vi "MC_8_16_12b_JW.vi"() -> ()   [LabVIEW 2011]
uses:
  <vilib>/Utility/file.llb/Read From Spreadsheet File (string).vi
  <vilib>/Utility/inputDevices.llb/keyboardAcquire.vi
  <vilib>/Utility/file.llb/Write To Spreadsheet File (DBL).vi
  <vilib>/Utility/file.llb/Write To Spreadsheet File (string).vi
  <vilib>/regexp/Match Regular Expression.xnode
panel:
  out "X Axis Display Type":string
  out "Opj X Axis":string
  in  "Room Temp":dbl=294.0
  out "No Image 2":path=path "\\\\acad1\\physics/Jurchescu-group/JW-PD/Image Not Found.png"
  out "Save1 Array":string[][](array[string])
  out "Lin Vd":dbl
  out "Lin-Vg Array-Used":dbl[](array[numeric])
  out "Lin Id-Used":dbl[](array[numeric])
  out "Comments":string
  out "Folder Index":dbl caption="Length"
  out "Current \nRecord":string[](array[string])
  out "Transformer \nHeaders":string[](array[string])
  out "Current Device ID":string
  out "Column":string
  out "Row":string
  out "Rec: Concentration":dbl
  out "Rec: Solvent":string
  out "Rec: Method":string
  in  "?":T1(tab)
  in  "Transport File":path
  out "Transport Folder":path
  out "Rec: Material":string
  in  "Treatment Concentration (mM):":dbl=nan
  in  "Surface Treatment:":string="NaN"
  in  "# Drops*:":dbl=inf
  in  "Solution Temp (C):":dbl=nan
  in  "Relative Humidity (%):":dbl=nan
  in  "Room Temp (F):":dbl=nan
  in  "Time (s):":dbl=nan
  out "Accel (RPM/s):":dbl
  in  "RPM:":dbl=nan
  in  "Wait Time (s):":dbl=nan
  in  "Sample #:":dbl=1.0
  in  "Fabricator:":string="NaN"
  in  "Transfer File":path
  out "Transfer Folder":path
  in  "Image Folder":path
  out "Image File":path=path "D:/UserData/Desktop/Jeremy/WFU/Research/Programs/VI mods/Image Not Found.png"
  in  "Ramp (s):":dbl=3.0
  out "Calc: On/Off":dbl caption="On/Off-Sat" format="%#.2e"
  out "Calc: Off I-Sat":dbl caption="Off I-Sat" format="%#.2e"
  in  "Manuel-Dielectric":bool
  in  "Manuel-Length":bool
  out "Calc: VT-Lin":dbl
  out "New: VT-Lin":dbl
  out "Rec: VT-Lin":dbl caption="VT-Lin" format="%#_3g"
  out "Calc: Trap Density-STS":dbl format="%#.2e"
  out "New: Trap Density-STS":dbl format="%#.2e"
  out "Rec: Trap Density-STS":dbl caption="N-Sat (STS)" format="%#.2e"
  out "Calc: Trap Density-VT":dbl format="%#.2e"
  out "New: Trap Density-VT":dbl format="%#.2e"
  out "Rec: Trap Density-VT":dbl caption="N-Sat (VT)" format="%#.2e"
  out "Calc: Mobility-Lin":dbl format="%#.2e"
  out "New: Mobility-Lin":dbl format="%#_4e"
  out "Rec: Mobility-Lin":dbl caption="Mobility-Lin" format="%#_3e"
  out "Calc: Mobility-Sat":dbl format="%#.2e"
  out "Rec: Length":dbl caption="Length" format="%#_3g"
  out "Rec: Width":dbl caption="Width" format="%#_4g"
  out "Rec: Dielectric (d)":dbl caption="Dielectric (d)" format="%#_3g"
  in  "Cancel Button":bool
  in  "Up Button":bool
  in  "Down Button":bool
  out "Data Name:":string
  in  "Save Changes?":bool
  in  "New: Dielectric":dbl
  in  "New: Length":dbl
  in  "New: Width":dbl
  out "New: Mobility-Sat":dbl format="%#.2e"
  in  "Blank Button":bool
  in  "Zoom":i16(slide)=-3 scale=-5.0..5.0
  out "Image Out 2":T2(plugin-control)
  out "Image Out":T2(plugin-control)
  in  "Magnification":u16(ring) items=["5x", "10x", "20x", "50x", "80x"]
  out "Total Width":dbl
  out "Distances":dbl[](array[numeric])
  in  "Undo Button":bool
  in  "Remove Button":bool
  out "Rec: Mobility-Sat":dbl caption="Mobility-Sat" format="%#.2e"
  out "Index":string
  out "Image Name":string
  in  "Export":bool
  out "Calc: VT-Sat":dbl format="%#.2g"
  out "New: VT-Sat":dbl format="%#.2g"
  in  "Manual-Width":bool caption="Manual"
  out "Calc: STS":dbl format="%#.2g"
  out "New: STS":dbl format="%#.2g"
  out "Rec: VT-Sat":dbl caption="VT-Sat" format="%#.2g"
  out "Rec: STS":dbl caption="STS-Sat" format="%#.2g"
  out "Rec: On/Off":dbl caption="On/Off-Sat" format="%#.2e"
  in  "Save Changes? 2":bool
  in  "Save Changes? 3":bool
  out "Date Recorded":string="Date Recorded" caption="Measured"
  out "Date Created":string caption="Fabricated"
  out "Rec: Temp":dbl caption="Sample Temp" format="%.1f"
  in  "New: Temp":dbl format="%.1f"
  out "Rec: Off I-Sat":dbl caption="Off I-Sat" format="%#.2e"
  in  "Independant Variable":string(combo)="Length (um):"
  in  "Transfer Plots":enum32{"Linear", "Saturation"}(tab)=enum."Saturation"
  out "XY Graph-Lin":cluster{dbl[], dbl[]}[](graph)
  in  "Slide":dbl(slide) step=1.0 scale=-22.0..90.0 scale format="%#_1p"
  out "XY Graph":cluster{dbl[], dbl[]}[](graph)
  in  "Previous Button":bool
  in  "Next Button":bool
  in  "NumPts":dbl=5.0
  in  "Log Plots":enum32{"Linear", "Saturation"}(tab)=enum."Saturation"
  in  "Slide 2":dbl(slide) step=1.0 scale=-1.0..82.0 scale format="%#_1p"
  out "XY Graph 2":cluster{dbl[], dbl[]}[](graph)
  in  "Previous Button 2":bool
  in  "Next Button 2":bool
  in  "NumPts 2":dbl=5.0 caption="NumPts"
  in  "Manual-Temp":bool caption="Manual"
  in  "Origin Project File":path=path "\\\\acad1\\physics/Jurchescu-group/JW-PD/Group Library/Origin Project Files/DeviceData_8_10_12a_JW.opj"
  in  "No Image File":path=path "\\\\acad1\\physics/Jurchescu-group/JW-PD/Mega Awesome/Image Not Found.png"
  out "String":string
  out "Index 2":dbl
  out "Sat Id-Log-Used":dbl[](array[numeric])
  out "Vg Array-Log-Used":dbl[](array[numeric])
  out "ROI Descriptor out":T3 {"Contours"."Type" items=["No Selection", "Point", "Line", "Rectangle", "Oval", "Polygon", "Freehand Region", "Annulus", "Unused2", "Unused3", "Broken Line", "Freehand Line", "Rotated Rectangle"]}
  out "ROI Descriptor":T3 {"Contours"."Type" items=["No Selection", "Point", "Line", "Rectangle", "Oval", "Polygon", "Freehand Region", "Annulus", "Unused2", "Unused3", "Broken Line", "Freehand Line", "Rotated Rectangle"]}
  out "Numeric 3":dbl
  out "Array 6":dbl[][](array[numeric])
  out "Cluster":T4
  out "Array 5":dbl[](array[numeric])
  out "Array 4":dbl[](array[numeric])
  out "Array 3":dbl[](array[numeric])
  out "Numeric 2":dbl
  out "Numeric":dbl
  out "Sat Id-Used":dbl[](array[numeric])
  out "Sat Vg Array-Used":dbl[](array[numeric])
  out "MobVi Index":dbl
  in  "Row Start":dbl=20.0
  # "Data Locations"
  # "Transport Location"
  # "Transfer Location"
  # "Image Location"
  # "Sample Properties"
  # "*     Inf = Full coverage\n   NaN = Unknown or Not Applicable"
  # "Recorded"
  # "Calculated"
  # "Re-Calculated"
  # "Manual"
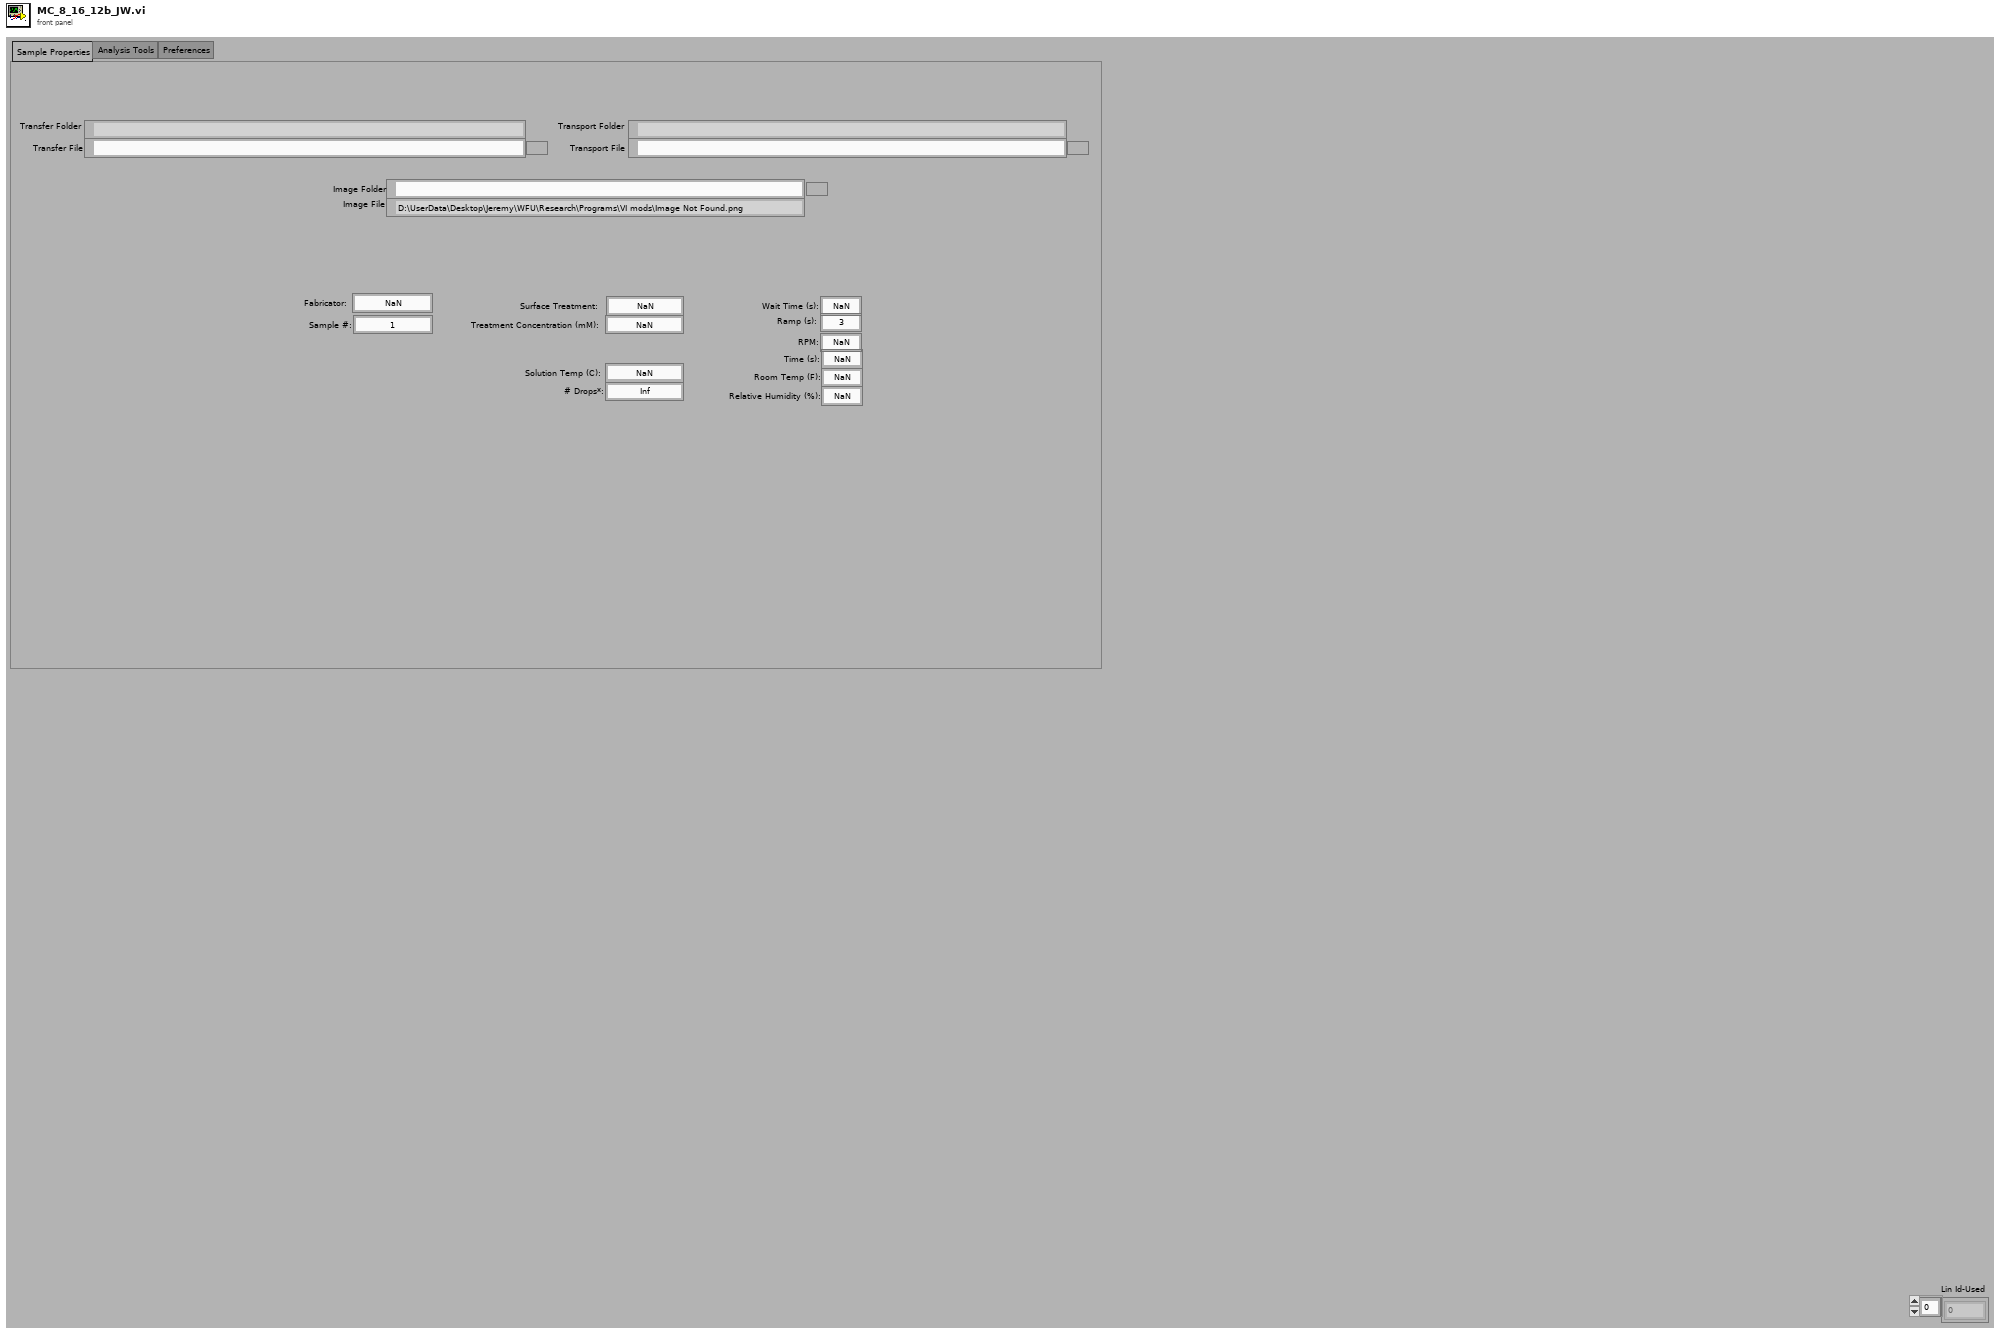
[diagram p1: front panel]
types:
  T1 = enum32{"Sample Properties", "Analysis Tools", "Preferences", "Current Database"}
  T2 = typedef "IMAQ Image.ctl" = refnum<image>
  T3 = typedef "ROI Descriptor" = cluster{"Global Rectangle":i32[], "Contours":cluster{"ID":enum32{"External", "Internal"}, "Type":u32, "Coordinates":i32[]}[]}
  T4 = cluster{"Numeric":dbl, "Numeric 2":dbl, "Numeric 3":dbl, "Numeric 4":dbl}
  T5 = cluster{"Mobility-Sat":dbl, "Moblitity-Lin":dbl, "On/Off":dbl, "Off Current":dbl, "Vt-Sat":dbl, "STS":dbl, "Trap Density-VT":dbl, "Trap Density-STS":dbl}
  T6 = cluster{"Date Recorded":string, "Index":string, "Length":dbl, "Width":dbl, "Sample Temp":dbl}
  T7 = cluster{"Date Created":string, "Material":string, "Solvent":string, "Concentration":dbl, "Method":string, "Dielectric (nm)":dbl, "Treatment":string, "Comments":string}
  T8 = cluster{"Mobility-Sat":dbl, "Vt-Sat":dbl, "Mobility-Lin":dbl, "Vt-Lin":dbl, "Off I-Sat":dbl, "On/Off I-Sat":dbl}
  T9 = cluster{"[0]":cluster{dbl[], dbl[]}, "[1]":cluster{dbl[], dbl[]}, "[2]":cluster{dbl[], dbl[]}, "[3]":cluster{dbl[], dbl[]}, "[4]":cluster{dbl[], dbl[]}, "[5]":cluster{dbl[], dbl[]}, "[6]":cluster{dbl[], dbl[]}, "[7]":cluster{dbl[], dbl[]}, "[8]":cluster{dbl[], dbl[]}}
  T10 = cluster{"Global Rectangle":i32[], "Contours":cluster{"Contour Type":u32, "ROI Type":u32, "Points":i32[]}[]}
  T11 = typedef "LVBoundsTypeDef.ctl" = cluster{"Width":u32, "Height":u32}
  T12 = enum16{"0", "1", "2", "3", "4", "5", "6", "7", "8", "9", "A", "B", "C", "D", "E", "F", "G", "H", "I", "J", "K", "L", "M", "N", "O", "P", "Q", "R", "S", "T", "U", "V", "W", "X", "Y", "Z", "F1", "F2", "F3", "F4", "F5", "F6", "F7", "F8", "F9", "F10", "F11", "F12", "F13", "F14", "F15", "ADD", "BACK", "BACKSLASH", "CAPITAL", "COMMA", "DECIMAL", "DELETE", "DIVIDE", "DOWN", "END", "EQUALS", "ESCAPE", "GRAVE (`)", "HOME", "INSERT", "LBRACKET", "LCONTROL", "LEFT", "L ALT", "LSHIFT", "LWIN", "MINUS", "MULTIPLY", "NEXT", "NUMLOCK", "NUMPAD_0", "NUMPAD_1", "NUMPAD_2", "NUMPAD_3", "NUMPAD_4", "NUMPAD_5", "NUMPAD_6", "NUMPAD_7", "NUMPAD_8", "NUMPAD_9", "PAUSE", "PERIOD", "PRIOR (PG UP)", "RBRACKET", "RCONTROL", "RETURN", "RIGHT", "R ALT", "RSHIFT", "RWIN", "SCROLL", "SEMICOLON", "SLASH", "SPACE", "SUBTRACT", "TAB", "UP", "ENTER (num pad)", "' (quote)"}[]
  T13 = enum16{"0", "1", "2", "3", "4", "5", "6", "7", "8", "9", "A", "B", "C", "D", "E", "F", "G", "H", "I", "J", "K", "L", "M", "N", "O", "P", "Q", "R", "S", "T", "U", "V", "W", "X", "Y", "Z", "F1", "F2", "F3", "F4", "F5", "F6", "F7", "F8", "F9", "F10", "F11", "F12", "F13", "F14", "F15", "ADD", "BACK", "BACKSLASH", "CAPITAL", "COMMA", "DECIMAL", "DELETE", "DIVIDE", "DOWN", "END", "EQUALS", "ESCAPE", "GRAVE (`)", "HOME", "INSERT", "LBRACKET", "LCONTROL", "LEFT", "L ALT", "LSHIFT", "LWIN", "MINUS", "MULTIPLY", "NEXT", "NUMLOCK", "NUMPAD_0", "NUMPAD_1", "NUMPAD_2", "NUMPAD_3", "NUMPAD_4", "NUMPAD_5", "NUMPAD_6", "NUMPAD_7", "NUMPAD_8", "NUMPAD_9", "PAUSE", "PERIOD", "PRIOR (PG UP)", "RBRACKET", "RCONTROL", "RETURN", "RIGHT", "R ALT", "RSHIFT", "RWIN", "SCROLL", "SEMICOLON", "SLASH", "SPACE", "SUBTRACT", "TAB", "UP", "ENTER (num pad)", "' (quote)"}
  T14 = cluster{"Contour Type":u32, "ROI Type":u32, "Points":i32[]}[]
  T15 = cluster{i32[], cluster{"Contour Type":u32, "ROI Type":u32, "Points":i32[]}[]}
  T16 = cluster{"Independant  Variable Indicator":string, "Parameter String Indicator":string}
  T17 = cluster{string, sgl, bool, bool, bool, bool, bool, bool, i32}
  T18 = cluster{i32, cluster{string, sgl, bool, bool, bool, bool, bool, bool, i32}, i32, i32}
  T19 = cluster{"Contour Type":u32, "ROI Type":u32, "Points":i32[]}
  T20 = cluster{"Points[0]":i32, "Points[1]":i32, "Points[2]":i32, "Points[3]":i32, "Points[4]":i32, "Points[5]":i32, "Points[6]":i32, "Points[7]":i32, "Points[8]":i32}
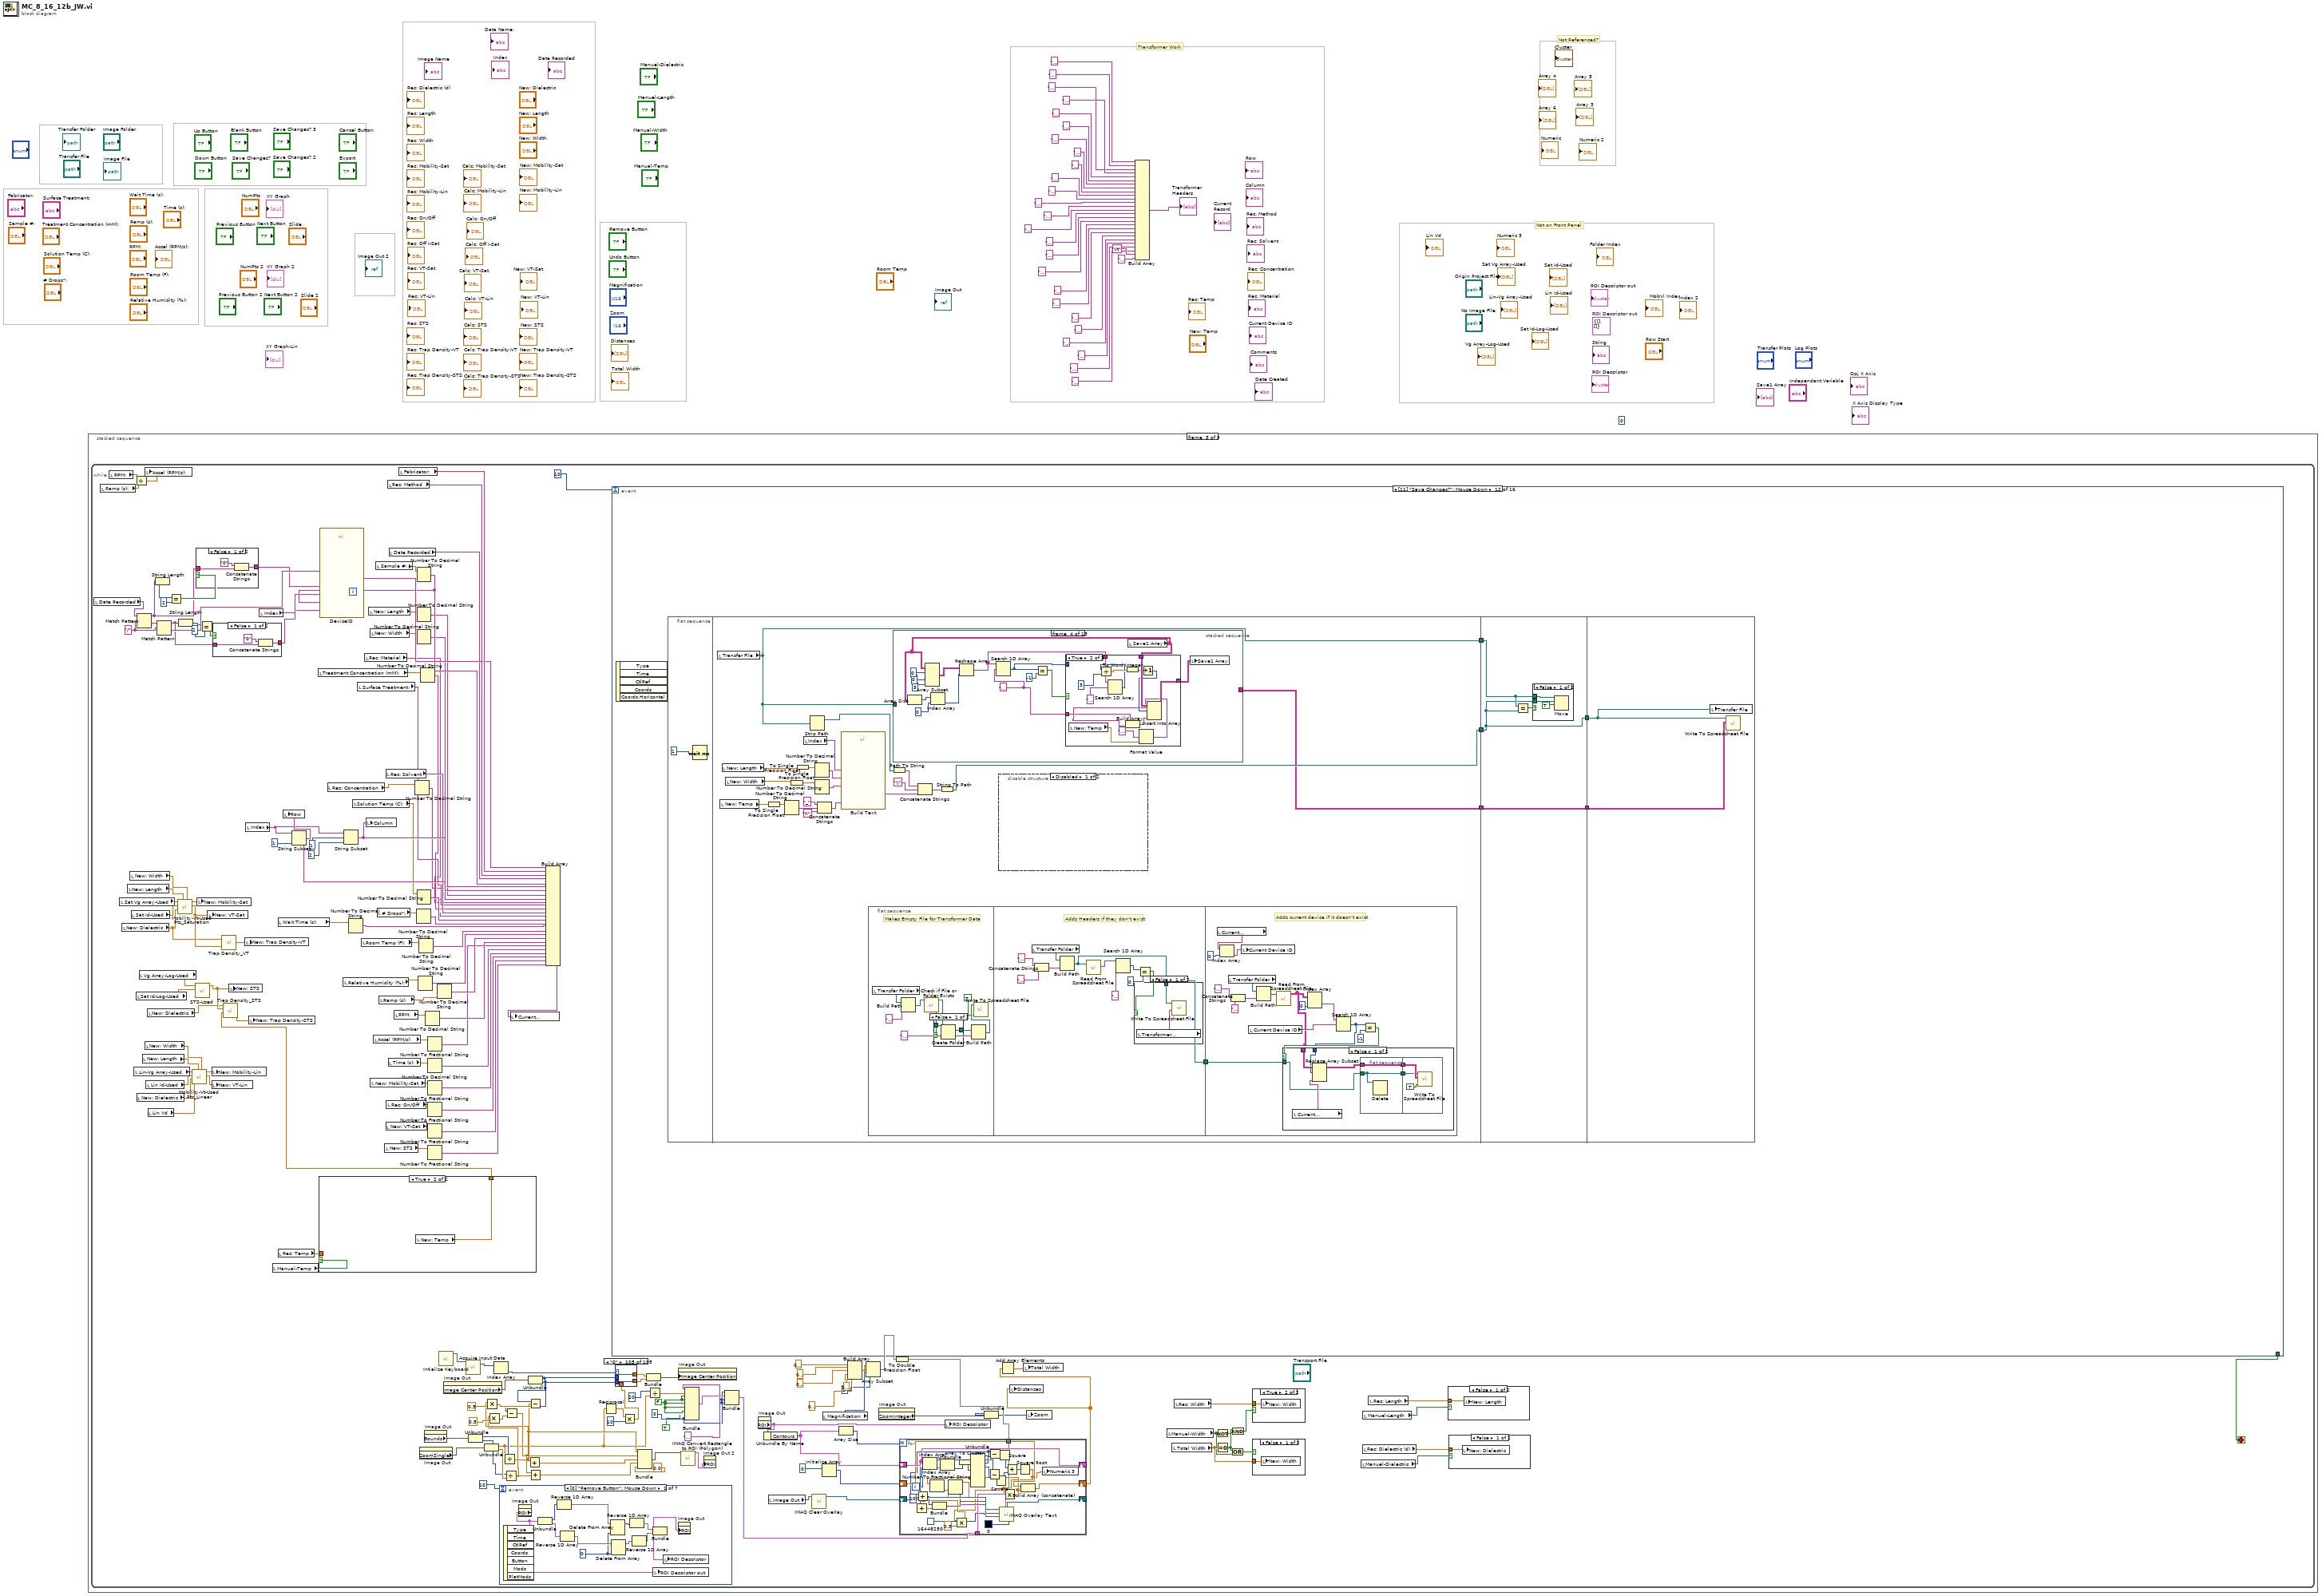
[diagram p0: block diagram]
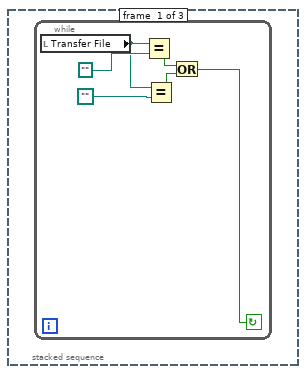
[diagram p2: hidden frame]
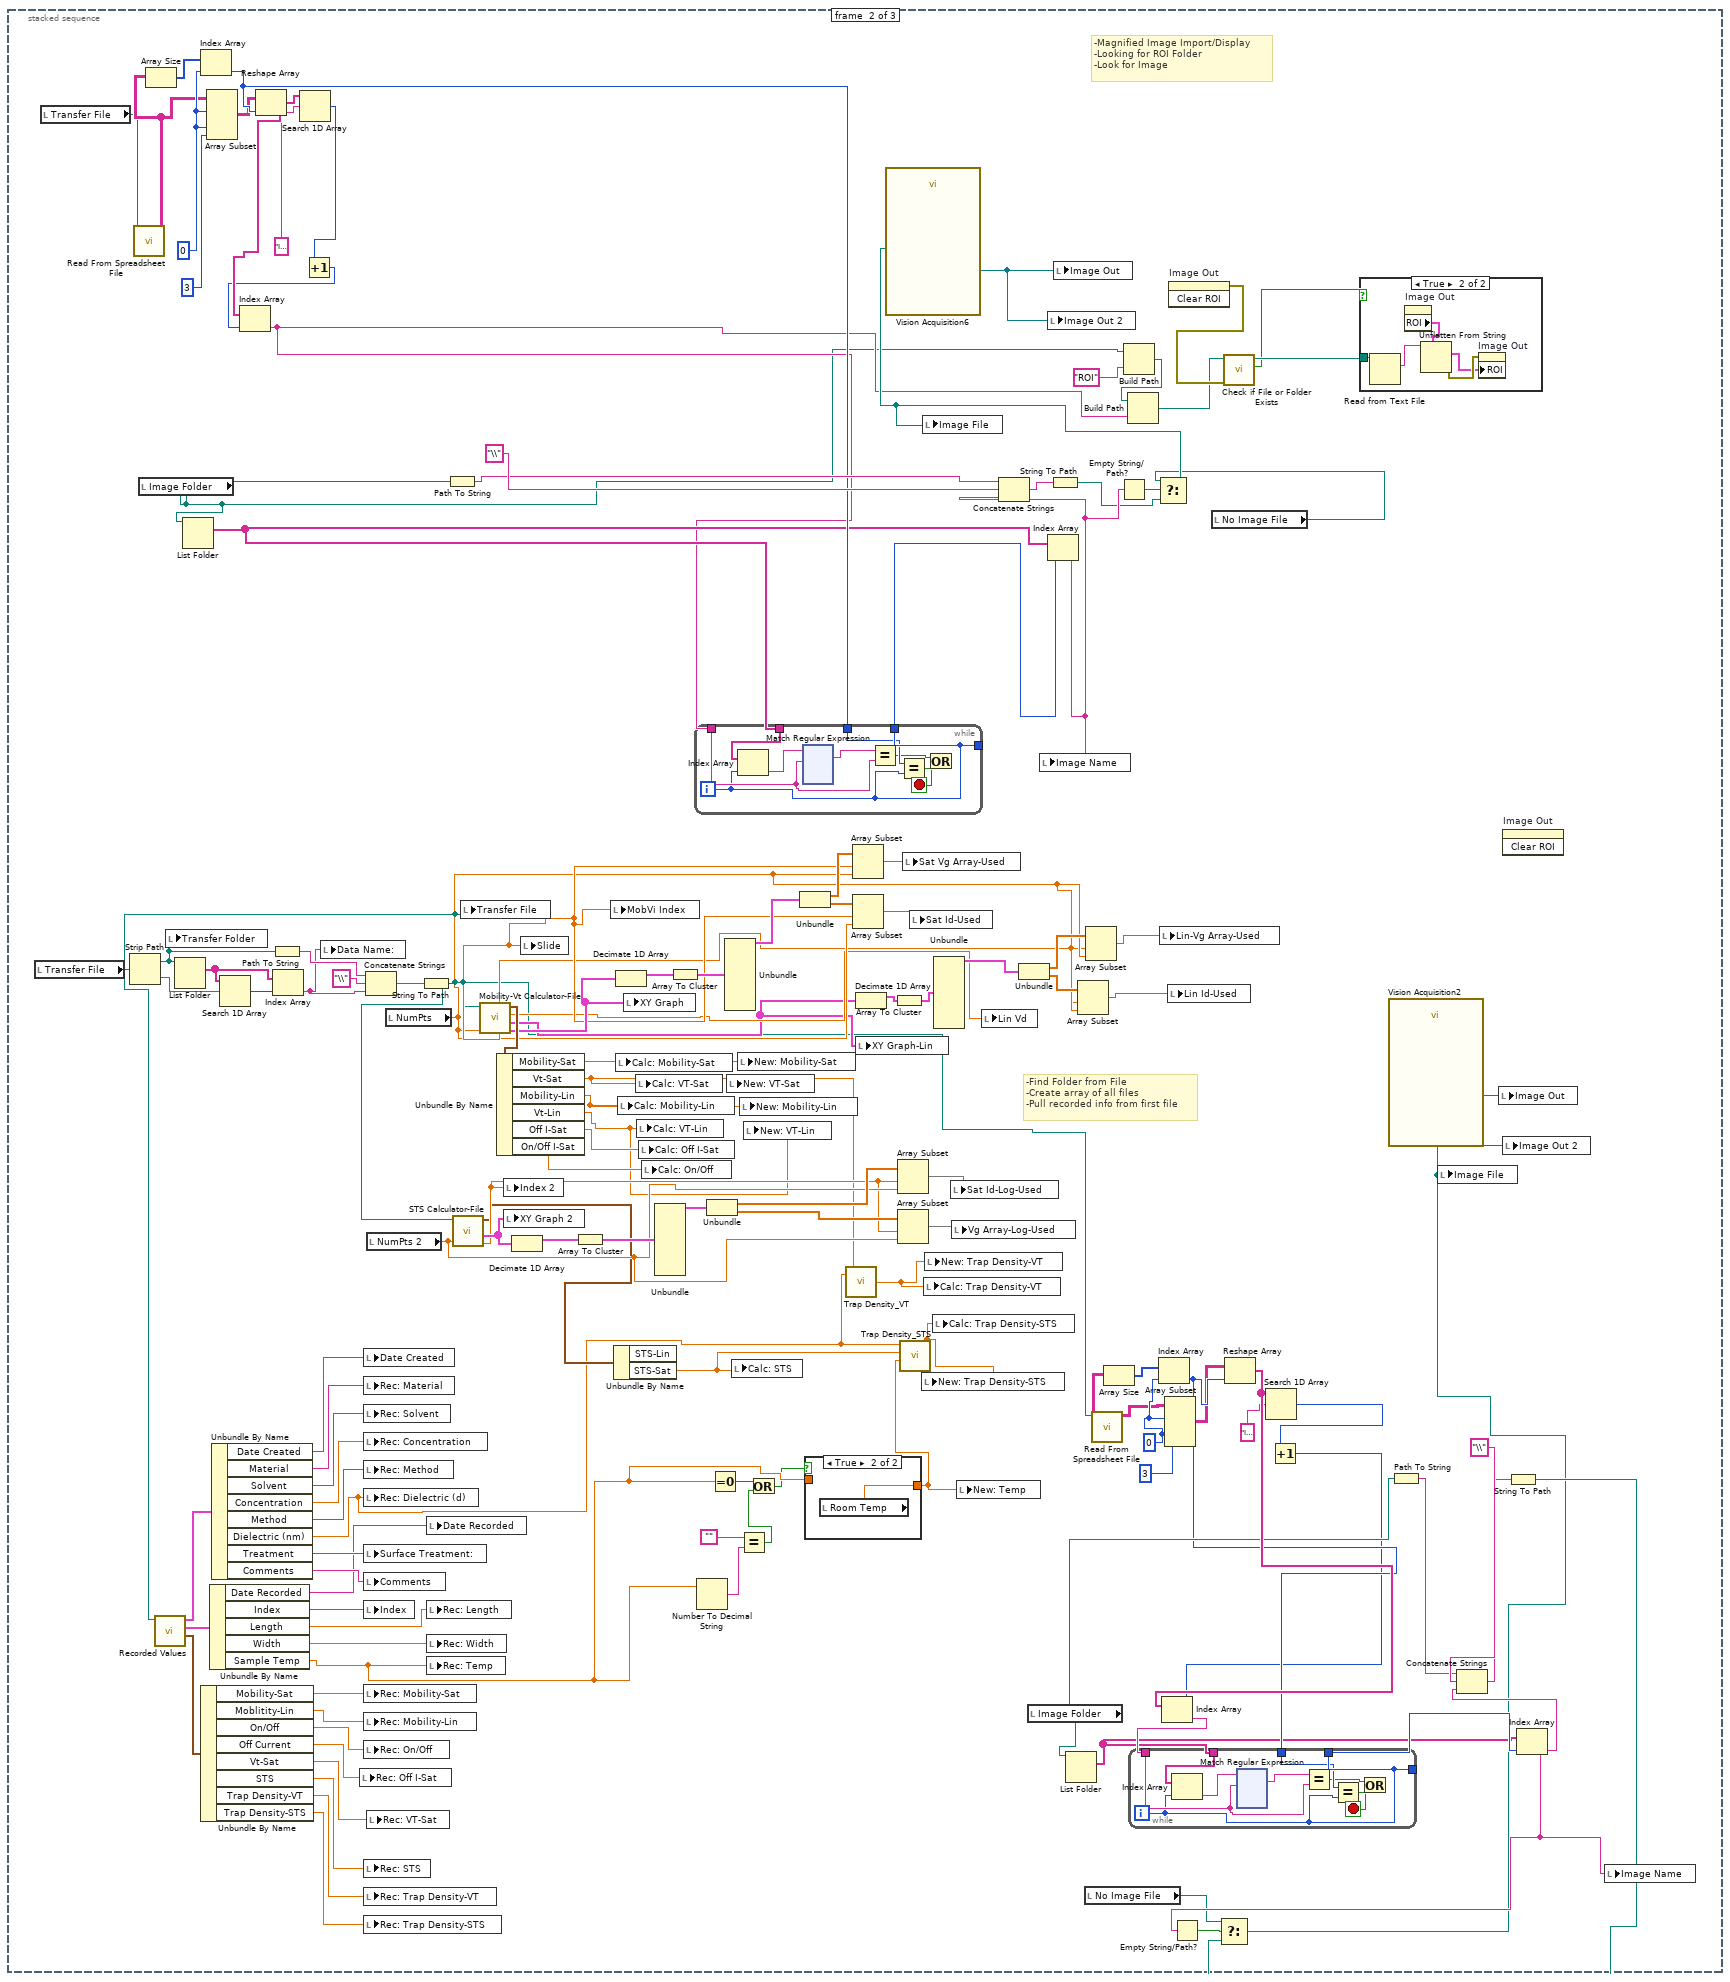
[diagram p3: hidden frame]
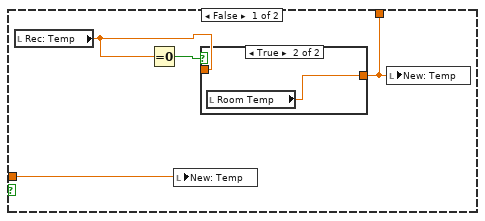
[diagram p6: hidden frame]
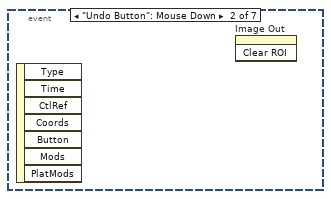
[diagram p14: hidden frame]
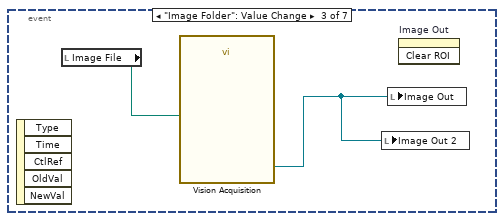
[diagram p15: hidden frame]
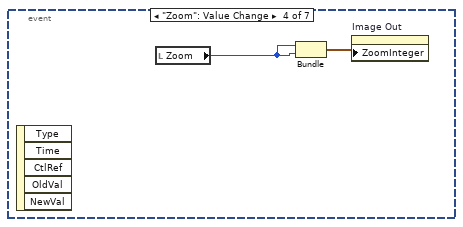
[diagram p16: hidden frame]
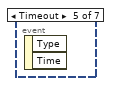
[diagram p17: hidden frame]
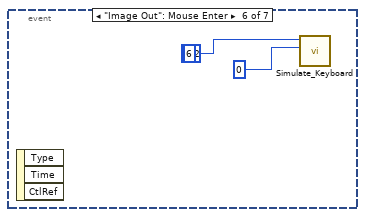
[diagram p18: hidden frame]
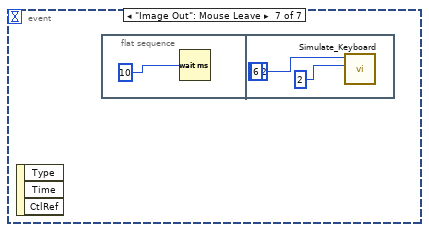
[diagram p19: hidden frame]
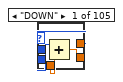
[diagram p20: hidden frame]
diagram:
  (unwired) 0
  (unwired) T3 {"Global Rectangle"=[], "Contours"=[]}  # ROI Descriptor out
  # "Not Referenced?"
  # "Transformer Work"
  # "Not on Front Panel"
  n1 = stacked-sequence {
    frame #0 {
      n2 = while {
        stop <- w29 continue-if-true
        n3 = local read "Transfer File"() -> (w31:path)
        n4 = Equal?(x=w31, y=path "") -> (x = y?=w33:bool)
        n5 = Equal?(x=w31, y=path "") -> (x = y?=w32:bool)
        n6 = Or(x=w33, y=w32) -> (x .or. y?=w29:bool)
      }
    }
    frame #1 {
      w133 = 0
      w157 = 0
      # "-Find Folder from File\n-Create array of all files\n-Pull recorded info from first file"
      # "-Magnified Image Import/Display\n-Looking for ROI Folder\n-Look for Image"
      n7 = local read "Transfer File"() -> (w137:path)
      n8 = local read "Transfer File"() -> (w152:path)
      n9 = Strip Path(path=w137) -> (stripped path=w138:path, name=w124:string)
      n10 = call-poly <vilib>:"Read From Spreadsheet File.vi"("file path (dialog if empty)"=w152) -> ("all rows"=w155:string[][])  [unwired: 6 in, 4 out]
      n11 = local read "Image Folder"() -> (w94:path)
      n12 = Array Size(array=w155) -> (size(s)=w156:i32[])
      n13 = local write "Transfer Folder"(w138) -> ()
      n14 = List Folder(path=w138) -> (filenames=w128:string[])  [unwired: 3 in, 3 out]
      n15 = List Folder(path=w94) -> (filenames=w161:string[])  [unwired: 3 in, 3 out]
      n16 = Index Array(array=w156, index=w157) -> (element=w163:i32)
      n17 = Array Subset(array=w155, index (row)=w157, index (col)=w157, length (col)=3) -> (w154:string[][])  [unwired: 1 in]
      n18 = Search 1D Array(1D array=w128, element=w124) -> (index of element=w127:i32)  [unwired: 1 in]
      n19 = Reshape Array(w154, w163) -> (w168:string[])
      n20 = Path To String(path=w138) -> (string=w123:string)
      n21 = Index Array(array=w128, index=w127) -> (element=w93:string)
      n22 = Search 1D Array(1D array=w168, element="Index:") -> (index of element=w160:i32)  [unwired: 1 in]
      n23 = Increment(x=w160) -> (x+1=w159:i32)
      n24 = Index Array(array=w168, index=w159) -> (element=w95:string)
      n25 = local write "Data Name:"(w93) -> ()
      n26 = Concatenate Strings(w123, "\\", w93) -> (w125:string)
      n27 = local read "NumPts 2"() -> (w68:dbl)
      n28 = local read "NumPts"() -> (w59:dbl)
      n29 = String To Path(string=w125) -> (path=w52:path)
      n30 = call "Recorded Values.vi"("Path"=w52) -> ("Recorded Char"=w91:T5, "Recorded Prop"=w90:T6, "Fabrication Prop"=w92:T7)  [unwired: 8 in]
      n31 = Unbundle By Name(w91) -> ("Mobility-Sat"=w79:dbl, "Moblitity-Lin"=w78:dbl, "On/Off"=w77:dbl, "Off Current"=w76:dbl, "Vt-Sat"=w38:dbl, "STS"=w75:dbl, "Trap Density-VT"=w74:dbl, "Trap Density-STS"=w73:dbl)
      n32 = Unbundle By Name(w90) -> ("Date Recorded"=w83:string, "Index"=w82:string, "Length"=w81:dbl, "Width"=w80:dbl, "Sample Temp"=w44:dbl)
      n33 = Unbundle By Name(w92) -> ("Date Created"=w72:string, "Material"=w89:string, "Solvent"=w88:string, "Concentration"=w87:dbl, "Method"=w86:string, "Dielectric (nm)"=w48:dbl, "Treatment"=w85:string, "Comments"=w84:string)
      n34 = local write "Rec: Off I-Sat"(w76) -> ()
      n35 = local write "Date Created"(w72) -> ()
      n36 = local write "Rec: Material"(w89) -> ()
      n37 = local write "Rec: Solvent"(w88) -> ()
      n38 = local write "Rec: Concentration"(w87) -> ()
      n39 = local write "Rec: Method"(w86) -> ()
      n40 = local write "Rec: Dielectric (d)"(w48) -> ()
      n41 = local write "Surface Treatment:"(w85) -> ()
      n42 = local write "Comments"(w84) -> ()
      n43 = local write "Index"(w82) -> ()
      n44 = local write "Rec: Mobility-Sat"(w79) -> ()
      n45 = local write "Rec: Mobility-Lin"(w78) -> ()
      n46 = local write "Rec: On/Off"(w77) -> ()
      n47 = local write "Rec: STS"(w75) -> ()
      n48 = local write "Rec: Trap Density-VT"(w74) -> ()
      n49 = local write "Rec: Trap Density-STS"(w73) -> ()
      n50 = local write "Rec: VT-Sat"(w38) -> ()
      n51 = local write "Date Recorded"(w83) -> ()
      n52 = local write "Rec: Length"(w81) -> ()
      n53 = local write "Rec: Width"(w80) -> ()
      n54 = local write "Rec: Temp"(w44) -> ()
      n55 = Path To String(path=w94) -> (string=w165:string)
      n56 = call "STS Calculator-File.vi"("NumPts"=w68, "Path"=w52) -> ("STS Index-Sat"=w66:dbl, "XY Graph-Sat"=w67:cluster{dbl[], dbl[]}[], "Ouput"=w65:cluster{"STS-Sat":dbl, "STS-Lin":dbl})  [unwired: 5 in, 2 out]
      n57 = local write "Transfer File"(w52) -> ()
      n58 = call "Mobility-Vt Calculator-File.vi"("NumPts"=w59, "Path"=w52) -> ("XY Graph-Sat"=w70:cluster{dbl[], dbl[]}[], "XY Graph-Lin"=w54:cluster{dbl[], dbl[]}[], "Lin Vd"=w55:dbl, "Output"=w71:T8, "Index-Sat"=w69:dbl, "Index-Lin"=w58:dbl)  [unwired: 4 in]
      n59 = Unbundle By Name(w71) -> ("Mobility-Sat"=w47:dbl, "Vt-Sat"=w46:dbl, "Mobility-Lin"=w37:dbl, "Vt-Lin"=w35:dbl, "Off I-Sat"=w53:dbl, "On/Off I-Sat"=w36:dbl)
      n60 = local write "Index 2"(w66) -> ()
      n61 = local write "XY Graph 2"(w67) -> ()
      n62 = Decimate 1D Array(w67) -> (w115:cluster{dbl[], dbl[]}[])  [unwired: 1 out]
      n63 = local write "Slide"(w69) -> ()
      n64 = Array To Cluster(array=w115) -> (cluster=w117:T9)
      n65 = local write "MobVi Index"(w69) -> ()
      n66 = Unbundle By Name(w65) -> ("STS-Sat"=w51:dbl)  [unwired: 1 out]
      n67 = Decimate 1D Array(w70) -> (w151:cluster{dbl[], dbl[]}[])  [unwired: 1 out]
      n68 = local write "Calc: Mobility-Sat"(w47) -> ()
      n69 = local write "Calc: Mobility-Lin"(w37) -> ()
      n70 = local write "XY Graph"(w70) -> ()
      n71 = local write "Calc: VT-Sat"(w46) -> ()
      n72 = local write "Calc: VT-Lin"(w35) -> ()
      n73 = local write "Calc: Off I-Sat"(w53) -> ()
      n74 = local write "Calc: On/Off"(w36) -> ()
      n75 = Unbundle(w117) -> ("[0]"=w116:cluster{dbl[], dbl[]})  [unwired: 8 out]
      n76 = Array To Cluster(array=w151) -> (cluster=w149:T9)
      n77 = while {
        tunnel: w161 -> [w303]
        tunnel: w95 -> [w301]
        tunnel: [w300] -> _
        tunnel: [w300] -> w162
        tunnel: w163 -> [w299]
        i -> [w300]
        stop <- w296 stop-if-true
        n78 = Index Array(array=w303, index=w300) -> (element=w304:string)
        n79 = xnode "Match Regular Expression"("input string"=w304, "regular expression"=w301) -> ("whole match"=w302:string)  [unwired: 4 in, 4 out]
        n80 = Equal?(x=w302, y=w301) -> (x = y?=w298:bool)
        n81 = Equal?(x=w299, y=w300) -> (x = y?=w297:bool)
        n82 = Or(x=w298, y=w297) -> (x .or. y?=w296:bool)
      }
      n83 = Number To Decimal String(number=w44) -> (decimal integer string=w42:string)  [unwired: 1 in]
      n84 = Unbundle(w116) -> (w113:dbl[], w112:dbl[])
      n85 = Equal To 0?(x=w44) -> (x = 0?=w43:bool)
      n86 = Unbundle(w149) -> ("[0]"=w150:cluster{dbl[], dbl[]})  [unwired: 8 out]
      n87 = local write "New: VT-Sat"(w46) -> ()
      n88 = local write "Calc: STS"(w51) -> ()
      n89 = local write "New: Mobility-Sat"(w47) -> ()
      n90 = Equal?(x="", y=w42) -> (x = y?=w40:bool)
      n91 = local write "New: Mobility-Lin"(w37) -> ()
      n92 = local write "New: VT-Lin"(w35) -> ()
      n93 = Or(x=w43, y=w40) -> (x .or. y?=w39:bool)
      n94 = Unbundle(w150) -> (w114:dbl[], w118:dbl[])
      n95 = case shown="True" w39 {
        tunnel: [w169 w170] -> w50
        tunnel: w44 -> [w169 _]
        frame False {
        }
        frame True {
          n96 = local read "Room Temp"() -> (w170:dbl)
        }
      }
      n97 = call "Trap Density_VT.vi"("VT"=w46, "Dielectric"=w48) -> ("Trap Density-VT"=w45:dbl)
      n98 = Array Subset(array=w114, index=w69, length=w59) -> (w121:dbl[])
      n99 = Array Subset(array=w118, index=w69, length=w59) -> (w122:dbl[])
      n100 = Decimate 1D Array(w54) -> (w64:cluster{dbl[], dbl[]}[])  [unwired: 1 out]
      n101 = local write "XY Graph-Lin"(w54) -> ()
      n102 = Array To Cluster(array=w64) -> (cluster=w63:T9)
      n103 = Array Subset(array=w113, index=w66, length=w68) -> (w120:dbl[])
      n104 = Array Subset(array=w112, index=w66, length=w68) -> (w119:dbl[])
      n105 = call "Trap Density_STS.vi"("Temp (T) [K]"=w50, "S.T.S. (S)"=w51, "Dielectric"=w48) -> ("Trap Density (N)"=w49:dbl)  [unwired: 8 in]
      n106 = local write "Sat Vg Array-Used"(w121) -> ()
      n107 = local write "Sat Id-Used"(w122) -> ()
      n108 = local write "New: Trap Density-STS"(w49) -> ()
      n109 = local write "Calc: Trap Density-VT"(w45) -> ()
      n110 = local write "New: Trap Density-VT"(w45) -> ()
      n111 = local write "Calc: Trap Density-STS"(w49) -> ()
      n112 = Unbundle(w63) -> ("[0]"=w62:cluster{dbl[], dbl[]})  [unwired: 8 out]
      n113 = local write "Sat Id-Log-Used"(w120) -> ()
      n114 = local write "Vg Array-Log-Used"(w119) -> ()
      n115 = local write "New: Temp"(w50) -> ()
      n116 = local write "Lin Vd"(w55) -> ()
      n117 = Unbundle(w62) -> (w61:dbl[], w60:dbl[])
      n118 = local read "Image Folder"() -> (w144:path)
      n119 = Index Array(array=w161, index=w162) -> (element=w111:string)
      n120 = Concatenate Strings(w165, "\\", w111) -> (w166:string)
      n121 = local write "Image Name"(w111) -> ()
      n122 = String To Path(string=w166) -> (path=w109:path)
      n123 = List Folder(path=w144) -> (filenames=w140:string[])  [unwired: 3 in, 3 out]
      n124 = Array Subset(array=w60, index=w58, length=w59) -> (w56:dbl[])
      n125 = local read "No Image File"() -> (w103:path)
      n126 = Array Subset(array=w61, index=w58, length=w59) -> (w57:dbl[])
      n127 = call-poly <vilib>:"Read From Spreadsheet File.vi"("file path (dialog if empty)"=w52) -> ("all rows"=w131:string[][])  [unwired: 6 in, 4 out]
      n128 = Array Size(array=w131) -> (size(s)=w132:i32[])
      n129 = Empty String/Path?(string/path=w111) -> (empty?=w110:bool)
      n130 = Build Path(base path=w94, name or relative path="ROI") -> (appended path=w97:path)
      n131 = Build Path(base path=w97, name or relative path=w95) -> (appended path=w96:path)
      n132 = Index Array(array=w132, index=w133) -> (element=w143:i32)
      n133 = local write "Lin-Vg Array-Used"(w57) -> ()
      n134 = Array Subset(array=w131, index (row)=w133, index (col)=w133, length (col)=3) -> (w130:string[][])  [unwired: 1 in]
      n135 = local write "Lin Id-Used"(w56) -> ()
      n136 = invoke on="Image Out" class="ImageControl" method="Clear ROI"() -> (error out=w101:errorcluster)  [unwired: 3 in, 2 out]
      n137 = local read "No Image File"() -> (w102:path)
      n138 = Select(t=w102, s=w110, f=w109) -> (s? t:f=w108:path)
      n139 = call "Vision Acquisition6"("Image Path"=w108) -> ("Image Out"=w164:T2)  [unwired: 25 in, 1 out]
      n140 = local write "Image File"(w108) -> ()
      n141 = local write "Image Out 2"(w164) -> ()
      n142 = local write "Image Out"(w164) -> ()
      n143 = call <vilib>:"Check if File or Folder Exists.vi"("error in (no error)"=w101, "path"=w96) -> ("file or folder exists?"=w99:bool, "dup path"=w100:path)  [unwired: 7 in, 1 out]
      n144 = Reshape Array(w130, w143) -> (w148:string[])
      n145 = Search 1D Array(1D array=w148, element="Index:") -> (index of element=w136:i32)  [unwired: 1 in]
      n146 = Increment(x=w136) -> (x+1=w135:i32)
      n147 = Index Array(array=w148, index=w135) -> (element=w141:string)
      n148 = while {
        tunnel: w140 -> [w183]
        tunnel: w141 -> [w181]
        tunnel: [w180] -> _
        tunnel: [w180] -> w142
        tunnel: w143 -> [w179]
        i -> [w180]
        stop <- w176 stop-if-true
        n149 = Index Array(array=w183, index=w180) -> (element=w184:string)
        n150 = xnode "Match Regular Expression"("input string"=w184, "regular expression"=w181) -> ("whole match"=w182:string)  [unwired: 4 in, 4 out]
        n151 = Equal?(x=w182, y=w181) -> (x = y?=w178:bool)
        n152 = Equal?(x=w179, y=w180) -> (x = y?=w177:bool)
        n153 = Or(x=w178, y=w177) -> (x .or. y?=w176:bool)
      }
      n154 = case shown="True" w99 {
        tunnel: w100 -> [_ w171]
        frame False {
        }
        frame True {
          n155 = Read from Text File(file (use dialog)=w171) -> (text=w175:string)  [unwired: 3 in, 3 out]
          n156 = property on="Image Out" class="ImageControl"() -> ("ROI"=w172:T10)  [unwired: 2 in, 2 out]
          n157 = Unflatten From String(type=w172, binary string=w175) -> (value=w173:T10, error out=w174:errorcluster)  [unwired: 3 in, 1 out]
          n158 = property on="Image Out" class="ImageControl"(error in=w174, "ROI"=w173) -> ()  [unwired: 1 in, 2 out]
        }
      }
      n159 = Path To String(path=w144) -> (string=w145:string)
      n160 = invoke on="Image Out" class="ImageControl" method="Clear ROI"() -> ()  [unwired: 3 in, 3 out]
      n161 = Index Array(array=w140, index=w142) -> (element=w106:string)
      n162 = Empty String/Path?(string/path=w106) -> (empty?=w107:bool)
      n163 = Concatenate Strings(w145, "\\", w106) -> (w146:string)
      n164 = String To Path(string=w146) -> (path=w105:path)
      n165 = Select(t=w103, s=w107, f=w105) -> (s? t:f=w104:path)
      n166 = call "Vision Acquisition2"("Image Path"=w104) -> ("Image Out"=w139:T2)  [unwired: 25 in, 1 out]
      n167 = local write "Image File"(w104) -> ()
      n168 = local write "Image Out"(w139) -> ()
      n169 = local write "Image Out 2"(w139) -> ()
      n170 = local write "Image Name"(w106) -> ()
    }
    frame #2 {
      n171 = while {
        stop <- w581 stop-if-true
        w477 = "/"
        w531 = FALSE
        w529 = 0
        n172 = local read "Date Recorded"() -> (w480:string)
        n173 = local read "Ramp (s):"() -> (w447:dbl)
        n174 = local read "RPM:"() -> (w448:dbl)
        n175 = local read "Sat Vg Array-Used"() -> (w436:dbl[])
        n176 = local read "New: Dielectric"() -> (w421:dbl)
        n177 = local read "New: Length"() -> (w437:dbl)
        n178 = local read "New: Width"() -> (w439:dbl)
        n179 = local read "Sat Id-Used"() -> (w435:dbl[])
        n180 = local read "Lin-Vg Array-Used"() -> (w430:dbl[])
        n181 = Divide(x=w448, y=w447) -> (x/y=w446:dbl)
        n182 = local read "Sat Id-Log-Used"() -> (w434:dbl[])
        n183 = local read "New: Dielectric"() -> (w427:dbl)
        n184 = Match Pattern(string=w480, regular expression=w477) -> (before substring=w471:string, after substring=w478:string)  [unwired: 1 in, 2 out]
        n185 = local read "Vg Array-Log-Used"() -> (w433:dbl[])
        n186 = local read "New: Length"() -> (w429:dbl)
        n187 = local write "Accel (RPM/s):"(w446) -> ()
        n188 = local read "New: Width"() -> (w426:dbl)
        n189 = local read "Lin Id-Used"() -> (w431:dbl[])
        n190 = local read "New: Dielectric"() -> (w423:dbl)
        n191 = local read "Lin Vd"() -> (w425:dbl)
        n192 = String Length(string=w471) -> (length=w474:i32)
        n193 = Match Pattern(string=w478, regular expression=w477) -> (before substring=w465:string, after substring=w476:string)  [unwired: 1 in, 2 out]
        n194 = Equal?(x=w474, y=2) -> (x = y?=w472:bool)
        n195 = call "Mobility-Vt-Used Pts_Saturation.vi"("Width"=w439, "Length"=w437, "Dielectric (d)"=w421, "Sat Id Used"=w435, "Vg Used"=w436) -> ("Vt"=w422:dbl, "Mobility"=w438:dbl)  [unwired: 4 in, 1 out]
        n196 = String Length(string=w465) -> (length=w467:i32)
        n197 = call "Mobility-Vt-Used Pts_Linear.vi"("Width"=w426, "Length"=w429, "Vd"=w425, "Dielectric (d)"=w427, "Sat Id Used"=w431, "Vg Used"=w430) -> ("Vt"=w432:dbl, "Mobility"=w428:dbl)  [unwired: 3 in, 1 out]
        n198 = call "STS-Used.vi"("Id Used"=w434, "Vg-Used"=w433) -> ("STS"=w424:dbl)  [unwired: 9 in]
        n199 = case shown="False" w472 {
          tunnel: w471 -> [w596 w598]
          tunnel: [w595 w598] -> w470
          frame False {
            n200 = Concatenate Strings("0", w596) -> (w595:string)
          }
          frame True {
          }
        }
        n201 = local write "New: Mobility-Sat"(w438) -> ()
        n202 = Equal?(x=w467, y=2) -> (x = y?=w469:bool)
        n203 = local write "New: VT-Sat"(w422) -> ()
        n204 = local write "New: Mobility-Lin"(w428) -> ()
        n205 = local write "New: VT-Lin"(w432) -> ()
        n206 = case shown="False" w469 {
          tunnel: w465 -> [w592 w594]
          tunnel: [w591 w594] -> w466
          frame False {
            n207 = Concatenate Strings("0", w592) -> (w591:string)
          }
          frame True {
          }
        }
        n208 = call "Trap Density_VT.vi"("VT"=w422, "Dielectric"=w421) -> ("Trap Density-VT"=w420:dbl)
        n209 = local write "New: STS"(w424) -> ()
        n210 = local write "New: Trap Density-VT"(w420) -> ()
        n211 = local read "Index"() -> (w450:string)
        n212 = local read "Index"() -> (w464:string)
        n213 = local read "Manual-Temp"() -> (w417:bool)
        n214 = local read "Wait Time (s):"() -> (w510:dbl)
        n215 = local read "Rec: Temp"() -> (w418:dbl)
        n216 = String Subset(string=w450, length (rest)=1) -> (substring=w505:string)  [unwired: 1 in]
        n217 = local write "Row"(w505) -> ()
        n218 = local read "Treatment Concentration (mM):"() -> (w458:dbl)
        n219 = case shown="True" w417 {
          tunnel: w418 -> [w585 _]
          tunnel: [w582 w588] -> w416
          frame False {
            n220 = local read "Rec: Temp"() -> (w583:dbl)
            n221 = Equal To 0?(x=w583) -> (x = 0?=w584:bool)
            n222 = local write "New: Temp"(w585) -> ()
            n223 = case shown="True" w584 {
              tunnel: [w586 w587] -> w582
              tunnel: w583 -> [w586 _]
              frame False {
              }
              frame True {
                n224 = local read "Room Temp"() -> (w587:dbl)
              }
            }
            n225 = local write "New: Temp"(w582) -> ()
          }
          frame True {
            n226 = local read "New: Temp"() -> (w588:dbl)
          }
        }
        n227 = call "Trap Density_STS.vi"("Temp (T) [K]"=w416, "S.T.S. (S)"=w424, "Dielectric"=w423) -> ("Trap Density (N)"=w419:dbl)  [unwired: 8 in]
        n228 = local write "New: Trap Density-STS"(w419) -> ()
        n229 = local read "Rec: Concentration"() -> (w445:dbl)
        n230 = local read "Relative Humidity (%):"() -> (w455:dbl)
        n231 = String Subset(string=w450, offset (0)=1, length (rest)=2) -> (substring=w506:string)
        n232 = Number To Decimal String(number=w510) -> (decimal integer string=w511:string)  [unwired: 1 in]
        n233 = local read "Solution Temp (C):"() -> (w499:dbl)
        n234 = local read "Surface Treatment:"() -> (w457:string)
        n235 = local read "Room Temp (F):"() -> (w503:dbl)
        n236 = local read "Rec: Material"() -> (w453:string)
        n237 = local write "Column"(w506) -> ()
        n238 = local read "New: Length"() -> (w463:dbl)
        n239 = local read "New: Width"() -> (w462:dbl)
        n240 = local read "New: Mobility-Sat"() -> (w492:dbl)
        n241 = local read "Accel (RPM/s):"() -> (w490:dbl)
        n242 = local read "Sample #:"() -> (w482:dbl)
        n243 = local read "# Drops*:"() -> (w500:dbl)
        n244 = local read "Ramp (s):"() -> (w508:dbl)
        n245 = local read "New: STS"() -> (w484:dbl)
        n246 = local read "Rec: Solvent"() -> (w459:string)
        n247 = local read "New: VT-Sat"() -> (w486:dbl)
        n248 = local read "Rec: On/Off"() -> (w488:dbl)
        n249 = local read "Rec: Method"() -> (w483:string)
        n250 = local read "Time (s):"() -> (w495:dbl)
        n251 = local read "Date Recorded"() -> (w479:string)
        n252 = local read "RPM:"() -> (w496:dbl)
        n253 = local read "Fabricator:"() -> (w504:string)
        n254 = Number To Decimal String(number=w445) -> (decimal integer string=w444:string)  [unwired: 1 in]
        n255 = Number To Decimal String(number=w500) -> (decimal integer string=w501:string)  [unwired: 1 in]
        n256 = Number To Decimal String(number=w482) -> (decimal integer string=w475:string)  [unwired: 1 in]
        n257 = call "DeviceID"("Sample"=w475, "Year"=w476, "Month"=w470, "Day"=w466, "Index"=w464) -> ("Result"=w481:string)  [unwired: 9 in, 1 out]
        n258 = Number To Decimal String(number=w463) -> (decimal integer string=w461:string)  [unwired: 1 in]
        n259 = Number To Decimal String(number=w462) -> (decimal integer string=w460:string)  [unwired: 1 in]
        n260 = Number To Decimal String(number=w499) -> (decimal integer string=w498:string)  [unwired: 1 in]
        n261 = Number To Decimal String(number=w455) -> (decimal integer string=w454:string)  [unwired: 1 in]
        n262 = Number To Decimal String(number=w503) -> (decimal integer string=w502:string)  [unwired: 1 in]
        n263 = property on="Image Out" class="ImageControl"() -> ("ZoomSingle"=w549:cluster{"X":sgl, "Y":sgl})  [unwired: 2 in, 2 out]
        n264 = Number To Decimal String(number=w458) -> (decimal integer string=w456:string)  [unwired: 1 in]
        n265 = property on="Image Out" class="ImageControl"() -> ("Bounds"=w550:T11)  [unwired: 2 in, 2 out]
        n266 = Number To Decimal String(number=w496) -> (decimal integer string=w497:string)  [unwired: 1 in]
        n267 = Number To Fractional String(number=w490) -> (F-format string=w491:string)  [unwired: 3 in]
        n268 = Number To Decimal String(number=w495) -> (decimal integer string=w494:string)  [unwired: 1 in]
        n269 = Number To Fractional String(number=w492) -> (F-format string=w493:string)  [unwired: 3 in]
        n270 = Number To Fractional String(number=w488) -> (F-format string=w489:string)  [unwired: 3 in]
        n271 = Number To Fractional String(number=w486) -> (F-format string=w487:string)  [unwired: 3 in]
        n272 = Number To Fractional String(number=w484) -> (F-format string=w485:string)  [unwired: 3 in]
        n273 = Number To Decimal String(number=w508) -> (decimal integer string=w509:string)  [unwired: 1 in]
        n274 = call <vilib>:"Intialize Keyboard.vi"() -> ("device ID"=w561:refnum<k1>)  [unwired: 10 in, 1 out]
        n275 = property on="Image Out" class="ImageControl"() -> ("Image Center Position"=w556:cluster{"X":u32, "Y":u32})  [unwired: 2 in, 2 out]
        n276 = call-poly <vilib>:"Acquire Input Data.vi"("device ID"=w561) -> ("keys pressed"=w560:T12)  [unwired: 16 in, 2 out]
        n277 = Unbundle(w550) -> ("Width"=w547:u32, "Height"=w546:u32)
        n278 = Unbundle(w549) -> ("X"=w524:sgl, "Y"=w548:sgl)
        n279 = Index Array(array=w560) -> (element=w564:T13)  [unwired: 1 in]
        n280 = event shown="[0] \"Remove Button\": Mouse Down" {
          selector: _ -> [_ _ _ _ _ _ _]
          dyn-events: _ -> [_ _ _ _ _ _ _]
          timeout: 10 -> [_ _ _ _ _ _ _]
          event "Remove Button": Mouse Down {
            w603 = 0
            n281 = event-data() -> ()  [unwired: 1 in, 7 out]
            n282 = property on="Image Out" class="ImageControl"() -> ("ROI"=w601:T10)  [unwired: 2 in, 2 out]
            n283 = Unbundle(w601) -> ("Global Rectangle"=w604:i32[], "Contours"=w606:T14)
            n284 = Reverse 1D Array(array=w604) -> (reversed array=w605:i32[])
            n285 = Reverse 1D Array(array=w606) -> (reversed array=w607:T14)
            n286 = Delete From Array(array=w605, index=w603) -> (array with subset deleted=w608:i32[])  [unwired: 1 in, 1 out]
            n287 = Delete From Array(array=w607, index=w603) -> (array with subset deleted=w609:T14)  [unwired: 1 in, 1 out]
            n288 = Reverse 1D Array(array=w608) -> (reversed array=w610:i32[])
            n289 = Reverse 1D Array(array=w609) -> (reversed array=w611:T14)
            n290 = Bundle(w610, w611) -> (w602:T15)  [unwired: 1 in]
            n291 = local write "ROI Descriptor out"(w601) -> ()
            n292 = local write "ROI Descriptor"(w602) -> ()
            n293 = property on="Image Out" class="ImageControl"("ROI"=w602) -> ()  [unwired: 2 in, 2 out]
          }
          event "Undo Button": Mouse Down {
            n294 = event-data() -> ()  [unwired: 1 in, 7 out]
            n295 = invoke on="Image Out" class="ImageControl" method="Clear ROI"() -> ()  [unwired: 3 in, 3 out]
          }
          event "Image Folder": Value Change {
            n296 = event-data() -> ()  [unwired: 1 in, 5 out]
            n297 = local read "Image File"() -> (w613:path)
            n298 = call "Vision Acquisition"("Image Path"=w613) -> ("Image Out"=w612:T2)  [unwired: 25 in, 1 out]
            n299 = local write "Image Out 2"(w612) -> ()
            n300 = local write "Image Out"(w612) -> ()
            n301 = invoke on="Image Out" class="ImageControl" method="Clear ROI"() -> ()  [unwired: 3 in, 3 out]
          }
          event "Zoom": Value Change {
            n302 = event-data() -> ()  [unwired: 1 in, 5 out]
            n303 = local read "Zoom"() -> (w614:i16)
            n304 = Bundle("Zoom"=w614, "Zoom"=w614) -> (w615:cluster{"Zoom":i16, "Zoom":i16})  [unwired: 1 in]
            n305 = property on="Image Out" class="ImageControl"("ZoomInteger"=w615) -> ()  [unwired: 2 in, 2 out]
          }
          event Timeout {
            n306 = event-data() -> ()  [unwired: 1 in, 2 out]
          }
          event "Image Out": Mouse Enter {
            (unwired) 6
            n307 = event-data() -> ()  [unwired: 1 in, 3 out]
            n308 = call "Simulate_Keyboard.vi"("Action"=0, "Virtual Key"=162) -> ()  [unwired: 7 in, 1 out]
          }
          event "Image Out": Mouse Leave {
            n309 = event-data() -> ()  [unwired: 1 in, 3 out]
            n310 = flat-sequence {
              frame #0 {
                n311 = Wait (ms)(milliseconds to wait=10) -> ()  [unwired: 1 out]
              }
              frame #1 {
                (unwired) 6
                n312 = call "Simulate_Keyboard.vi"("Action"=2, "Virtual Key"=162) -> ()  [unwired: 7 in, 1 out]
              }
            }
          }
        }
        n313 = Divide(x=w547, y=w524) -> (x/y=w537:sgl)
        n314 = Multiply(x=w537, y=0.5) -> (x*y=w543:dbl)
        n315 = Divide(x=w546, y=w548) -> (x/y=w536:sgl)
        n316 = Multiply(x=w536, y=0.5) -> (x*y=w542:dbl)
        n317 = Unbundle(w556) -> ("X"=w538:u32, "Y"=w539:u32)
        n318 = Subtract(x=w539, y=w542) -> (x-y=w540:dbl)
        n319 = Subtract(x=w538, y=w543) -> (x-y=w541:dbl)
        n320 = Add(x=w541, y=w537) -> (x+y=w555:dbl)
        n321 = Add(x=w540, y=w536) -> (x+y=w554:dbl)
        n322 = Build Array(w481, w504, w483, w479, w475, w505, w506, w461, w460, w453, w457, w456, w459, w444, w498, w501, w511, w502, w454, w509, w497, w491, w494, w493, w489, w487, w485) -> (w507:string[])
        n323 = local write "Current \nRecord"(w507) -> ()
        n324 = Reciprocal(x=w524) -> (1/x=w523:sgl)
        n325 = event shown="[11] \"Save Changes?\": Mouse Down" {
          selector: _ -> [_ _ _ _ _ _ _ _ _ _ _ _ _ _ _ _]
          dyn-events: _ -> [_ _ _ _ _ _ _ _ _ _ _ _ _ _ _ _]
          timeout: 10 -> [_ _ _ _ _ _ _ _ _ _ _ _ _ _ _ _]
          tunnel: [_ _ _ _ _ _ _ _ _ _ _ _ _ TRUE _ TRUE] -> w581
          event Timeout {
            n326 = event-data() -> ()  [unwired: 1 in, 2 out]
          }
          event "Down Button": Mouse Down {
            w955 = 0
            n327 = event-data() -> ()  [unwired: 1 in, 7 out]
            n328 = local read "Transfer File"() -> (w960:path)
            n329 = Strip Path(path=w960) -> (stripped path=w951:path, name=w969:string)
            n330 = local write "Transfer Folder"(w951) -> ()
            n331 = List Folder(path=w951) -> (filenames=w965:string[], error out=w905:errorcluster)  [unwired: 3 in, 2 out]
            n332 = local read "Folder Index"() -> (w907:dbl)
            n333 = Array Size(array=w965) -> (size(s)=w961:i32)
            n334 = Search 1D Array(1D array=w965, element=w969) -> (index of element=w962:i32)  [unwired: 1 in]
            n335 = property on="Image Out" class="ImageControl"() -> (error out=w908:errorcluster, "Image Center Position"=w912:cluster{"X":u32, "Y":u32})  [unwired: 2 in, 1 out]
            n336 = Decrement(x=w961) -> (x-1=w963:i32)
            n337 = Equal?(x=w962, y=w963) -> (x = y?=w964:bool)
            n338 = invoke on="Image Out" class="ImageControl" method="Clear ROI"() -> ()  [unwired: 3 in, 3 out]
            n339 = case shown="False" w964 {
              tunnel: w907 -> [w1122 _]
              tunnel: [w1121 0] -> w906
              tunnel: w905 -> [w1120 w1123]
              tunnel: [w1120 w1123] -> w904
              frame False {
                n340 = Increment(x=w1122) -> (x+1=w1121:dbl)
              }
              frame True {
              }
            }
            n341 = Unbundle(w912) -> ("X"=w910:u32)  [unwired: 1 out]
            n342 = local write "Folder Index"(w906) -> ()
            n343 = Bundle("X"=w910, 0) -> (w911:cluster{"X":u32, i32})  [unwired: 1 in]
            n344 = property on="Image Out" class="ImageControl"(error in=w908, "Image Center Position"=w911) -> ()  [unwired: 1 in, 2 out]
            n345 = Path To String(path=w951) -> (string=w970:string)
            n346 = Index Array(array=w965, index=w906) -> (element=w966:string)
            n347 = local write "Data Name:"(w966) -> ()
            n348 = Concatenate Strings(w970, "\\", w966) -> (w968:string)
            n349 = String To Path(string=w968) -> (path=w878:path)
            n350 = call "Recorded Values.vi"("Path"=w878) -> ("Recorded Char"=w972:T5, "Recorded Prop"=w973:T6, "Fabrication Prop"=w971:T7)  [unwired: 8 in]
            n351 = Unbundle By Name(w972) -> ("Mobility-Sat"=w985:dbl, "Moblitity-Lin"=w986:dbl, "On/Off"=w987:dbl, "Off Current"=w988:dbl, "Vt-Sat"=w873:dbl, "STS"=w989:dbl, "Trap Density-VT"=w990:dbl, "Trap Density-STS"=w991:dbl)
            n352 = Unbundle By Name(w971) -> ("Date Created"=w992:string, "Material"=w974:string, "Solvent"=w975:string, "Concentration"=w976:dbl, "Method"=w977:string, "Dielectric (nm)"=w978:dbl, "Treatment"=w979:string, "Comments"=w980:string)
            n353 = Unbundle By Name(w973) -> ("Date Recorded"=w981:string, "Index"=w982:string, "Length"=w983:dbl, "Width"=w984:dbl, "Sample Temp"=w875:dbl)
            n354 = local write "Date Created"(w992) -> ()
            n355 = local write "Rec: Off I-Sat"(w988) -> ()
            n356 = local write "Rec: Material"(w974) -> ()
            n357 = local write "Rec: VT-Sat"(w873) -> ()
            n358 = local write "Rec: Concentration"(w976) -> ()
            n359 = local write "Rec: Method"(w977) -> ()
            n360 = local write "Rec: Dielectric (d)"(w978) -> ()
            n361 = local write "Surface Treatment:"(w979) -> ()
            n362 = local write "Comments"(w980) -> ()
            n363 = local write "Index"(w982) -> ()
            n364 = local write "Rec: Mobility-Sat"(w985) -> ()
            n365 = local write "Rec: Mobility-Lin"(w986) -> ()
            n366 = local write "Rec: On/Off"(w987) -> ()
            n367 = local write "Rec: STS"(w989) -> ()
            n368 = local write "Rec: Trap Density-VT"(w990) -> ()
            n369 = local write "Rec: Trap Density-STS"(w991) -> ()
            n370 = local write "Rec: Solvent"(w975) -> ()
            n371 = local write "Date Recorded"(w981) -> ()
            n372 = local write "Rec: Length"(w983) -> ()
            n373 = local write "Rec: Width"(w984) -> ()
            n374 = local write "Rec: Temp"(w875) -> ()
            n375 = Equal To 0?(x=w875) -> (x = 0?=w876:bool)
            n376 = case shown="True" w876 {
              tunnel: [w993 w994] -> w874
              tunnel: w875 -> [w993 _]
              frame False {
              }
              frame True {
                n377 = local read "Room Temp"() -> (w994:dbl)
              }
            }
            n378 = local read "NumPts 2"() -> (w899:dbl)
            n379 = local write "Transfer File"(w878) -> ()
            n380 = local read "NumPts"() -> (w903:dbl)
            n381 = call-poly <vilib>:"Read From Spreadsheet File.vi"("file path (dialog if empty)"=w878) -> ("all rows"=w957:string[][])  [unwired: 6 in, 4 out]
            n382 = call "Mobility-Vt Calculator-File.vi"("NumPts"=w903, "Path"=w878) -> ("XY Graph-Sat"=w901:cluster{dbl[], dbl[]}[], "XY Graph-Lin"=w872:cluster{dbl[], dbl[]}[], "Output"=w902:T8, "Index-Sat"=w900:dbl, "Index-Lin"=w886:dbl)  [unwired: 4 in, 1 out]
            n383 = local read "New: Dielectric"() -> (w883:dbl)
            n384 = call "STS Calculator-File.vi"("NumPts"=w899, "Path"=w878) -> ("STS Index-Sat"=w898:dbl, "XY Graph-Sat"=w897:cluster{dbl[], dbl[]}[], "Ouput"=w896:cluster{"STS-Sat":dbl, "STS-Lin":dbl})  [unwired: 5 in, 2 out]
            n385 = Unbundle By Name(w902) -> ("Mobility-Sat"=w895:dbl, "Vt-Sat"=w882:dbl, "Mobility-Lin"=w894:dbl, "Vt-Lin"=w893:dbl, "Off I-Sat"=w879:dbl, "On/Off I-Sat"=w871:dbl)
            n386 = Unbundle By Name(w896) -> ("STS-Sat"=w877:dbl)  [unwired: 1 out]
            n387 = local write "Index 2"(w898) -> ()
            n388 = local write "XY Graph 2"(w897) -> ()
            n389 = local write "MobVi Index"(w900) -> ()
            n390 = local write "Slide"(w900) -> ()
            n391 = local write "XY Graph"(w901) -> ()
            n392 = Array Size(array=w957) -> (size(s)=w956:i32[])
            n393 = call "Trap Density_VT.vi"("VT"=w882, "Dielectric"=w883) -> ("Trap Density-VT"=w881:dbl)
            n394 = call "Trap Density_STS.vi"("Temp (T) [K]"=w874, "S.T.S. (S)"=w877, "Dielectric"=w883) -> ("Trap Density (N)"=w880:dbl)  [unwired: 8 in]
            n395 = local write "New: STS"(w877) -> ()
            n396 = local write "Calc: STS"(w877) -> ()
            n397 = local write "Calc: Mobility-Sat"(w895) -> ()
            n398 = local write "Calc: Off I-Sat"(w893) -> ()
            n399 = local write "Calc: Mobility-Lin"(w894) -> ()
            n400 = Index Array(array=w956, index=w955) -> (element=w937:i32)
            n401 = Decimate 1D Array(w897) -> (w931:cluster{dbl[], dbl[]}[])  [unwired: 1 out]
            n402 = Decimate 1D Array(w901) -> (w941:cluster{dbl[], dbl[]}[])  [unwired: 1 out]
            n403 = local write "Calc: Off I-Sat"(w879) -> ()
            n404 = local write "Calc: On/Off"(w871) -> ()
            n405 = Decimate 1D Array(w872) -> (w892:cluster{dbl[], dbl[]}[])  [unwired: 1 out]
            n406 = local write "Calc: VT-Sat"(w882) -> ()
            n407 = Array Subset(array=w957, index (row)=w955, index (col)=w955, length (col)=3) -> (w958:string[][])  [unwired: 1 in]
            n408 = local write "Calc: Trap Density-VT"(w881) -> ()
            n409 = local write "Calc: Trap Density-STS"(w880) -> ()
            n410 = local write "New: Trap Density-STS"(w880) -> ()
            n411 = local write "New: Trap Density-VT"(w881) -> ()
            n412 = local write "XY Graph-Lin"(w872) -> ()
            n413 = Array To Cluster(array=w931) -> (cluster=w929:T9)
            n414 = Array To Cluster(array=w941) -> (cluster=w943:T9)
            n415 = local write "New: VT-Lin"(w893) -> ()
            n416 = local write "New: VT-Sat"(w882) -> ()
            n417 = local write "New: Mobility-Sat"(w895) -> ()
            n418 = local write "New: Mobility-Lin"(w894) -> ()
            n419 = Reshape Array(w958, w937) -> (w944:string[])
            n420 = Array To Cluster(array=w892) -> (cluster=w891:T9)
            n421 = Subtract(x=w937, y=20) -> (x-y=w936:i32)
            n422 = property on="Slide" class="Slide (strict)"("Scale.Maximum"=w936) -> ()  [unwired: 2 in, 2 out]
            n423 = Unbundle(w929) -> ("[0]"=w930:cluster{dbl[], dbl[]})  [unwired: 8 out]
            n424 = Unbundle(w943) -> ("[0]"=w942:cluster{dbl[], dbl[]})  [unwired: 8 out]
            n425 = Unbundle(w891) -> ("[0]"=w888:cluster{dbl[], dbl[]})  [unwired: 8 out]
            n426 = Search 1D Array(1D array=w944, element="Index:") -> (index of element=w952:i32)  [unwired: 1 in]
            n427 = local read "NumPts"() -> (w887:dbl)
            n428 = Unbundle(w888) -> (w890:dbl[], w889:dbl[])
            n429 = Increment(x=w952) -> (x+1=w953:i32)
            n430 = Unbundle(w930) -> (w928:dbl[], w927:dbl[])
            n431 = Unbundle(w942) -> (w933:dbl[], w932:dbl[])
            n432 = Array Subset(array=w890, index=w886, length=w887) -> (w885:dbl[])
            n433 = Array Subset(array=w889, index=w886, length=w887) -> (w884:dbl[])
            n434 = Array Subset(array=w928, index=w898, length=w899) -> (w935:dbl[])
            n435 = Array Subset(array=w927, index=w898, length=w899) -> (w934:dbl[])
            n436 = Array Subset(array=w933, index=w900, length=w903) -> (w940:dbl[])
            n437 = Array Subset(array=w932, index=w900, length=w903) -> (w939:dbl[])
            n438 = Index Array(array=w944, index=w953) -> (element=w916:string)
            n439 = local write "Lin-Vg Array-Used"(w885) -> ()
            n440 = local write "Sat Vg Array-Used"(w940) -> ()
            n441 = local write "Vg Array-Log-Used"(w934) -> ()
            n442 = local write "Lin Id-Used"(w884) -> ()
            n443 = local read "Image Folder"() -> (w914:path)
            n444 = local write "Sat Id-Used"(w939) -> ()
            n445 = local write "Sat Id-Log-Used"(w935) -> ()
            n446 = List Folder(path=w914, error in=w904) -> (filenames=w950:string[], error out=w917:errorcluster)  [unwired: 2 in, 2 out]
            n447 = while {
              tunnel: w950 -> [w1007]
              tunnel: w916 -> [w1005]
              tunnel: [w1004] -> _
              tunnel: [w1004] -> w949
              tunnel: w937 -> [w1003]
              i -> [w1004]
              stop <- w1000 stop-if-true
              n448 = Index Array(array=w1007, index=w1004) -> (element=w1008:string)
              n449 = xnode "Match Regular Expression"("input string"=w1008, "regular expression"=w1005) -> ("whole match"=w1006:string)  [unwired: 4 in, 4 out]
              n450 = Equal?(x=w1006, y=w1005) -> (x = y?=w1002:bool)
              n451 = Equal?(x=w1003, y=w1004) -> (x = y?=w1001:bool)
              n452 = Or(x=w1002, y=w1001) -> (x .or. y?=w1000:bool)
            }
            n453 = Build Path(base path=w914, name or relative path="ROI") -> (appended path=w913:path)
            n454 = Path To String(path=w914) -> (string=w947:string)
            n455 = Index Array(array=w950, index=w949) -> (element=w925:string)
            n456 = invoke on="Image Out" class="ImageControl" method="Clear ROI"(error in=w917) -> (error out=w920:errorcluster)  [unwired: 2 in, 2 out]
            n457 = local write "Image Name"(w925) -> ()
            n458 = Build Path(base path=w913, name or relative path=w916) -> (appended path=w921:path)
            n459 = call <vilib>:"Check if File or Folder Exists.vi"("error in (no error)"=w920, "path"=w921) -> ("file or folder exists?"=w918:bool, "dup path"=w919:path)  [unwired: 7 in, 1 out]
            n460 = Concatenate Strings(w947, "\\", w925) -> (w946:string)
            n461 = case shown="False" w918 {
              tunnel: w919 -> [_ w995]
              frame False {
              }
              frame True {
                n462 = Read from Text File(file (use dialog)=w995) -> (text=w999:string)  [unwired: 3 in, 3 out]
                n463 = property on="Image Out" class="ImageControl"() -> ("ROI"=w996:T10)  [unwired: 2 in, 2 out]
                n464 = Unflatten From String(type=w996, binary string=w999) -> (value=w997:T10, error out=w998:errorcluster)  [unwired: 3 in, 1 out]
                n465 = property on="Image Out" class="ImageControl"(error in=w998, "ROI"=w997) -> ()  [unwired: 1 in, 2 out]
              }
            }
            n466 = String To Path(string=w946) -> (path=w924:path)
            n467 = Empty String/Path?(string/path=w925) -> (empty?=w926:bool)
            n468 = local read "No Image File"() -> (w922:path)
            n469 = Select(t=w922, s=w926, f=w924) -> (s? t:f=w923:path)
            n470 = local write "Image File"(w923) -> ()
            n471 = call "Vision Acquisition4"("Image Path"=w923) -> ("Image Out"=w948:T2)  [unwired: 25 in, 1 out]
            n472 = local write "Image Out"(w948) -> ()
            n473 = local write "Image Out 2"(w948) -> ()
          }
          event "Transfer File": Value Change {
            w1231 = 0
            n474 = event-data() -> ()  [unwired: 1 in, 5 out]
            n475 = local read "Transfer File"() -> (w1227:path)
            n476 = Strip Path(path=w1227) -> (stripped path=w1226:path, name=w1240:string)
            n477 = local write "Transfer Folder"(w1226) -> ()
            n478 = property on="Image Out" class="ImageControl"() -> (error out=w1182:errorcluster, "Image Center Position"=w1186:cluster{"X":u32, "Y":u32})  [unwired: 2 in, 1 out]
            n479 = List Folder(path=w1226) -> (filenames=w1236:string[], error out=w1192:errorcluster)  [unwired: 3 in, 2 out]
            n480 = Search 1D Array(1D array=w1236, element=w1240) -> (index of element=w1181:i32)  [unwired: 1 in]
            n481 = local write "Folder Index"(w1181) -> ()
            n482 = Unbundle(w1186) -> ("X"=w1184:u32)  [unwired: 1 out]
            n483 = Path To String(path=w1226) -> (string=w1241:string)
            n484 = Index Array(array=w1236, index=w1181) -> (element=w1237:string)
            n485 = Bundle("X"=w1184, 0) -> (w1185:cluster{"X":u32, i32})  [unwired: 1 in]
            n486 = local write "Data Name:"(w1237) -> ()
            n487 = property on="Image Out" class="ImageControl"(error in=w1182, "Image Center Position"=w1185) -> ()  [unwired: 1 in, 2 out]
            n488 = Concatenate Strings(w1241, "\\", w1237) -> (w1239:string)
            n489 = String To Path(string=w1239) -> (path=w1132:path)
            n490 = call "Recorded Values.vi"("Path"=w1132) -> ("Recorded Char"=w1179:T5, "Recorded Prop"=w1178:T6, "Fabrication Prop"=w1180:T7)  [unwired: 8 in]
            n491 = Unbundle By Name(w1179) -> ("Mobility-Sat"=w1166:dbl, "Moblitity-Lin"=w1165:dbl, "On/Off"=w1164:dbl, "Off Current"=w1163:dbl, "Vt-Sat"=w1128:dbl, "STS"=w1162:dbl, "Trap Density-VT"=w1161:dbl, "Trap Density-STS"=w1160:dbl)
            n492 = Unbundle By Name(w1180) -> ("Date Created"=w1159:string, "Material"=w1177:string, "Solvent"=w1176:string, "Concentration"=w1175:dbl, "Method"=w1174:string, "Dielectric (nm)"=w1173:dbl, "Treatment"=w1172:string, "Comments"=w1171:string)
            n493 = Unbundle By Name(w1178) -> ("Date Recorded"=w1170:string, "Index"=w1169:string, "Length"=w1168:dbl, "Width"=w1167:dbl, "Sample Temp"=w1130:dbl)
            n494 = local write "Date Created"(w1159) -> ()
            n495 = local write "Rec: Material"(w1177) -> ()
            n496 = local write "Rec: Off I-Sat"(w1163) -> ()
            n497 = local write "Rec: VT-Sat"(w1128) -> ()
            n498 = local write "Rec: Concentration"(w1175) -> ()
            n499 = local write "Rec: Method"(w1174) -> ()
            n500 = local write "Rec: Dielectric (d)"(w1173) -> ()
            n501 = local write "Surface Treatment:"(w1172) -> ()
            n502 = local write "Comments"(w1171) -> ()
            n503 = local write "Index"(w1169) -> ()
            n504 = local write "Rec: Mobility-Sat"(w1166) -> ()
            n505 = local write "Rec: Mobility-Lin"(w1165) -> ()
            n506 = local write "Rec: On/Off"(w1164) -> ()
            n507 = local write "Rec: STS"(w1162) -> ()
            n508 = local write "Rec: Trap Density-VT"(w1161) -> ()
            n509 = local write "Rec: Trap Density-STS"(w1160) -> ()
            n510 = local write "Rec: Solvent"(w1176) -> ()
            n511 = local write "Date Recorded"(w1170) -> ()
            n512 = local write "Rec: Length"(w1168) -> ()
            n513 = local write "Rec: Width"(w1167) -> ()
            n514 = local write "Rec: Temp"(w1130) -> ()
            n515 = Equal To 0?(x=w1130) -> (x = 0?=w1131:bool)
            n516 = case shown="False" w1131 {
              tunnel: [w1242 w1243] -> w1129
              tunnel: w1130 -> [w1242 _]
              frame False {
              }
              frame True {
                n517 = local read "Room Temp"() -> (w1243:dbl)
              }
            }
            n518 = local write "Transfer File"(w1132) -> ()
            n519 = local read "NumPts 2"() -> (w1154:dbl)
            n520 = local read "NumPts"() -> (w1155:dbl)
            n521 = call-poly <vilib>:"Read From Spreadsheet File.vi"("file path (dialog if empty)"=w1132) -> ("all rows"=w1233:string[][])  [unwired: 6 in, 4 out]
            n522 = local read "New: Dielectric"() -> (w1138:dbl)
            n523 = call "STS Calculator-File.vi"("NumPts"=w1154, "Path"=w1132) -> ("STS Index-Sat"=w1152:dbl, "XY Graph-Sat"=w1153:cluster{dbl[], dbl[]}[], "Ouput"=w1151:cluster{"STS-Sat":dbl, "STS-Lin":dbl})  [unwired: 5 in, 2 out]
            n524 = call "Mobility-Vt Calculator-File.vi"("NumPts"=w1155, "Path"=w1132) -> ("XY Graph-Sat"=w1158:cluster{dbl[], dbl[]}[], "XY Graph-Lin"=w1127:cluster{dbl[], dbl[]}[], "Output"=w1156:T8, "Index-Sat"=w1157:dbl, "Index-Lin"=w1144:dbl)  [unwired: 4 in, 1 out]
            n525 = Unbundle By Name(w1156) -> ("Mobility-Sat"=w1140:dbl, "Vt-Sat"=w1134:dbl, "Mobility-Lin"=w1139:dbl, "Vt-Lin"=w1125:dbl, "Off I-Sat"=w1133:dbl, "On/Off I-Sat"=w1126:dbl)
            n526 = local write "Index 2"(w1152) -> ()
            n527 = local write "XY Graph 2"(w1153) -> ()
            n528 = Unbundle By Name(w1151) -> ("STS-Sat"=w1135:dbl)  [unwired: 1 out]
            n529 = local write "MobVi Index"(w1157) -> ()
            n530 = Array Size(array=w1233) -> (size(s)=w1232:i32[])
            n531 = call "Trap Density_VT.vi"("VT"=w1134, "Dielectric"=w1138) -> ("Trap Density-VT"=w1137:dbl)
            n532 = call "Trap Density_STS.vi"("Temp (T) [K]"=w1129, "S.T.S. (S)"=w1135, "Dielectric"=w1138) -> ("Trap Density (N)"=w1136:dbl)  [unwired: 8 in]
            n533 = local write "Slide"(w1157) -> ()
            n534 = local write "Calc: Mobility-Lin"(w1139) -> ()
            n535 = local write "Calc: Mobility-Sat"(w1140) -> ()
            n536 = local write "Calc: VT-Sat"(w1134) -> ()
            n537 = local write "Calc: Off I-Sat"(w1133) -> ()
            n538 = local write "Calc: VT-Lin"(w1125) -> ()
            n539 = local write "Calc: On/Off"(w1126) -> ()
            n540 = local write "Calc: STS"(w1135) -> ()
            n541 = Decimate 1D Array(w1127) -> (w1150:cluster{dbl[], dbl[]}[])  [unwired: 1 out]
            n542 = local write "Calc: Trap Density-VT"(w1137) -> ()
            n543 = local write "Calc: Trap Density-STS"(w1136) -> ()
            n544 = local write "New: Trap Density-STS"(w1136) -> ()
            n545 = local write "New: Trap Density-VT"(w1137) -> ()
            n546 = local write "XY Graph-Lin"(w1127) -> ()
            n547 = local write "New: VT-Sat"(w1134) -> ()
            n548 = Decimate 1D Array(w1153) -> (w1207:cluster{dbl[], dbl[]}[])  [unwired: 1 out]
            n549 = Index Array(array=w1232, index=w1231) -> (element=w1213:i32)
            n550 = Decimate 1D Array(w1158) -> (w1216:cluster{dbl[], dbl[]}[])  [unwired: 1 out]
            n551 = local write "XY Graph"(w1158) -> ()
            n552 = local write "New: Mobility-Lin"(w1139) -> ()
            n553 = Array Subset(array=w1233, index (row)=w1231, index (col)=w1231, length (col)=3) -> (w1234:string[][])  [unwired: 1 in]
            n554 = local write "New: VT-Lin"(w1125) -> ()
            n555 = Array To Cluster(array=w1150) -> (cluster=w1149:T9)
            n556 = local write "New: STS"(w1135) -> ()
            n557 = local write "New: Mobility-Sat"(w1140) -> ()
            n558 = Array To Cluster(array=w1207) -> (cluster=w1205:T9)
            n559 = Array To Cluster(array=w1216) -> (cluster=w1218:T9)
            n560 = Reshape Array(w1234, w1213) -> (w1219:string[])
            n561 = Subtract(x=w1213, y=20) -> (x-y=w1211:i32)
            n562 = Unbundle(w1149) -> ("[0]"=w1148:cluster{dbl[], dbl[]})  [unwired: 8 out]
            n563 = property on="Slide" class="Slide (strict)"("Scale.Maximum"=w1211) -> ()  [unwired: 2 in, 2 out]
            n564 = local read "NumPts"() -> (w1145:dbl)
            n565 = Unbundle(w1148) -> (w1147:dbl[], w1146:dbl[])
            n566 = Unbundle(w1205) -> ("[0]"=w1206:cluster{dbl[], dbl[]})  [unwired: 8 out]
            n567 = Unbundle(w1218) -> ("[0]"=w1217:cluster{dbl[], dbl[]})  [unwired: 8 out]
            n568 = Search 1D Array(1D array=w1219, element="Index:") -> (index of element=w1228:i32)  [unwired: 1 in]
            n569 = local read "NumPts"() -> (w1141:dbl)
            n570 = Array Subset(array=w1147, index=w1144, length=w1145) -> (w1143:dbl[])
            n571 = Array Subset(array=w1146, index=w1144, length=w1145) -> (w1142:dbl[])
            n572 = Increment(x=w1228) -> (x+1=w1229:i32)
            n573 = Unbundle(w1206) -> (w1203:dbl[], w1202:dbl[])
            n574 = Unbundle(w1217) -> (w1204:dbl[], w1208:dbl[])
            n575 = local read "Image Folder"() -> (w1188:path)
            n576 = local write "Lin-Vg Array-Used"(w1143) -> ()
            n577 = Array Subset(array=w1203, index=w1152, length=w1154) -> (w1210:dbl[])
            n578 = Array Subset(array=w1202, index=w1152, length=w1154) -> (w1209:dbl[])
            n579 = Array Subset(array=w1204, index=w1157, length=w1141) -> (w1215:dbl[])
            n580 = Array Subset(array=w1208, index=w1157, length=w1141) -> (w1214:dbl[])
            n581 = Index Array(array=w1219, index=w1229) -> (element=w1190:string)
            n582 = local write "Lin Id-Used"(w1142) -> ()
            n583 = local write "Sat Vg Array-Used"(w1215) -> ()
            n584 = local write "Vg Array-Log-Used"(w1209) -> ()
            n585 = local write "Sat Id-Log-Used"(w1210) -> ()
            n586 = local write "Sat Id-Used"(w1214) -> ()
            n587 = local write "Index"(w1190) -> ()
            n588 = List Folder(path=w1188, error in=w1192) -> (filenames=w1224:string[], error out=w1191:errorcluster)  [unwired: 2 in, 2 out]
            n589 = Build Path(base path=w1188, name or relative path="ROI") -> (appended path=w1187:path)
            n590 = invoke on="Image Out" class="ImageControl" method="Clear ROI"(error in=w1191) -> (error out=w1195:errorcluster)  [unwired: 2 in, 2 out]
            n591 = Build Path(base path=w1187, name or relative path=w1190) -> (appended path=w1196:path)
            n592 = while {
              tunnel: w1224 -> [w1256]
              tunnel: w1190 -> [w1254]
              tunnel: [w1253] -> _
              tunnel: [w1253] -> w1223
              tunnel: w1213 -> [w1252]
              i -> [w1253]
              stop <- w1249 stop-if-true
              n593 = Index Array(array=w1256, index=w1253) -> (element=w1257:string)
              n594 = xnode "Match Regular Expression"("input string"=w1257, "regular expression"=w1254) -> ("whole match"=w1255:string)  [unwired: 4 in, 4 out]
              n595 = Equal?(x=w1255, y=w1254) -> (x = y?=w1251:bool)
              n596 = Equal?(x=w1252, y=w1253) -> (x = y?=w1250:bool)
              n597 = Or(x=w1251, y=w1250) -> (x .or. y?=w1249:bool)
            }
            n598 = call <vilib>:"Check if File or Folder Exists.vi"("error in (no error)"=w1195, "path"=w1196) -> ("file or folder exists?"=w1193:bool, "dup path"=w1194:path)  [unwired: 7 in, 1 out]
            n599 = case shown="True" w1193 {
              tunnel: w1194 -> [_ w1244]
              frame False {
              }
              frame True {
                n600 = Read from Text File(file (use dialog)=w1244) -> (text=w1248:string)  [unwired: 3 in, 3 out]
                n601 = property on="Image Out" class="ImageControl"() -> ("ROI"=w1245:T10)  [unwired: 2 in, 2 out]
                n602 = Unflatten From String(type=w1245, binary string=w1248) -> (value=w1246:T10, error out=w1247:errorcluster)  [unwired: 3 in, 1 out]
                n603 = property on="Image Out" class="ImageControl"(error in=w1247, "ROI"=w1246) -> ()  [unwired: 1 in, 2 out]
              }
            }
            n604 = invoke on="Image Out" class="ImageControl" method="Clear ROI"() -> ()  [unwired: 3 in, 3 out]
            n605 = Path To String(path=w1188) -> (string=w1222:string)
            n606 = Index Array(array=w1224, index=w1223) -> (element=w1200:string)
            n607 = Concatenate Strings(w1222, "\\", w1200) -> (w1221:string)
            n608 = local write "Image Name"(w1200) -> ()
            n609 = String To Path(string=w1221) -> (path=w1199:path)
            n610 = Empty String/Path?(string/path=w1200) -> (empty?=w1201:bool)
            n611 = local read "No Image File"() -> (w1197:path)
            n612 = Select(t=w1197, s=w1201, f=w1199) -> (s? t:f=w1198:path)
            n613 = local write "Image File"(w1198) -> ()
            n614 = call "Vision Acquisition3"("Image Path"=w1198) -> ("Image Out"=w1225:T2)  [unwired: 25 in, 1 out]
            n615 = local write "Image Out"(w1225) -> ()
            n616 = local write "Image Out 2"(w1225) -> ()
          }
          event "Up Button": Mouse Down {
            w1476 = 0
            n617 = event-data() -> ()  [unwired: 1 in, 5 out]
            n618 = local read "Transfer File"() -> (w1472:path)
            n619 = Strip Path(path=w1472) -> (stripped path=w1471:path, name=w1487:string)
            n620 = local write "Transfer Folder"(w1471) -> ()
            n621 = List Folder(path=w1471) -> (filenames=w1481:string[], error out=w1438:errorcluster)  [unwired: 3 in, 2 out]
            n622 = Array Size(array=w1481) -> (size(s)=w1426:i32)
            n623 = Search 1D Array(1D array=w1481, element=w1487) -> (index of element=w1482:i32)  [unwired: 1 in]
            n624 = Equal To 0?(x=w1482) -> (x = 0?=w1483:bool)
            n625 = local read "Folder Index"() -> (w1425:dbl)
            n626 = property on="Image Out" class="ImageControl"() -> (error out=w1428:errorcluster, "Image Center Position"=w1432:cluster{"X":u32, "Y":u32})  [unwired: 2 in, 1 out]
            n627 = case shown="True" w1483 {
              tunnel: w1425 -> [w1617 _]
              tunnel: [w1616 w1618] -> w1424
              tunnel: w1426 -> [_ w1619]
              frame False {
                n628 = Decrement(x=w1617) -> (x-1=w1616:dbl)
              }
              frame True {
                n629 = Decrement(x=w1619) -> (x-1=w1618:i32)
              }
            }
            n630 = Unbundle(w1432) -> ("X"=w1430:u32)  [unwired: 1 out]
            n631 = local write "Folder Index"(w1424) -> ()
            n632 = Bundle("X"=w1430, 0) -> (w1431:cluster{"X":u32, i32})  [unwired: 1 in]
            n633 = Path To String(path=w1471) -> (string=w1488:string)
            n634 = Index Array(array=w1481, index=w1424) -> (element=w1484:string)
            n635 = local write "Data Name:"(w1484) -> ()
            n636 = property on="Image Out" class="ImageControl"(error in=w1428, "Image Center Position"=w1431) -> ()  [unwired: 1 in, 2 out]
            n637 = Concatenate Strings(w1488, "\\", w1484) -> (w1486:string)
            n638 = String To Path(string=w1486) -> (path=w1375:path)
            n639 = call "Recorded Values.vi"("Path"=w1375) -> ("Recorded Char"=w1422:T5, "Recorded Prop"=w1421:T6, "Fabrication Prop"=w1423:T7)  [unwired: 8 in]
            n640 = Unbundle By Name(w1422) -> ("Mobility-Sat"=w1409:dbl, "Moblitity-Lin"=w1408:dbl, "On/Off"=w1407:dbl, "Off Current"=w1406:dbl, "Vt-Sat"=w1371:dbl, "STS"=w1405:dbl, "Trap Density-VT"=w1404:dbl, "Trap Density-STS"=w1403:dbl)
            n641 = Unbundle By Name(w1423) -> ("Date Created"=w1402:string, "Material"=w1420:string, "Solvent"=w1419:string, "Concentration"=w1418:dbl, "Method"=w1417:string, "Dielectric (nm)"=w1416:dbl, "Treatment"=w1415:string, "Comments"=w1414:string)
            n642 = Unbundle By Name(w1421) -> ("Date Recorded"=w1413:string, "Index"=w1412:string, "Length"=w1411:dbl, "Width"=w1410:dbl, "Sample Temp"=w1372:dbl)
            n643 = local write "Date Created"(w1402) -> ()
            n644 = local write "Rec: Material"(w1420) -> ()
            n645 = local write "Rec: Off I-Sat"(w1406) -> ()
            n646 = local write "Rec: VT-Sat"(w1371) -> ()
            n647 = local write "Rec: Solvent"(w1419) -> ()
            n648 = local write "Rec: Concentration"(w1418) -> ()
            n649 = local write "Rec: Method"(w1417) -> ()
            n650 = local write "Rec: Dielectric (d)"(w1416) -> ()
            n651 = local write "Surface Treatment:"(w1415) -> ()
            n652 = local write "Comments"(w1414) -> ()
            n653 = local write "Index"(w1412) -> ()
            n654 = local write "Rec: Mobility-Sat"(w1409) -> ()
            n655 = local write "Rec: Mobility-Lin"(w1408) -> ()
            n656 = local write "Rec: On/Off"(w1407) -> ()
            n657 = local write "Rec: STS"(w1405) -> ()
            n658 = local write "Rec: Trap Density-VT"(w1404) -> ()
            n659 = local write "Rec: Trap Density-STS"(w1403) -> ()
            n660 = local write "Date Recorded"(w1413) -> ()
            n661 = local write "Rec: Length"(w1411) -> ()
            n662 = local write "Rec: Width"(w1410) -> ()
            n663 = local write "Rec: Temp"(w1372) -> ()
            n664 = Equal To 0?(x=w1372) -> (x = 0?=w1374:bool)
            n665 = case shown="False" w1374 {
              tunnel: [w1489 w1490] -> w1373
              tunnel: w1372 -> [w1489 _]
              frame False {
              }
              frame True {
                n666 = local read "Room Temp"() -> (w1490:dbl)
              }
            }
            n667 = local write "Transfer File"(w1375) -> ()
            n668 = local read "NumPts 2"() -> (w1397:dbl)
            n669 = local read "NumPts"() -> (w1401:dbl)
            n670 = local read "New: Dielectric"() -> (w1381:dbl)
            n671 = call "Mobility-Vt Calculator-File.vi"("NumPts"=w1401, "Path"=w1375) -> ("XY Graph-Sat"=w1399:cluster{dbl[], dbl[]}[], "XY Graph-Lin"=w1370:cluster{dbl[], dbl[]}[], "Output"=w1400:T8, "Index-Sat"=w1398:dbl, "Index-Lin"=w1385:dbl)  [unwired: 4 in, 1 out]
            n672 = call "STS Calculator-File.vi"("NumPts"=w1397, "Path"=w1375) -> ("STS Index-Sat"=w1396:dbl, "XY Graph-Sat"=w1395:cluster{dbl[], dbl[]}[], "Ouput"=w1394:cluster{"STS-Sat":dbl, "STS-Lin":dbl})  [unwired: 5 in, 2 out]
            n673 = call-poly <vilib>:"Read From Spreadsheet File.vi"("file path (dialog if empty)"=w1375) -> ("all rows"=w1478:string[][])  [unwired: 6 in, 4 out]
            n674 = Unbundle By Name(w1400) -> ("Mobility-Sat"=w1384:dbl, "Vt-Sat"=w1377:dbl, "Mobility-Lin"=w1383:dbl, "Vt-Lin"=w1382:dbl, "Off I-Sat"=w1376:dbl, "On/Off I-Sat"=w1369:dbl)
            n675 = Unbundle By Name(w1394) -> ("STS-Sat"=w1378:dbl)  [unwired: 1 out]
            n676 = local write "Index 2"(w1396) -> ()
            n677 = local write "XY Graph 2"(w1395) -> ()
            n678 = local write "MobVi Index"(w1398) -> ()
            n679 = local write "Slide"(w1398) -> ()
            n680 = local write "XY Graph"(w1399) -> ()
            n681 = local write "Calc: Mobility-Sat"(w1384) -> ()
            n682 = local write "Calc: VT-Sat"(w1377) -> ()
            n683 = local write "Calc: Mobility-Lin"(w1383) -> ()
            n684 = local write "Calc: Off I-Sat"(w1376) -> ()
            n685 = local write "Calc: On/Off"(w1369) -> ()
            n686 = Array Size(array=w1478) -> (size(s)=w1477:i32[])
            n687 = local write "Calc: VT-Lin"(w1382) -> ()
            n688 = call "Trap Density_VT.vi"("VT"=w1377, "Dielectric"=w1381) -> ("Trap Density-VT"=w1380:dbl)
            n689 = call "Trap Density_STS.vi"("Temp (T) [K]"=w1373, "S.T.S. (S)"=w1378, "Dielectric"=w1381) -> ("Trap Density (N)"=w1379:dbl)  [unwired: 8 in]
            n690 = local write "Calc: STS"(w1378) -> ()
            n691 = local write "New: STS"(w1378) -> ()
            n692 = Decimate 1D Array(w1370) -> (w1393:cluster{dbl[], dbl[]}[])  [unwired: 1 out]
            n693 = local write "Calc: Trap Density-VT"(w1380) -> ()
            n694 = local write "New: VT-Sat"(w1377) -> ()
            n695 = local write "Calc: Trap Density-STS"(w1379) -> ()
            n696 = local write "New: Trap Density-STS"(w1379) -> ()
            n697 = local write "New: Trap Density-VT"(w1380) -> ()
            n698 = local write "XY Graph-Lin"(w1370) -> ()
            n699 = local write "New: VT-Lin"(w1382) -> ()
            n700 = local write "New: Mobility-Sat"(w1384) -> ()
            n701 = local write "New: Mobility-Lin"(w1383) -> ()
            n702 = Decimate 1D Array(w1395) -> (w1455:cluster{dbl[], dbl[]}[])  [unwired: 1 out]
            n703 = Index Array(array=w1477, index=w1476) -> (element=w1461:i32)
            n704 = Decimate 1D Array(w1399) -> (w1465:cluster{dbl[], dbl[]}[])  [unwired: 1 out]
            n705 = Array To Cluster(array=w1393) -> (cluster=w1392:T9)
            n706 = Array Subset(array=w1478, index (row)=w1476, index (col)=w1476, length (col)=3) -> (w1479:string[][])  [unwired: 1 in]
            n707 = Array To Cluster(array=w1455) -> (cluster=w1453:T9)
            n708 = Array To Cluster(array=w1465) -> (cluster=w1467:T9)
            n709 = Reshape Array(w1479, w1461) -> (w1468:string[])
            n710 = Subtract(x=w1461, y=20) -> (x-y=w1460:i32)
            n711 = Unbundle(w1392) -> ("[0]"=w1389:cluster{dbl[], dbl[]})  [unwired: 8 out]
            n712 = property on="Slide" class="Slide (strict)"("Scale.Maximum"=w1460) -> ()  [unwired: 2 in, 2 out]
            n713 = Unbundle(w1453) -> ("[0]"=w1454:cluster{dbl[], dbl[]})  [unwired: 8 out]
            n714 = Unbundle(w1467) -> ("[0]"=w1466:cluster{dbl[], dbl[]})  [unwired: 8 out]
            n715 = local read "NumPts"() -> (w1386:dbl)
            n716 = Unbundle(w1389) -> (w1388:dbl[], w1387:dbl[])
            n717 = Search 1D Array(1D array=w1468, element="Index:") -> (index of element=w1473:i32)  [unwired: 1 in]
            n718 = Increment(x=w1473) -> (x+1=w1474:i32)
            n719 = Unbundle(w1454) -> (w1452:dbl[], w1451:dbl[])
            n720 = Unbundle(w1466) -> (w1459:dbl[], w1458:dbl[])
            n721 = Array Subset(array=w1388, index=w1385, length=w1386) -> (w1390:dbl[])
            n722 = Array Subset(array=w1387, index=w1385, length=w1386) -> (w1391:dbl[])
            n723 = local read "Image Folder"() -> (w1427:path)
            n724 = local write "Lin-Vg Array-Used"(w1390) -> ()
            n725 = Array Subset(array=w1452, index=w1396, length=w1397) -> (w1457:dbl[])
            n726 = Array Subset(array=w1451, index=w1396, length=w1397) -> (w1456:dbl[])
            n727 = Array Subset(array=w1459, index=w1398, length=w1401) -> (w1464:dbl[])
            n728 = Array Subset(array=w1458, index=w1398, length=w1401) -> (w1463:dbl[])
            n729 = local write "Lin Id-Used"(w1391) -> ()
            n730 = Index Array(array=w1468, index=w1474) -> (element=w1434:string)
            n731 = local write "Sat Vg Array-Used"(w1464) -> ()
            n732 = local write "Vg Array-Log-Used"(w1456) -> ()
            n733 = local write "Sat Id-Log-Used"(w1457) -> ()
            n734 = local write "Sat Id-Used"(w1463) -> ()
            n735 = local write "Index"(w1434) -> ()
            n736 = List Folder(path=w1427, error in=w1438) -> (filenames=w1470:string[], error out=w1437:errorcluster)  [unwired: 2 in, 2 out]
            n737 = Build Path(base path=w1427, name or relative path="ROI") -> (appended path=w1435:path)
            n738 = invoke on="Image Out" class="ImageControl" method="Clear ROI"(error in=w1437) -> (error out=w1441:errorcluster)  [unwired: 2 in, 2 out]
            n739 = while {
              tunnel: w1470 -> [w1503]
              tunnel: w1434 -> [w1501]
              tunnel: [w1500] -> w1469
              tunnel: w1461 -> [w1499]
              i -> [w1500]
              stop <- w1496 stop-if-true
              n740 = Index Array(array=w1503, index=w1500) -> (element=w1504:string)
              n741 = xnode "Match Regular Expression"("input string"=w1504, "regular expression"=w1501) -> ("whole match"=w1502:string)  [unwired: 4 in, 4 out]
              n742 = Equal?(x=w1502, y=w1501) -> (x = y?=w1498:bool)
              n743 = Equal?(x=w1499, y=w1500) -> (x = y?=w1497:bool)
              n744 = Or(x=w1498, y=w1497) -> (x .or. y?=w1496:bool)
            }
            n745 = Build Path(base path=w1435, name or relative path=w1434) -> (appended path=w1433:path)
            n746 = call <vilib>:"Check if File or Folder Exists.vi"("error in (no error)"=w1441, "path"=w1433) -> ("file or folder exists?"=w1439:bool, "dup path"=w1440:path)  [unwired: 7 in, 1 out]
            n747 = case shown="True" w1439 {
              tunnel: w1440 -> [_ w1491]
              frame False {
              }
              frame True {
                n748 = Read from Text File(file (use dialog)=w1491) -> (text=w1495:string)  [unwired: 3 in, 3 out]
                n749 = property on="Image Out" class="ImageControl"() -> ("ROI"=w1492:T10)  [unwired: 2 in, 2 out]
                n750 = Unflatten From String(type=w1492, binary string=w1495) -> (value=w1493:T10, error out=w1494:errorcluster)  [unwired: 3 in, 1 out]
                n751 = property on="Image Out" class="ImageControl"(error in=w1494, "ROI"=w1493) -> ()  [unwired: 1 in, 2 out]
              }
            }
            n752 = Index Array(array=w1470, index=w1469) -> (element=w1443:string)
            n753 = local write "Image Name"(w1443) -> ()
            n754 = Empty String/Path?(string/path=w1443) -> (empty?=w1450:bool)
            n755 = Build Path(base path=w1427, name or relative path=w1443) -> (appended path=w1442:path)
            n756 = local read "No Image File"() -> (w1449:path)
            n757 = Select(t=w1449, s=w1450, f=w1442) -> (s? t:f=w1444:path)
            n758 = call <vilib>:"Get File Extension.vi"("file"=w1444) -> ("lowercase file extension"=w1446:string)  [unwired: 7 in, 3 out]
            n759 = local write "Image File"(w1444) -> ()
            n760 = local write "String"(w1446) -> ()
            n761 = Search 1D Array(1D array=string[] ["bmp", "jpeg", "png", "jpg", "gif"], element=w1446) -> (index of element=w1445:i32)  [unwired: 1 in]
            n762 = call "Vision Acquisition5"("Image Path"=w1444) -> ("Image Out"=w1448:T2)  [unwired: 25 in, 1 out]
            n763 = Less Than 0?(x=w1445) -> ()  [unwired: 1 out]
            n764 = local write "Image Out"(w1448) -> ()
            n765 = local write "Image Out 2"(w1448) -> ()
          }
          event "Save Changes? 3": Mouse Down {
            n766 = event-data() -> ()  [unwired: 1 in, 7 out]
            n767 = local read "Image Folder"() -> (w1620:path)
            n768 = Build Path(base path=w1620, name or relative path="ROI") -> (appended path=w1627:path)
            n769 = call <vilib>:"Check if File or Folder Exists.vi"("path"=w1627) -> ("file or folder exists?"=w1629:bool, "dup path"=w1626:path)  [unwired: 8 in, 1 out]
            n770 = case shown="False" w1629 {
              tunnel: w1626 -> [w1631 w1632]
              tunnel: [w1630 w1632] -> w1621
              frame False {
                n771 = Create Folder(path (use dialog)=w1631) -> (created path=w1630:path)  [unwired: 2 in, 2 out]
              }
              frame True {
              }
            }
            n772 = local read "Index"() -> (w1623:string)
            n773 = property on="Image Out" class="ImageControl"() -> ("ROI"=w1625:T10)  [unwired: 2 in, 2 out]
            n774 = Build Path(base path=w1621, name or relative path=w1623) -> (appended path=w1622:path)
            n775 = Flatten To String(anything=w1625) -> (data string=w1624:string)  [unwired: 3 in, 2 out]
            n776 = Write to Text File(file (use dialog)=w1622, text=w1624) -> ()  [unwired: 2 in, 3 out]
          }
          event "Next Button": Mouse Down {
            n777 = event-data() -> ()  [unwired: 1 in, 5 out]
            n778 = local read "XY Graph"() -> (w1645:cluster{dbl[], dbl[]}[])
            n779 = Decimate 1D Array(w1645) -> (w1641:cluster{dbl[], dbl[]}[], w1640:cluster{dbl[], dbl[]}[])
            n780 = Array To Cluster(array=w1641) -> (cluster=w1651:T9)
            n781 = local read "MobVi Index"() -> (w1647:dbl)
            n782 = Unbundle(w1651) -> ("[0]"=w1650:cluster{dbl[], dbl[]})  [unwired: 8 out]
            n783 = local read "NumPts"() -> (w1646:dbl)
            n784 = Unbundle(w1650) -> (w1649:dbl[], w1648:dbl[])
            n785 = Increment(x=w1647) -> (x+1=w1642:dbl)
            n786 = local read "New: Dielectric"() -> (w1636:dbl)
            n787 = local read "New: Length"() -> (w1635:dbl)
            n788 = local read "New: Width"() -> (w1634:dbl)
            n789 = local write "MobVi Index"(w1642) -> ()
            n790 = Array Subset(array=w1649, index=w1642, length=w1646) -> (w1638:dbl[])
            n791 = Array Subset(array=w1648, index=w1642, length=w1646) -> (w1637:dbl[])
            n792 = local write "Sat Vg Array-Used"(w1638) -> ()
            n793 = local write "Sat Id-Used"(w1637) -> ()
            n794 = call "Mobility-Vt-Used Pts_Saturation.vi"("Width"=w1634, "Length"=w1635, "Dielectric (d)"=w1636, "Sat Id Used"=w1637, "Vg Used"=w1638) -> ("Vt"=w1633:dbl, "Mobility"=w1639:dbl)  [unwired: 4 in, 1 out]
            n795 = Bundle(w1638, w1637) -> (w1644:cluster{dbl[], dbl[]})  [unwired: 1 in]
            n796 = Build Array (concatenate)(w1641, w1640, w1644) -> (w1643:cluster{dbl[], dbl[]}[])
            n797 = local write "New: Mobility-Sat"(w1639) -> ()
            n798 = local write "New: VT-Sat"(w1633) -> ()
            n799 = local write "XY Graph"(w1643) -> ()
          }
          event "Next Button 2": Mouse Down {
            n800 = event-data() -> ()  [unwired: 1 in, 7 out]
            n801 = local read "XY Graph 2"() -> (w1660:cluster{dbl[], dbl[]}[])
            n802 = Decimate 1D Array(w1660) -> (w1656:cluster{dbl[], dbl[]}[], w1655:cluster{dbl[], dbl[]}[])
            n803 = Array To Cluster(array=w1656) -> (cluster=w1666:T9)
            n804 = local read "Index 2"() -> (w1662:dbl)
            n805 = Unbundle(w1666) -> ("[0]"=w1665:cluster{dbl[], dbl[]})  [unwired: 8 out]
            n806 = local read "NumPts 2"() -> (w1661:dbl)
            n807 = Unbundle(w1665) -> (w1664:dbl[], w1663:dbl[])
            n808 = Increment(x=w1662) -> (x+1=w1657:dbl)
            n809 = local write "Index 2"(w1657) -> ()
            n810 = Array Subset(array=w1663, index=w1657, length=w1661) -> (w1652:dbl[])
            n811 = Array Subset(array=w1664, index=w1657, length=w1661) -> (w1653:dbl[])
            n812 = call "STS-Used.vi"("Id Used"=w1653, "Vg-Used"=w1652) -> ("STS"=w1654:dbl)  [unwired: 9 in]
            n813 = Bundle(w1653, w1652) -> (w1659:cluster{dbl[], dbl[]})  [unwired: 1 in]
            n814 = local write "Vg Array-Log-Used"(w1652) -> ()
            n815 = local write "Sat Id-Log-Used"(w1653) -> ()
            n816 = local write "New: STS"(w1654) -> ()
            n817 = Build Array (concatenate)(w1656, w1655, w1659) -> (w1658:cluster{dbl[], dbl[]}[])
            n818 = local write "XY Graph 2"(w1658) -> ()
          }
          event "Previous Button 2": Mouse Down {
            n819 = event-data() -> ()  [unwired: 1 in, 7 out]
            n820 = local read "XY Graph 2"() -> (w1676:cluster{dbl[], dbl[]}[])
            n821 = Decimate 1D Array(w1676) -> (w1673:cluster{dbl[], dbl[]}[], w1672:cluster{dbl[], dbl[]}[])
            n822 = Array To Cluster(array=w1673) -> (cluster=w1681:T9)
            n823 = local read "Index 2"() -> (w1669:dbl)
            n824 = Unbundle(w1681) -> ("[0]"=w1680:cluster{dbl[], dbl[]})  [unwired: 8 out]
            n825 = local read "NumPts 2"() -> (w1677:dbl)
            n826 = Unbundle(w1680) -> (w1679:dbl[], w1678:dbl[])
            n827 = Decrement(x=w1669) -> (x-1=w1670:dbl)
            n828 = local write "Index 2"(w1670) -> ()
            n829 = Array Subset(array=w1679, index=w1670, length=w1677) -> (w1667:dbl[])
            n830 = Array Subset(array=w1678, index=w1670, length=w1677) -> (w1668:dbl[])
            n831 = local write "Vg Array-Log-Used"(w1668) -> ()
            n832 = local write "Sat Id-Log-Used"(w1667) -> ()
            n833 = Bundle(w1667, w1668) -> (w1675:cluster{dbl[], dbl[]})  [unwired: 1 in]
            n834 = call "STS-Used.vi"("Id Used"=w1667, "Vg-Used"=w1668) -> ("STS"=w1671:dbl)  [unwired: 9 in]
            n835 = Build Array (concatenate)(w1673, w1672, w1675) -> (w1674:cluster{dbl[], dbl[]}[])
            n836 = local write "New: STS"(w1671) -> ()
            n837 = local write "XY Graph 2"(w1674) -> ()
          }
          event "Previous Button": Mouse Down {
            n838 = event-data() -> ()  [unwired: 1 in, 5 out]
            n839 = local read "XY Graph"() -> (w1695:cluster{dbl[], dbl[]}[])
            n840 = Decimate 1D Array(w1695) -> (w1692:cluster{dbl[], dbl[]}[], w1691:cluster{dbl[], dbl[]}[])
            n841 = Array To Cluster(array=w1692) -> (cluster=w1700:T9)
            n842 = local read "MobVi Index"() -> (w1690:dbl)
            n843 = Unbundle(w1700) -> ("[0]"=w1699:cluster{dbl[], dbl[]})  [unwired: 8 out]
            n844 = local read "NumPts"() -> (w1696:dbl)
            n845 = Unbundle(w1699) -> (w1698:dbl[], w1697:dbl[])
            n846 = Decrement(x=w1690) -> (x-1=w1689:dbl)
            n847 = local read "New: Dielectric"() -> (w1683:dbl)
            n848 = local read "New: Length"() -> (w1684:dbl)
            n849 = local read "New: Width"() -> (w1685:dbl)
            n850 = local write "MobVi Index"(w1689) -> ()
            n851 = Array Subset(array=w1698, index=w1689, length=w1696) -> (w1688:dbl[])
            n852 = Array Subset(array=w1697, index=w1689, length=w1696) -> (w1687:dbl[])
            n853 = local write "Sat Vg Array-Used"(w1688) -> ()
            n854 = local write "Sat Id-Used"(w1687) -> ()
            n855 = call "Mobility-Vt-Used Pts_Linear.vi"("Width"=w1685, "Length"=w1684, "Dielectric (d)"=w1683, "Sat Id Used"=w1687, "Vg Used"=w1688) -> ("Vt"=w1682:dbl, "Mobility"=w1686:dbl)  [unwired: 4 in, 1 out]
            n856 = Bundle(w1688, w1687) -> (w1694:cluster{dbl[], dbl[]})  [unwired: 1 in]
            n857 = local write "New: VT-Sat"(w1682) -> ()
            n858 = Build Array (concatenate)(w1692, w1691, w1694) -> (w1693:cluster{dbl[], dbl[]}[])
            n859 = local write "New: Mobility-Sat"(w1686) -> ()
            n860 = local write "XY Graph"(w1693) -> ()
          }
          event "Slide": Value Change {
            n861 = event-data() -> ()  [unwired: 1 in, 5 out]
            n862 = local read "XY Graph"() -> (w1713:cluster{dbl[], dbl[]}[])
            n863 = Decimate 1D Array(w1713) -> (w1710:cluster{dbl[], dbl[]}[], w1709:cluster{dbl[], dbl[]}[])
            n864 = Array To Cluster(array=w1710) -> (cluster=w1718:T9)
            n865 = Unbundle(w1718) -> ("[0]"=w1717:cluster{dbl[], dbl[]})  [unwired: 8 out]
            n866 = local read "NumPts"() -> (w1714:dbl)
            n867 = local read "Slide"() -> (w1702:dbl)
            n868 = Unbundle(w1717) -> (w1716:dbl[], w1715:dbl[])
            n869 = local read "New: Dielectric"() -> (w1703:dbl)
            n870 = local read "New: Length"() -> (w1704:dbl)
            n871 = local read "New: Width"() -> (w1705:dbl)
            n872 = local write "MobVi Index"(w1702) -> ()
            n873 = Array Subset(array=w1716, index=w1702, length=w1714) -> (w1708:dbl[])
            n874 = Array Subset(array=w1715, index=w1702, length=w1714) -> (w1707:dbl[])
            n875 = local write "Sat Vg Array-Used"(w1708) -> ()
            n876 = local write "Sat Id-Used"(w1707) -> ()
            n877 = call "Mobility-Vt-Used Pts_Linear.vi"("Width"=w1705, "Length"=w1704, "Dielectric (d)"=w1703, "Sat Id Used"=w1707, "Vg Used"=w1708) -> ("Vt"=w1701:dbl, "Mobility"=w1706:dbl)  [unwired: 4 in, 1 out]
            n878 = Bundle(w1708, w1707) -> (w1712:cluster{dbl[], dbl[]})  [unwired: 1 in]
            n879 = local write "New: VT-Sat"(w1701) -> ()
            n880 = Build Array (concatenate)(w1710, w1709, w1712) -> (w1711:cluster{dbl[], dbl[]}[])
            n881 = local write "New: Mobility-Sat"(w1706) -> ()
            n882 = local write "XY Graph"(w1711) -> ()
          }
          event "Slide 2": Value Change {
            n883 = event-data() -> ()  [unwired: 1 in, 5 out]
            n884 = local read "XY Graph 2"() -> (w1727:cluster{dbl[], dbl[]}[])
            n885 = Decimate 1D Array(w1727) -> (w1724:cluster{dbl[], dbl[]}[], w1723:cluster{dbl[], dbl[]}[])
            n886 = Array To Cluster(array=w1724) -> (cluster=w1732:T9)
            n887 = Unbundle(w1732) -> ("[0]"=w1731:cluster{dbl[], dbl[]})  [unwired: 8 out]
            n888 = local read "NumPts 2"() -> (w1728:dbl)
            n889 = local read "Slide 2"() -> (w1722:dbl)
            n890 = Unbundle(w1731) -> (w1730:dbl[], w1729:dbl[])
            n891 = local write "Index 2"(w1722) -> ()
            n892 = Array Subset(array=w1730, index=w1722, length=w1728) -> (w1720:dbl[])
            n893 = Array Subset(array=w1729, index=w1722, length=w1728) -> (w1719:dbl[])
            n894 = local write "Vg Array-Log-Used"(w1719) -> ()
            n895 = local write "Sat Id-Log-Used"(w1720) -> ()
            n896 = call "STS-Used.vi"("Id Used"=w1720, "Vg-Used"=w1719) -> ("STS"=w1721:dbl)  [unwired: 9 in]
            n897 = Bundle(w1720, w1719) -> (w1726:cluster{dbl[], dbl[]})  [unwired: 1 in]
            n898 = local write "New: STS"(w1721) -> ()
            n899 = Build Array (concatenate)(w1724, w1723, w1726) -> (w1725:cluster{dbl[], dbl[]}[])
            n900 = local write "XY Graph 2"(w1725) -> ()
          }
          event "Save Changes?": Mouse Down {
            n901 = event-data() -> ()  [unwired: 1 in, 5 out]
            n902 = flat-sequence {
              tunnel: [w1739] -> w1737
              tunnel: [w1747] -> w1736
              tunnel: [w1740] -> w1735
              tunnel: w1737 -> [w2256]
              tunnel: w1736 -> [w2253]
              tunnel: [w2254] -> w1734
              tunnel: w1735 -> [w2254]
              tunnel: [w2253] -> w1733
              tunnel: w1734 -> [w2261]
              tunnel: w1733 -> [w2260]
              frame #0 {
                n903 = Wait (ms)(milliseconds to wait=1) -> ()  [unwired: 1 out]
              }
              frame #1 {
                n904 = local read "Transfer File"() -> (w1739:path)
                n905 = local read "New: Temp"() -> (w1741:dbl)
                n906 = local read "New: Length"() -> (w1745:dbl)
                n907 = local read "New: Width"() -> (w1743:dbl)
                n908 = To Single Precision Float(number=w1741) -> (single precision float=w1742:sgl)
                n909 = Number To Decimal String(number=w1742) -> (decimal integer string=w1750:string)  [unwired: 1 in]
                n910 = To Single Precision Float(number=w1743) -> (single precision float=w1744:sgl)
                n911 = To Single Precision Float(number=w1745) -> (single precision float=w1746:sgl)
                n912 = local read "Index"() -> (w1755:string)
                n913 = Strip Path(path=w1739) -> (stripped path=w1760:path)  [unwired: 1 out]
                n914 = Number To Decimal String(number=w1746) -> (decimal integer string=w1753:string)  [unwired: 1 in]
                n915 = Number To Decimal String(number=w1744) -> (decimal integer string=w1754:string)  [unwired: 1 in]
                n916 = Concatenate Strings("_", w1750, "K") -> (w1748:string)
                n917 = call "Build Text"("Temp"=w1748, "Index"=w1755, "Length"=w1753, "Width"=w1754) -> ("Result"=w1756:string)  [unwired: 10 in, 1 out]
                n918 = flat-sequence {
                  tunnel: [w2210] -> w1752
                  tunnel: w1752 -> [w2227]
                  frame #0 {
                    # "Makes Empty File for Transformer Data"
                    n919 = local read "Transfer Folder"() -> (w2199:path)
                    n920 = Build Path(base path=w2199, name or relative path="Stats") -> (appended path=w2201:path)
                    n921 = call <vilib>:"Check if File or Folder Exists.vi"("path"=w2201) -> ("file or folder exists?"=w2202:bool, "dup path"=w2203:path)  [unwired: 8 in, 1 out]
                    n922 = case shown="False" w2202 {
                      tunnel: [w2207 w2209] -> w2204
                      tunnel: w2203 -> [w2208 w2209]
                      frame False {
                        n923 = Create Folder(path (use dialog)=w2208) -> (created path=w2207:path)  [unwired: 2 in, 2 out]
                      }
                      frame True {
                      }
                    }
                    n924 = Build Path(base path=w2204, name or relative path="Tranformer Data.txt") -> (appended path=w2206:path)
                    n925 = call-poly <vilib>:"Write To Spreadsheet File.vi"("append to file? (new file:F)"=TRUE, "file path (dialog if empty)"=w2206) -> ()  [unwired: 6 in, 1 out]
                  }
                  frame #1 {
                    # "Adds Headers if they don't exist"
                    n926 = local read "Transfer Folder"() -> (w2216:path)
                    n927 = Concatenate Strings("Stats\\", "Tranformer Data.txt") -> (w2217:string)
                    n928 = Build Path(base path=w2216, name or relative path=w2217) -> (appended path=w2210:path)
                    n929 = call-poly <vilib>:"Read From Spreadsheet File.vi"("file path (dialog if empty)"=w2210) -> ("first row"=w2215:string[])  [unwired: 6 in, 4 out]
                    n930 = Search 1D Array(1D array=w2215, element="DeviceID") -> (index of element=w2213:i32)  [unwired: 1 in]
                    n931 = Equal?(x=w2213, y=0) -> (x = y?=w2211:bool)
                    n932 = case shown="False" w2211 {
                      tunnel: w2210 -> [w2221 _]
                      frame False {
                        n933 = local read "Transformer \nHeaders"() -> (w2220:string[])
                        n934 = call-poly <vilib>:"Write To Spreadsheet File.vi"("1D data"=w2220, "file path (dialog if empty)"=w2221) -> ()  [unwired: 6 in, 1 out]
                      }
                      frame True {
                      }
                    }
                  }
                  frame #2 {
                    # "Adds current device if it doesn't exist"
                    n935 = local read "Current \nRecord"() -> (w2226:string[])
                    n936 = Index Array(array=w2226, index=0) -> (element=w2225:string)
                    n937 = local read "Transfer Folder"() -> (w2229:path)
                    n938 = Concatenate Strings("Stats\\", "Tranformer Data.txt") -> (w2230:string)
                    n939 = local write "Current Device ID"(w2225) -> ()
                    n940 = local read "Current Device ID"() -> (w2235:string)
                    n941 = Build Path(base path=w2229, name or relative path=w2230) -> (appended path=w2228:path)
                    n942 = call-poly <vilib>:"Read From Spreadsheet File.vi"("file path (dialog if empty)"=w2228) -> ("all rows"=w2222:string[][])  [unwired: 6 in, 4 out]
                    n943 = Index Array(array=w2222, index (col)=0) -> (element=w2223:string[])  [unwired: 1 in]
                    n944 = Search 1D Array(1D array=w2223, element=w2235) -> (index of element=w2224:i32)  [unwired: 1 in]
                    n945 = Equal?(x=w2224, y=-1) -> (x = y?=w2237:bool)
                    n946 = case shown="False" w2237 {
                      tunnel: w2227 -> [w2240 w2251]
                      tunnel: w2224 -> [w2243 _]
                      tunnel: w2222 -> [w2244 _]
                      frame False {
                        n947 = local read "Current \nRecord"() -> (w2242:string[])
                        n948 = Replace Array Subset(array=w2244, new element=w2242, index (row)=w2243) -> (w2241:string[][])  [unwired: 1 in]
                        n949 = flat-sequence {
                          tunnel: w2240 -> [w2245]
                          tunnel: w2241 -> [w2246]
                          tunnel: [w2246] -> w2239
                          tunnel: [w2245] -> w2238
                          tunnel: w2239 -> [w2248]
                          tunnel: w2238 -> [w2247]
                          frame #0 {
                            n950 = Delete(path (use dialog)=w2245) -> ()  [unwired: 4 in, 3 out]
                          }
                          frame #1 {
                            n951 = call-poly <vilib>:"Write To Spreadsheet File.vi"("append to file? (new file:F)"=TRUE, "2D data"=w2248, "file path (dialog if empty)"=w2247) -> ()  [unwired: 5 in, 1 out]
                          }
                        }
                      }
                      frame True {
                        n952 = local read "Current \nRecord"() -> (w2250:string[])
                        n953 = call-poly <vilib>:"Write To Spreadsheet File.vi"("append to file? (new file:F)"=TRUE, "1D data"=w2250, "file path (dialog if empty)"=w2251) -> ()  [unwired: 5 in, 1 out]
                      }
                    }
                  }
                }
                n954 = Path To String(path=w1760) -> (string=w1758:string)
                n955 = stacked-sequence {
                  tunnel: [_ _ _ _ _ _ _ _ _ _ _ _ w2170] -> w1740
                  tunnel: w1739 -> [w1762 _ _ _ _ _ _ _ _ _ _ _ _]
                  frame #0 {
                    n956 = call-poly <vilib>:"Read From Spreadsheet File.vi"("file path (dialog if empty)"=w1762) -> ("all rows"=w1761:string[][])  [unwired: 6 in, 4 out]
                    n957 = Array Size(array=w1761) -> (size(s)=w1766:i32[])
                    n958 = Array Subset(array=w1761, index (row)=0, index (col)=0, length (col)=3) -> (w1770:string[][])  [unwired: 1 in]
                    n959 = Index Array(array=w1766, index=0) -> (element=w1764:i32)
                    n960 = Reshape Array(w1770, w1764) -> (w1763:string[])
                    n961 = Search 1D Array(1D array=w1763, element="Dielectric (nm):") -> (index of element=w1773:i32)  [unwired: 1 in]
                    n962 = Equal?(x=w1773, y=-1) -> (x = y?=w1772:bool)
                    n963 = case shown="False" w1772 {
                      tunnel: w1761 -> [w1781 w1785]
                      tunnel: w1773 -> [w1777 _]
                      tunnel: [w1776 w1785] -> w1771
                      frame False {
                        n964 = local read "New: Dielectric"() -> (w1783:dbl)
                        n965 = Number To Fractional String(number=w1783) -> (F-format string=w1778:string)  [unwired: 3 in]
                        n966 = Divide(x=w1777, y=3) -> (x/y=w1780:dbl)
                        n967 = To Word Integer(number=w1780) -> (16bit integer=w1779:i16)
                        n968 = Replace Array Subset(array=w1781, new element=w1778, index (row)=w1779, index (col)=1) -> (w1776:string[][])
                      }
                      frame True {
                      }
                    }
                    n969 = local write "Save1 Array"(w1771) -> ()
                  }
                  frame #1 {
                    n970 = local read "Save1 Array"() -> (w1787:string[][])
                    n971 = Array Size(array=w1787) -> (size(s)=w1790:i32[])
                    n972 = Array Subset(array=w1787, index (row)=0, index (col)=0, length (col)=3) -> (w1794:string[][])  [unwired: 1 in]
                    n973 = Index Array(array=w1790, index=0) -> (element=w1788:i32)
                    n974 = Reshape Array(w1794, w1788) -> (w1786:string[])
                    n975 = Search 1D Array(1D array=w1786, element="Length (um):") -> (index of element=w1797:i32)  [unwired: 1 in]
                    n976 = Equal?(x=w1797, y=-1) -> (x = y?=w1796:bool)
                    n977 = case shown="False" w1796 {
                      tunnel: w1787 -> [w1807 w1810]
                      tunnel: w1797 -> [w1804 _]
                      tunnel: [w1803 w1810] -> w1795
                      frame False {
                        n978 = local read "New: Length"() -> (w1800:dbl)
                        n979 = Divide(x=w1804, y=3) -> (x/y=w1806:dbl)
                        n980 = Format Value(format string="%#g", value (0)=w1800) -> (output string=w1801:string)  [unwired: 1 in]
                        n981 = To Word Integer(number=w1806) -> (16bit integer=w1805:i16)
                        n982 = Replace Array Subset(array=w1807, new element=w1801, index (row)=w1805, index (col)=1) -> (w1803:string[][])
                      }
                      frame True {
                      }
                    }
                    n983 = local write "Save1 Array"(w1795) -> ()
                  }
                  frame #2 {
                    n984 = local read "Save1 Array"() -> (w1812:string[][])
                    n985 = Array Size(array=w1812) -> (size(s)=w1817:i32[])
                    n986 = Array Subset(array=w1812, index (row)=0, index (col)=0, length (col)=3) -> (w1813:string[][])  [unwired: 1 in]
                    n987 = Index Array(array=w1817, index=0) -> (element=w1819:i32)
                    n988 = Reshape Array(w1813, w1819) -> (w1811:string[])
                    n989 = Search 1D Array(1D array=w1811, element="Width (um):") -> (index of element=w1822:i32)  [unwired: 1 in]
                    n990 = Equal?(x=w1822, y=-1) -> (x = y?=w1821:bool)
                    n991 = case shown="False" w1821 {
                      tunnel: w1822 -> [w1830 _]
                      tunnel: w1812 -> [w1829 w1835]
                      tunnel: [w1828 w1835] -> w1820
                      frame False {
                        n992 = local read "New: Width"() -> (w1825:dbl)
                        n993 = Divide(x=w1830, y=3) -> (x/y=w1832:dbl)
                        n994 = To Word Integer(number=w1832) -> (16bit integer=w1831:i16)
                        n995 = Format Value(format string="%#g", value (0)=w1825) -> (output string=w1826:string)  [unwired: 1 in]
                        n996 = Replace Array Subset(array=w1829, new element=w1826, index (row)=w1831, index (col)=1) -> (w1828:string[][])
                      }
                      frame True {
                      }
                    }
                    n997 = local write "Save1 Array"(w1820) -> ()
                  }
                  frame #3 {
                    w1845 = "Sample Temp (K):"
                    n998 = local read "Save1 Array"() -> (w1837:string[][])
                    n999 = Array Size(array=w1837) -> (size(s)=w1842:i32[])
                    n1000 = Array Subset(array=w1837, index (row)=0, index (col)=0, length (col)=3) -> (w1838:string[][])  [unwired: 1 in]
                    n1001 = Index Array(array=w1842, index=0) -> (element=w1844:i32)
                    n1002 = Reshape Array(w1838, w1844) -> (w1836:string[])
                    n1003 = Search 1D Array(1D array=w1836, element=w1845) -> (index of element=w1848:i32)  [unwired: 1 in]
                    n1004 = Equal?(x=w1848, y=-1) -> (x = y?=w1847:bool)
                    n1005 = case shown="True" w1847 {
                      tunnel: w1837 -> [w1857 w1871]
                      tunnel: w1848 -> [w1854 _]
                      tunnel: [w1853 w1870] -> w1846
                      tunnel: w1836 -> [_ w1873]
                      tunnel: w1845 -> [_ w1860]
                      frame False {
                        n1006 = local read "New: Temp"() -> (w1851:dbl)
                        n1007 = Divide(x=w1854, y=3) -> (x/y=w1856:dbl)
                        n1008 = Format Value(format string="%#g", value (0)=w1851) -> (output string=w1850:string)  [unwired: 1 in]
                        n1009 = To Word Integer(number=w1856) -> (16bit integer=w1855:i16)
                        n1010 = Replace Array Subset(array=w1857, new element=w1850, index (row)=w1855, index (col)=1) -> (w1853:string[][])
                      }
                      frame True {
                        n1011 = local read "New: Temp"() -> (w1862:dbl)
                        n1012 = Search 1D Array(1D array=w1873, element="Width (um):") -> (index of element=w1867:i32)  [unwired: 1 in]
                        n1013 = Divide(x=w1867, y=3) -> (x/y=w1868:dbl)
                        n1014 = To Word Integer(number=w1868) -> (16bit integer=w1866:i16)
                        n1015 = Format Value(format string="%#g", value (0)=w1862) -> (output string=w1861:string)  [unwired: 1 in]
                        n1016 = Build Array(w1860, w1861) -> (w1864:string[])
                        n1017 = Increment(x=w1866) -> (x+1=w1865:i16)
                        n1018 = Insert Into Array(array=w1871, index (row)=w1865, new element=w1864) -> (w1870:string[][])  [unwired: 1 in]
                      }
                    }
                    n1019 = local write "Save1 Array"(w1846) -> ()
                  }
                  frame #4 {
                    w1883 = "Mobility-Sat (cm^2/Vs):"
                    n1020 = local read "Save1 Array"() -> (w1875:string[][])
                    n1021 = Array Size(array=w1875) -> (size(s)=w1880:i32[])
                    n1022 = Array Subset(array=w1875, index (row)=0, index (col)=0, length (col)=3) -> (w1876:string[][])  [unwired: 1 in]
                    n1023 = Index Array(array=w1880, index=0) -> (element=w1882:i32)
                    n1024 = Reshape Array(w1876, w1882) -> (w1874:string[])
                    n1025 = Search 1D Array(1D array=w1874, element=w1883) -> (index of element=w1886:i32)  [unwired: 1 in]
                    n1026 = Equal?(x=w1886, y=-1) -> (x = y?=w1885:bool)
                    n1027 = case shown="True" w1885 {
                      tunnel: w1875 -> [w1895 w1903]
                      tunnel: w1886 -> [w1892 _]
                      tunnel: [w1891 w1902] -> w1884
                      tunnel: w1874 -> [_ w1900]
                      tunnel: w1883 -> [_ w1898]
                      frame False {
                        n1028 = local read "New: Mobility-Sat"() -> (w1888:dbl)
                        n1029 = Divide(x=w1892, y=3) -> (x/y=w1894:dbl)
                        n1030 = To Word Integer(number=w1894) -> (16bit integer=w1893:i16)
                        n1031 = Format Value(format string="%#g", value (0)=w1888) -> (output string=w1889:string)  [unwired: 1 in]
                        n1032 = Replace Array Subset(array=w1895, new element=w1889, index (row)=w1893, index (col)=1) -> (w1891:string[][])
                      }
                      frame True {
                        n1033 = local read "New: Mobility-Sat"() -> (w1904:dbl)
                        n1034 = Search 1D Array(1D array=w1900, element="Mobility (cm^2/Vs):") -> (index of element=w1907:i32)  [unwired: 1 in]
                        n1035 = Divide(x=w1907, y=3) -> (x/y=w1908:dbl)
                        n1036 = To Word Integer(number=w1908) -> (16bit integer=w1899:i16)
                        n1037 = Format Value(format string="%#g", value (0)=w1904) -> (output string=w1901:string)  [unwired: 1 in]
                        n1038 = Build Array(w1898, w1901) -> (w1906:string[])
                        n1039 = Replace Array Subset(array=w1903, new element=w1906, index (row)=w1899) -> (w1902:string[][])  [unwired: 1 in]
                      }
                    }
                    n1040 = local write "Save1 Array"(w1884) -> ()
                  }
                  frame #5 {
                    w1920 = "Mobility-Lin (cm^2/Vs):"
                    n1041 = local read "Save1 Array"() -> (w1911:string[][])
                    n1042 = Array Size(array=w1911) -> (size(s)=w1917:i32[])
                    n1043 = Array Subset(array=w1911, index (row)=0, index (col)=0, length (col)=3) -> (w1913:string[][])  [unwired: 1 in]
                    n1044 = Index Array(array=w1917, index=0) -> (element=w1919:i32)
                    n1045 = Reshape Array(w1913, w1919) -> (w1912:string[])
                    n1046 = Search 1D Array(1D array=w1912, element=w1920) -> (index of element=w1923:i32)  [unwired: 1 in]
                    n1047 = Equal?(x=w1923, y=-1) -> (x = y?=w1922:bool)
                    n1048 = case shown="True" w1922 {
                      tunnel: w1911 -> [w1932 w1938]
                      tunnel: w1923 -> [w1929 _]
                      tunnel: [w1928 w1937] -> w1921
                      tunnel: w1912 -> [_ w1936]
                      tunnel: w1920 -> [_ w1935]
                      frame False {
                        n1049 = local read "Calc: Mobility-Lin"() -> (w1925:dbl)
                        n1050 = Divide(x=w1929, y=3) -> (x/y=w1931:dbl)
                        n1051 = To Word Integer(number=w1931) -> (16bit integer=w1930:i16)
                        n1052 = Format Value(format string="%#g", value (0)=w1925) -> (output string=w1926:string)  [unwired: 1 in]
                        n1053 = Replace Array Subset(array=w1932, new element=w1926, index (row)=w1930, index (col)=1) -> (w1928:string[][])
                      }
                      frame True {
                        n1054 = local read "Calc: Mobility-Lin"() -> (w1939:dbl)
                        n1055 = Search 1D Array(1D array=w1936, element="Mobility-Sat (cm^2/Vs):") -> (index of element=w1944:i32)  [unwired: 1 in]
                        n1056 = Divide(x=w1944, y=3) -> (x/y=w1945:dbl)
                        n1057 = To Word Integer(number=w1945) -> (16bit integer=w1943:i16)
                        n1058 = Format Value(format string="%#g", value (0)=w1939) -> (output string=w1948:string)  [unwired: 1 in]
                        n1059 = Build Array(w1935, w1948) -> (w1941:string[])
                        n1060 = Increment(x=w1943) -> (x+1=w1942:i16)
                        n1061 = Insert Into Array(array=w1938, index (row)=w1942, new element=w1941) -> (w1937:string[][])  [unwired: 1 in]
                      }
                    }
                    n1062 = local write "Save1 Array"(w1921) -> ()
                  }
                  frame #6 {
                    w1958 = "On/Off I-Sat:"
                    n1063 = local read "Save1 Array"() -> (w1949:string[][])
                    n1064 = Array Size(array=w1949) -> (size(s)=w1955:i32[])
                    n1065 = Array Subset(array=w1949, index (row)=0, index (col)=0, length (col)=3) -> (w1951:string[][])  [unwired: 1 in]
                    n1066 = Index Array(array=w1955, index=0) -> (element=w1957:i32)
                    n1067 = Reshape Array(w1951, w1957) -> (w1950:string[])
                    n1068 = Search 1D Array(1D array=w1950, element=w1958) -> (index of element=w1961:i32)  [unwired: 1 in]
                    n1069 = Equal?(x=w1961, y=-1) -> (x = y?=w1960:bool)
                    n1070 = case shown="True" w1960 {
                      tunnel: w1949 -> [w1970 w1977]
                      tunnel: w1961 -> [w1967 _]
                      tunnel: [w1966 w1978] -> w1959
                      tunnel: w1950 -> [_ w1975]
                      tunnel: w1958 -> [_ w1973]
                      frame False {
                        n1071 = local read "Calc: On/Off"() -> (w1963:dbl)
                        n1072 = Divide(x=w1967, y=3) -> (x/y=w1969:dbl)
                        n1073 = To Word Integer(number=w1969) -> (16bit integer=w1968:i16)
                        n1074 = Format Value(format string="%#g", value (0)=w1963) -> (output string=w1964:string)  [unwired: 1 in]
                        n1075 = Replace Array Subset(array=w1970, new element=w1964, index (row)=w1968, index (col)=1) -> (w1966:string[][])
                      }
                      frame True {
                        n1076 = local read "Calc: On/Off"() -> (w1979:dbl)
                        n1077 = Search 1D Array(1D array=w1975, element="On/Off Current:") -> (index of element=w1982:i32)  [unwired: 1 in]
                        n1078 = Divide(x=w1982, y=3) -> (x/y=w1983:dbl)
                        n1079 = To Word Integer(number=w1983) -> (16bit integer=w1974:i16)
                        n1080 = Format Value(format string="%#g", value (0)=w1979) -> (output string=w1976:string)  [unwired: 1 in]
                        n1081 = Build Array(w1973, w1976) -> (w1981:string[])
                        n1082 = Replace Array Subset(array=w1977, new element=w1981, index (row)=w1974) -> (w1978:string[][])  [unwired: 1 in]
                      }
                    }
                    n1083 = local write "Save1 Array"(w1959) -> ()
                  }
                  frame #7 {
                    w1995 = "Off I-Sat (A):"
                    n1084 = local read "Save1 Array"() -> (w1986:string[][])
                    n1085 = Array Size(array=w1986) -> (size(s)=w1992:i32[])
                    n1086 = Array Subset(array=w1986, index (row)=0, index (col)=0, length (col)=3) -> (w1988:string[][])  [unwired: 1 in]
                    n1087 = Index Array(array=w1992, index=0) -> (element=w1994:i32)
                    n1088 = Reshape Array(w1988, w1994) -> (w1987:string[])
                    n1089 = Search 1D Array(1D array=w1987, element=w1995) -> (index of element=w1998:i32)  [unwired: 1 in]
                    n1090 = Equal?(x=w1998, y=-1) -> (x = y?=w1997:bool)
                    n1091 = case shown="True" w1997 {
                      tunnel: w1986 -> [w2007 w2013]
                      tunnel: w1998 -> [w2004 _]
                      tunnel: [w2003 w2012] -> w1996
                      tunnel: w1987 -> [_ w2011]
                      tunnel: w1995 -> [_ w2010]
                      frame False {
                        n1092 = local read "Calc: Off I-Sat"() -> (w2002:dbl)
                        n1093 = Divide(x=w2004, y=3) -> (x/y=w2006:dbl)
                        n1094 = Format Value(format string="%#g", value (0)=w2002) -> (output string=w2000:string)  [unwired: 1 in]
                        n1095 = To Word Integer(number=w2006) -> (16bit integer=w2005:i16)
                        n1096 = Replace Array Subset(array=w2007, new element=w2000, index (row)=w2005, index (col)=1) -> (w2003:string[][])
                      }
                      frame True {
                        n1097 = local read "Calc: Off I-Sat"() -> (w2014:dbl)
                        n1098 = Search 1D Array(1D array=w2011, element="On/Off I-Sat:") -> (index of element=w2019:i32)  [unwired: 1 in]
                        n1099 = Divide(x=w2019, y=3) -> (x/y=w2020:dbl)
                        n1100 = To Word Integer(number=w2020) -> (16bit integer=w2018:i16)
                        n1101 = Format Value(format string="%#g", value (0)=w2014) -> (output string=w2023:string)  [unwired: 1 in]
                        n1102 = Build Array(w2010, w2023) -> (w2016:string[])
                        n1103 = Increment(x=w2018) -> (x+1=w2017:i16)
                        n1104 = Insert Into Array(array=w2013, index (row)=w2017, new element=w2016) -> (w2012:string[][])  [unwired: 1 in]
                      }
                    }
                    n1105 = local write "Save1 Array"(w1996) -> ()
                  }
                  frame #8 {
                    w2025 = "Vt-Sat (V):"
                    n1106 = local read "Save1 Array"() -> (w2026:string[][])
                    n1107 = Array Size(array=w2026) -> (size(s)=w2031:i32[])
                    n1108 = Array Subset(array=w2026, index (row)=0, index (col)=0, length (col)=3) -> (w2027:string[][])  [unwired: 1 in]
                    n1109 = Index Array(array=w2031, index=0) -> (element=w2033:i32)
                    n1110 = Reshape Array(w2027, w2033) -> (w2024:string[])
                    n1111 = Search 1D Array(1D array=w2024, element=w2025) -> (index of element=w2036:i32)  [unwired: 1 in]
                    n1112 = Equal?(x=w2036, y=-1) -> (x = y?=w2035:bool)
                    n1113 = case shown="True" w2035 {
                      tunnel: w2026 -> [w2043 w2052]
                      tunnel: w2036 -> [w2039 _]
                      tunnel: [w2038 w2051] -> w2034
                      tunnel: w2025 -> [_ w2050]
                      tunnel: w2024 -> [_ w2049]
                      frame False {
                        n1114 = local read "New: VT-Sat"() -> (w2045:dbl)
                        n1115 = Number To Fractional String(number=w2045) -> (F-format string=w2040:string)  [unwired: 3 in]
                        n1116 = Divide(x=w2039, y=3) -> (x/y=w2042:dbl)
                        n1117 = To Word Integer(number=w2042) -> (16bit integer=w2041:i16)
                        n1118 = Replace Array Subset(array=w2043, new element=w2040, index (row)=w2041, index (col)=1) -> (w2038:string[][])
                      }
                      frame True {
                        n1119 = local read "New: VT-Sat"() -> (w2053:dbl)
                        n1120 = Search 1D Array(1D array=w2049, element="Threshold V (V):") -> (index of element=w2048:i32)  [unwired: 1 in]
                        n1121 = Divide(x=w2048, y=3) -> (x/y=w2056:dbl)
                        n1122 = To Word Integer(number=w2056) -> (16bit integer=w2047:i16)
                        n1123 = Format Value(format string="%#g", value (0)=w2053) -> (output string=w2059:string)  [unwired: 1 in]
                        n1124 = Build Array(w2050, w2059) -> (w2055:string[])
                        n1125 = Replace Array Subset(array=w2052, new element=w2055, index (row)=w2047) -> (w2051:string[][])  [unwired: 1 in]
                      }
                    }
                    n1126 = local write "Save1 Array"(w2034) -> ()
                  }
                  frame #9 {
                    n1127 = local read "Save1 Array"() -> (w2060:string[][])
                    n1128 = Array Size(array=w2060) -> (size(s)=w2066:i32[])
                    n1129 = Array Subset(array=w2060, index (row)=0, index (col)=0, length (col)=3) -> (w2062:string[][])  [unwired: 1 in]
                    n1130 = Index Array(array=w2066, index=0) -> (element=w2068:i32)
                    n1131 = Reshape Array(w2062, w2068) -> (w2061:string[])
                    n1132 = Search 1D Array(1D array=w2061, element="VT-Lin (V):") -> (index of element=w2071:i32)  [unwired: 1 in]
                    n1133 = Equal?(x=w2071, y=-1) -> (x = y?=w2070:bool)
                    n1134 = case shown="False" w2070 {
                      tunnel: w2060 -> [w2081 w2084]
                      tunnel: w2071 -> [w2078 _]
                      tunnel: [w2077 w2084] -> w2069
                      frame False {
                        n1135 = local read "New: VT-Lin"() -> (w2075:dbl)
                        n1136 = Divide(x=w2078, y=3) -> (x/y=w2080:dbl)
                        n1137 = Format Value(format string="%#g", value (0)=w2075) -> (output string=w2074:string)  [unwired: 1 in]
                        n1138 = To Word Integer(number=w2080) -> (16bit integer=w2079:i16)
                        n1139 = Replace Array Subset(array=w2081, new element=w2074, index (row)=w2079, index (col)=1) -> (w2077:string[][])
                      }
                      frame True {
                      }
                    }
                    n1140 = local write "Save1 Array"(w2069) -> ()
                  }
                  frame #10 {
                    w2085 = "STS-Sat (V/decade):"
                    n1141 = local read "Save1 Array"() -> (w2087:string[][])
                    n1142 = Array Size(array=w2087) -> (size(s)=w2092:i32[])
                    n1143 = Array Subset(array=w2087, index (row)=0, index (col)=0, length (col)=3) -> (w2088:string[][])  [unwired: 1 in]
                    n1144 = Index Array(array=w2092, index=0) -> (element=w2094:i32)
                    n1145 = Reshape Array(w2088, w2094) -> (w2086:string[])
                    n1146 = Search 1D Array(1D array=w2086, element=w2085) -> (index of element=w2097:i32)  [unwired: 1 in]
                    n1147 = Equal?(x=w2097, y=-1) -> (x = y?=w2096:bool)
                    n1148 = case shown="True" w2096 {
                      tunnel: w2087 -> [w2106 w2112]
                      tunnel: w2097 -> [w2103 _]
                      tunnel: [w2102 w2113] -> w2095
                      tunnel: w2086 -> [_ w2111]
                      tunnel: w2085 -> [_ w2110]
                      frame False {
                        n1149 = local read "New: STS"() -> (w2100:dbl)
                        n1150 = Divide(x=w2103, y=3) -> (x/y=w2105:dbl)
                        n1151 = Format Value(format string="%#g", value (0)=w2100) -> (output string=w2099:string)  [unwired: 1 in]
                        n1152 = To Word Integer(number=w2105) -> (16bit integer=w2104:i16)
                        n1153 = Replace Array Subset(array=w2106, new element=w2099, index (row)=w2104, index (col)=1) -> (w2102:string[][])
                      }
                      frame True {
                        n1154 = local read "New: STS"() -> (w2114:dbl)
                        n1155 = Search 1D Array(1D array=w2111, element="S.T.S. (V/decade):") -> (index of element=w2117:i32)  [unwired: 1 in]
                        n1156 = Divide(x=w2117, y=3) -> (x/y=w2118:dbl)
                        n1157 = To Word Integer(number=w2118) -> (16bit integer=w2109:i16)
                        n1158 = Format Value(format string="%#g", value (0)=w2114) -> (output string=w2121:string)  [unwired: 1 in]
                        n1159 = Build Array(w2110, w2121) -> (w2116:string[])
                        n1160 = Replace Array Subset(array=w2112, new element=w2116, index (row)=w2109) -> (w2113:string[][])  [unwired: 1 in]
                      }
                    }
                    n1161 = local write "Save1 Array"(w2095) -> ()
                  }
                  frame #11 {
                    w2122 = "Trap Density-VT (Traps/Vcm^2):"
                    n1162 = local read "Save1 Array"() -> (w2124:string[][])
                    n1163 = Array Size(array=w2124) -> (size(s)=w2129:i32[])
                    n1164 = Array Subset(array=w2124, index (row)=0, index (col)=0, length (col)=3) -> (w2125:string[][])  [unwired: 1 in]
                    n1165 = Index Array(array=w2129, index=0) -> (element=w2131:i32)
                    n1166 = Reshape Array(w2125, w2131) -> (w2123:string[])
                    n1167 = Search 1D Array(1D array=w2123, element=w2122) -> (index of element=w2134:i32)  [unwired: 1 in]
                    n1168 = Equal?(x=w2134, y=-1) -> (x = y?=w2133:bool)
                    n1169 = case shown="True" w2133 {
                      tunnel: w2124 -> [w2143 w2148]
                      tunnel: w2134 -> [w2139 _]
                      tunnel: [w2138 w2149] -> w2132
                      tunnel: w2123 -> [_ w2147]
                      tunnel: w2122 -> [_ w2146]
                      frame False {
                        n1170 = local read "New: Trap Density-VT"() -> (w2137:dbl)
                        n1171 = Format Value(format string="%#g", value (0)=w2137) -> (output string=w2140:string)  [unwired: 1 in]
                        n1172 = Divide(x=w2139, y=3) -> (x/y=w2142:dbl)
                        n1173 = To Word Integer(number=w2142) -> (16bit integer=w2141:i16)
                        n1174 = Replace Array Subset(array=w2143, new element=w2140, index (row)=w2141, index (col)=1) -> (w2138:string[][])
                      }
                      frame True {
                        n1175 = local read "New: Trap Density-VT"() -> (w2159:dbl)
                        n1176 = Search 1D Array(1D array=w2147, element="STS-Sat (V/decade):") -> (index of element=w2154:i32)  [unwired: 1 in]
                        n1177 = Divide(x=w2154, y=3) -> (x/y=w2153:dbl)
                        n1178 = To Word Integer(number=w2153) -> (16bit integer=w2155:i16)
                        n1179 = Format Value(format string="%#g", value (0)=w2159) -> (output string=w2150:string)  [unwired: 1 in]
                        n1180 = Build Array(w2146, w2150) -> (w2157:string[])
                        n1181 = Increment(x=w2155) -> (x+1=w2156:i16)
                        n1182 = Insert Into Array(array=w2148, index (row)=w2156, new element=w2157) -> (w2149:string[][])  [unwired: 1 in]
                      }
                    }
                    n1183 = local write "Save1 Array"(w2132) -> ()
                  }
                  frame #12 {
                    w2160 = "Trap Density-STS (Traps/Vcm^2):"
                    n1184 = local read "Save1 Array"() -> (w2162:string[][])
                    n1185 = Array Size(array=w2162) -> (size(s)=w2167:i32[])
                    n1186 = Array Subset(array=w2162, index (row)=0, index (col)=0, length (col)=3) -> (w2163:string[][])  [unwired: 1 in]
                    n1187 = Index Array(array=w2167, index=0) -> (element=w2169:i32)
                    n1188 = Reshape Array(w2163, w2169) -> (w2161:string[])
                    n1189 = Search 1D Array(1D array=w2161, element=w2160) -> (index of element=w2172:i32)  [unwired: 1 in]
                    n1190 = Equal?(x=w2172, y=-1) -> (x = y?=w2171:bool)
                    n1191 = case shown="True" w2171 {
                      tunnel: w2162 -> [w2181 w2186]
                      tunnel: w2172 -> [w2178 _]
                      tunnel: [w2177 w2187] -> w2170
                      tunnel: w2161 -> [_ w2185]
                      tunnel: w2160 -> [_ w2184]
                      frame False {
                        n1192 = local read "New: Trap Density-STS"() -> (w2175:dbl)
                        n1193 = Divide(x=w2178, y=3) -> (x/y=w2180:dbl)
                        n1194 = To Word Integer(number=w2180) -> (16bit integer=w2179:i16)
                        n1195 = Format Value(format string="%#g", value (0)=w2175) -> (output string=w2174:string)  [unwired: 1 in]
                        n1196 = Replace Array Subset(array=w2181, new element=w2174, index (row)=w2179, index (col)=1) -> (w2177:string[][])
                      }
                      frame True {
                        n1197 = local read "New: Trap Density-STS"() -> (w2188:dbl)
                        n1198 = Search 1D Array(1D array=w2185, element="Trap Density-VT (Traps/Vcm^2):") -> (index of element=w2193:i32)  [unwired: 1 in]
                        n1199 = Divide(x=w2193, y=3) -> (x/y=w2194:dbl)
                        n1200 = To Word Integer(number=w2194) -> (16bit integer=w2192:i16)
                        n1201 = Format Value(format string="%#g", value (0)=w2188) -> (output string=w2197:string)  [unwired: 1 in]
                        n1202 = Build Array(w2184, w2197) -> (w2190:string[])
                        n1203 = Increment(x=w2192) -> (x+1=w2191:i16)
                        n1204 = Insert Into Array(array=w2186, index (row)=w2191, new element=w2190) -> (w2187:string[][])  [unwired: 1 in]
                      }
                    }
                    n1205 = local write "Save1 Array"(w2170) -> ()
                  }
                }
                n1206 = Concatenate Strings(w1758, "\\", w1756) -> (w1757:string)
                n1207 = String To Path(string=w1757) -> (path=w1747:path)
                n1208 = disable-structure shown="Disabled" {
                  frame Disabled {
                  }
                  frame Enabled {
                  }
                }
              }
              frame #2 {
                n1209 = Equal?(x=w2256, y=w2253) -> (x = y?=w2255:bool)
                n1210 = case shown="False" w2255 {
                  tunnel: w2256 -> [w2259 _]
                  tunnel: w2253 -> [w2258 _]
                  frame False {
                    n1211 = Move(source path=w2259, 9:TRUE, 10:w2258) -> ()  [unwired: 2 in, 3 out]
                  }
                  frame True {
                  }
                }
              }
              frame #3 {
                n1212 = local write "Transfer File"(w2260) -> ()
                n1213 = call-poly <vilib>:"Write To Spreadsheet File.vi"("2D data"=w2261, "file path (dialog if empty)"=w2260) -> ()  [unwired: 6 in, 1 out]
              }
            }
          }
          event "Save Changes? 2": Mouse Down {
            n1214 = event-data() -> ()  [unwired: 1 in, 5 out]
            n1215 = stacked-sequence {
              seq-local: [w2319 _ _ _ _] -> [_ w2779 _ _ _]
              seq-local: [w2318 _ _ _ _] -> [_ w2780 _ _ _]
              seq-local: [w2318 _ _ _ _] -> [_ w2778 _ _ _]
              seq-local: [w2320 _ _ _ _] -> [_ w2776 _ _ _]
              seq-local: [_ w2780 _ _ _] -> [_ _ w2785 _ _]
              seq-local: [_ w2776 _ _ _] -> [_ _ w2784 _ _]
              frame #0 {
                n1216 = local read "Transfer File"() -> (w2319:path)
                n1217 = local read "New: Temp"() -> (w2322:dbl)
                n1218 = local read "New: Length"() -> (w2325:dbl)
                n1219 = local read "New: Width"() -> (w2323:dbl)
                n1220 = To Word Integer(number=w2322) -> (16bit integer=w2321:i16)
                n1221 = Number To Decimal String(number=w2321) -> (decimal integer string=w2329:string)  [unwired: 1 in]
                n1222 = To Single Precision Float(number=w2323) -> (single precision float=w2324:sgl)
                n1223 = To Single Precision Float(number=w2325) -> (single precision float=w2326:sgl)
                n1224 = local read "Index"() -> (w2333:string)
                n1225 = Strip Path(path=w2319) -> (stripped path=w2338:path)  [unwired: 1 out]
                n1226 = Number To Decimal String(number=w2326) -> (decimal integer string=w2331:string)  [unwired: 1 in]
                n1227 = Number To Decimal String(number=w2324) -> (decimal integer string=w2332:string)  [unwired: 1 in]
                n1228 = Concatenate Strings("_", w2329, "K") -> (w2327:string)
                n1229 = call "Build Text2"("Temp"=w2327, "Index"=w2333, "Length"=w2331, "Width"=w2332) -> ("Result"=w2334:string)  [unwired: 10 in, 1 out]
                n1230 = Path To String(path=w2338) -> (string=w2336:string)
                n1231 = Concatenate Strings(w2336, "\\", w2334) -> (w2335:string)
                n1232 = stacked-sequence {
                  tunnel: [_ _ _ _ _ _ _ _ _ _ _ _ w2738] -> _
                  tunnel: w2319 -> [w2340 _ _ _ _ _ _ _ _ _ _ _ _]
                  tunnel: [_ _ _ _ _ _ _ _ _ _ _ _ w2738] -> w2320
                  frame #0 {
                    n1233 = call-poly <vilib>:"Read From Spreadsheet File.vi"("file path (dialog if empty)"=w2340) -> ("all rows"=w2339:string[][])  [unwired: 6 in, 4 out]
                    n1234 = Array Size(array=w2339) -> (size(s)=w2344:i32[])
                    n1235 = Array Subset(array=w2339, index (row)=0, index (col)=0, length (col)=3) -> (w2348:string[][])  [unwired: 1 in]
                    n1236 = Index Array(array=w2344, index=0) -> (element=w2342:i32)
                    n1237 = Reshape Array(w2348, w2342) -> (w2341:string[])
                    n1238 = Search 1D Array(1D array=w2341, element="Dielectric (nm):") -> (index of element=w2351:i32)  [unwired: 1 in]
                    n1239 = Equal?(x=w2351, y=-1) -> (x = y?=w2350:bool)
                    n1240 = case shown="False" w2350 {
                      tunnel: w2339 -> [w2359 w2363]
                      tunnel: w2351 -> [w2355 _]
                      tunnel: [w2354 w2363] -> w2349
                      frame False {
                        n1241 = local read "New: Dielectric"() -> (w2361:dbl)
                        n1242 = Number To Fractional String(number=w2361) -> (F-format string=w2356:string)  [unwired: 3 in]
                        n1243 = Divide(x=w2355, y=3) -> (x/y=w2358:dbl)
                        n1244 = To Word Integer(number=w2358) -> (16bit integer=w2357:i16)
                        n1245 = Replace Array Subset(array=w2359, new element=w2356, index (row)=w2357, index (col)=1) -> (w2354:string[][])
                      }
                      frame True {
                      }
                    }
                    n1246 = local write "Save1 Array"(w2349) -> ()
                  }
                  frame #1 {
                    n1247 = local read "Save1 Array"() -> (w2365:string[][])
                    n1248 = Array Size(array=w2365) -> (size(s)=w2368:i32[])
                    n1249 = Array Subset(array=w2365, index (row)=0, index (col)=0, length (col)=3) -> (w2372:string[][])  [unwired: 1 in]
                    n1250 = Index Array(array=w2368, index=0) -> (element=w2366:i32)
                    n1251 = Reshape Array(w2372, w2366) -> (w2364:string[])
                    n1252 = Search 1D Array(1D array=w2364, element="Length (um):") -> (index of element=w2375:i32)  [unwired: 1 in]
                    n1253 = Equal?(x=w2375, y=-1) -> (x = y?=w2374:bool)
                    n1254 = case shown="False" w2374 {
                      tunnel: w2365 -> [w2385 w2388]
                      tunnel: w2375 -> [w2382 _]
                      tunnel: [w2381 w2388] -> w2373
                      frame False {
                        n1255 = local read "New: Length"() -> (w2378:dbl)
                        n1256 = Divide(x=w2382, y=3) -> (x/y=w2384:dbl)
                        n1257 = Format Value(format string="%#g", value (0)=w2378) -> (output string=w2379:string)  [unwired: 1 in]
                        n1258 = To Word Integer(number=w2384) -> (16bit integer=w2383:i16)
                        n1259 = Replace Array Subset(array=w2385, new element=w2379, index (row)=w2383, index (col)=1) -> (w2381:string[][])
                      }
                      frame True {
                      }
                    }
                    n1260 = local write "Save1 Array"(w2373) -> ()
                  }
                  frame #2 {
                    n1261 = local read "Save1 Array"() -> (w2390:string[][])
                    n1262 = Array Size(array=w2390) -> (size(s)=w2395:i32[])
                    n1263 = Array Subset(array=w2390, index (row)=0, index (col)=0, length (col)=3) -> (w2391:string[][])  [unwired: 1 in]
                    n1264 = Index Array(array=w2395, index=0) -> (element=w2397:i32)
                    n1265 = Reshape Array(w2391, w2397) -> (w2389:string[])
                    n1266 = Search 1D Array(1D array=w2389, element="Width (um):") -> (index of element=w2400:i32)  [unwired: 1 in]
                    n1267 = Equal?(x=w2400, y=-1) -> (x = y?=w2399:bool)
                    n1268 = case shown="False" w2399 {
                      tunnel: w2400 -> [w2408 _]
                      tunnel: w2390 -> [w2407 w2413]
                      tunnel: [w2406 w2413] -> w2398
                      frame False {
                        n1269 = local read "New: Width"() -> (w2403:dbl)
                        n1270 = Divide(x=w2408, y=3) -> (x/y=w2410:dbl)
                        n1271 = To Word Integer(number=w2410) -> (16bit integer=w2409:i16)
                        n1272 = Format Value(format string="%#g", value (0)=w2403) -> (output string=w2404:string)  [unwired: 1 in]
                        n1273 = Replace Array Subset(array=w2407, new element=w2404, index (row)=w2409, index (col)=1) -> (w2406:string[][])
                      }
                      frame True {
                      }
                    }
                    n1274 = local write "Save1 Array"(w2398) -> ()
                  }
                  frame #3 {
                    w2423 = "Sample Temp (K):"
                    n1275 = local read "Save1 Array"() -> (w2415:string[][])
                    n1276 = Array Size(array=w2415) -> (size(s)=w2420:i32[])
                    n1277 = Array Subset(array=w2415, index (row)=0, index (col)=0, length (col)=3) -> (w2416:string[][])  [unwired: 1 in]
                    n1278 = Index Array(array=w2420, index=0) -> (element=w2422:i32)
                    n1279 = Reshape Array(w2416, w2422) -> (w2414:string[])
                    n1280 = Search 1D Array(1D array=w2414, element=w2423) -> (index of element=w2426:i32)  [unwired: 1 in]
                    n1281 = Equal?(x=w2426, y=-1) -> (x = y?=w2425:bool)
                    n1282 = case shown="True" w2425 {
                      tunnel: w2415 -> [w2435 w2449]
                      tunnel: w2426 -> [w2432 _]
                      tunnel: [w2431 w2448] -> w2424
                      tunnel: w2414 -> [_ w2451]
                      tunnel: w2423 -> [_ w2438]
                      frame False {
                        n1283 = local read "New: Temp"() -> (w2429:dbl)
                        n1284 = Divide(x=w2432, y=3) -> (x/y=w2434:dbl)
                        n1285 = Format Value(format string="%#g", value (0)=w2429) -> (output string=w2428:string)  [unwired: 1 in]
                        n1286 = To Word Integer(number=w2434) -> (16bit integer=w2433:i16)
                        n1287 = Replace Array Subset(array=w2435, new element=w2428, index (row)=w2433, index (col)=1) -> (w2431:string[][])
                      }
                      frame True {
                        n1288 = local read "New: Temp"() -> (w2440:dbl)
                        n1289 = Search 1D Array(1D array=w2451, element="Width (um):") -> (index of element=w2445:i32)  [unwired: 1 in]
                        n1290 = Divide(x=w2445, y=3) -> (x/y=w2446:dbl)
                        n1291 = To Word Integer(number=w2446) -> (16bit integer=w2444:i16)
                        n1292 = Format Value(format string="%#g", value (0)=w2440) -> (output string=w2439:string)  [unwired: 1 in]
                        n1293 = Build Array(w2438, w2439) -> (w2442:string[])
                        n1294 = Increment(x=w2444) -> (x+1=w2443:i16)
                        n1295 = Insert Into Array(array=w2449, index (row)=w2443, new element=w2442) -> (w2448:string[][])  [unwired: 1 in]
                      }
                    }
                    n1296 = local write "Save1 Array"(w2424) -> ()
                  }
                  frame #4 {
                    w2461 = "Mobility-Sat (cm^2/Vs):"
                    n1297 = local read "Save1 Array"() -> (w2453:string[][])
                    n1298 = Array Size(array=w2453) -> (size(s)=w2458:i32[])
                    n1299 = Array Subset(array=w2453, index (row)=0, index (col)=0, length (col)=3) -> (w2454:string[][])  [unwired: 1 in]
                    n1300 = Index Array(array=w2458, index=0) -> (element=w2460:i32)
                    n1301 = Reshape Array(w2454, w2460) -> (w2452:string[])
                    n1302 = Search 1D Array(1D array=w2452, element=w2461) -> (index of element=w2464:i32)  [unwired: 1 in]
                    n1303 = Equal?(x=w2464, y=-1) -> (x = y?=w2463:bool)
                    n1304 = case shown="True" w2463 {
                      tunnel: w2453 -> [w2473 w2481]
                      tunnel: w2464 -> [w2470 _]
                      tunnel: [w2469 w2480] -> w2462
                      tunnel: w2452 -> [_ w2478]
                      tunnel: w2461 -> [_ w2476]
                      frame False {
                        n1305 = local read "New: Mobility-Sat"() -> (w2466:dbl)
                        n1306 = Divide(x=w2470, y=3) -> (x/y=w2472:dbl)
                        n1307 = To Word Integer(number=w2472) -> (16bit integer=w2471:i16)
                        n1308 = Format Value(format string="%#g", value (0)=w2466) -> (output string=w2467:string)  [unwired: 1 in]
                        n1309 = Replace Array Subset(array=w2473, new element=w2467, index (row)=w2471, index (col)=1) -> (w2469:string[][])
                      }
                      frame True {
                        n1310 = local read "New: Mobility-Sat"() -> (w2482:dbl)
                        n1311 = Search 1D Array(1D array=w2478, element="Mobility (cm^2/Vs):") -> (index of element=w2485:i32)  [unwired: 1 in]
                        n1312 = Divide(x=w2485, y=3) -> (x/y=w2486:dbl)
                        n1313 = To Word Integer(number=w2486) -> (16bit integer=w2477:i16)
                        n1314 = Format Value(format string="%#g", value (0)=w2482) -> (output string=w2479:string)  [unwired: 1 in]
                        n1315 = Build Array(w2476, w2479) -> (w2484:string[])
                        n1316 = Replace Array Subset(array=w2481, new element=w2484, index (row)=w2477) -> (w2480:string[][])  [unwired: 1 in]
                      }
                    }
                    n1317 = local write "Save1 Array"(w2462) -> ()
                  }
                  frame #5 {
                    w2498 = "Mobility-Lin (cm^2/Vs):"
                    n1318 = local read "Save1 Array"() -> (w2489:string[][])
                    n1319 = Array Size(array=w2489) -> (size(s)=w2495:i32[])
                    n1320 = Array Subset(array=w2489, index (row)=0, index (col)=0, length (col)=3) -> (w2491:string[][])  [unwired: 1 in]
                    n1321 = Index Array(array=w2495, index=0) -> (element=w2497:i32)
                    n1322 = Reshape Array(w2491, w2497) -> (w2490:string[])
                    n1323 = Search 1D Array(1D array=w2490, element=w2498) -> (index of element=w2501:i32)  [unwired: 1 in]
                    n1324 = Equal?(x=w2501, y=-1) -> (x = y?=w2500:bool)
                    n1325 = case shown="True" w2500 {
                      tunnel: w2489 -> [w2510 w2516]
                      tunnel: w2501 -> [w2507 _]
                      tunnel: [w2506 w2515] -> w2499
                      tunnel: w2490 -> [_ w2514]
                      tunnel: w2498 -> [_ w2513]
                      frame False {
                        n1326 = local read "Calc: Mobility-Lin"() -> (w2503:dbl)
                        n1327 = Divide(x=w2507, y=3) -> (x/y=w2509:dbl)
                        n1328 = To Word Integer(number=w2509) -> (16bit integer=w2508:i16)
                        n1329 = Format Value(format string="%#g", value (0)=w2503) -> (output string=w2504:string)  [unwired: 1 in]
                        n1330 = Replace Array Subset(array=w2510, new element=w2504, index (row)=w2508, index (col)=1) -> (w2506:string[][])
                      }
                      frame True {
                        n1331 = local read "Calc: Mobility-Lin"() -> (w2517:dbl)
                        n1332 = Search 1D Array(1D array=w2514, element="Mobility-Sat (cm^2/Vs):") -> (index of element=w2522:i32)  [unwired: 1 in]
                        n1333 = Divide(x=w2522, y=3) -> (x/y=w2523:dbl)
                        n1334 = To Word Integer(number=w2523) -> (16bit integer=w2521:i16)
                        n1335 = Format Value(format string="%#g", value (0)=w2517) -> (output string=w2526:string)  [unwired: 1 in]
                        n1336 = Build Array(w2513, w2526) -> (w2519:string[])
                        n1337 = Increment(x=w2521) -> (x+1=w2520:i16)
                        n1338 = Insert Into Array(array=w2516, index (row)=w2520, new element=w2519) -> (w2515:string[][])  [unwired: 1 in]
                      }
                    }
                    n1339 = local write "Save1 Array"(w2499) -> ()
                  }
                  frame #6 {
                    w2536 = "On/Off I-Sat:"
                    n1340 = local read "Save1 Array"() -> (w2527:string[][])
                    n1341 = Array Size(array=w2527) -> (size(s)=w2533:i32[])
                    n1342 = Array Subset(array=w2527, index (row)=0, index (col)=0, length (col)=3) -> (w2529:string[][])  [unwired: 1 in]
                    n1343 = Index Array(array=w2533, index=0) -> (element=w2535:i32)
                    n1344 = Reshape Array(w2529, w2535) -> (w2528:string[])
                    n1345 = Search 1D Array(1D array=w2528, element=w2536) -> (index of element=w2539:i32)  [unwired: 1 in]
                    n1346 = Equal?(x=w2539, y=-1) -> (x = y?=w2538:bool)
                    n1347 = case shown="True" w2538 {
                      tunnel: w2527 -> [w2548 w2555]
                      tunnel: w2539 -> [w2545 _]
                      tunnel: [w2544 w2556] -> w2537
                      tunnel: w2528 -> [_ w2553]
                      tunnel: w2536 -> [_ w2551]
                      frame False {
                        n1348 = local read "Calc: On/Off"() -> (w2541:dbl)
                        n1349 = Divide(x=w2545, y=3) -> (x/y=w2547:dbl)
                        n1350 = To Word Integer(number=w2547) -> (16bit integer=w2546:i16)
                        n1351 = Format Value(format string="%#g", value (0)=w2541) -> (output string=w2542:string)  [unwired: 1 in]
                        n1352 = Replace Array Subset(array=w2548, new element=w2542, index (row)=w2546, index (col)=1) -> (w2544:string[][])
                      }
                      frame True {
                        n1353 = local read "Calc: On/Off"() -> (w2557:dbl)
                        n1354 = Search 1D Array(1D array=w2553, element="On/Off Current:") -> (index of element=w2560:i32)  [unwired: 1 in]
                        n1355 = Divide(x=w2560, y=3) -> (x/y=w2561:dbl)
                        n1356 = To Word Integer(number=w2561) -> (16bit integer=w2552:i16)
                        n1357 = Format Value(format string="%#g", value (0)=w2557) -> (output string=w2554:string)  [unwired: 1 in]
                        n1358 = Build Array(w2551, w2554) -> (w2559:string[])
                        n1359 = Replace Array Subset(array=w2555, new element=w2559, index (row)=w2552) -> (w2556:string[][])  [unwired: 1 in]
                      }
                    }
                    n1360 = local write "Save1 Array"(w2537) -> ()
                  }
                  frame #7 {
                    w2573 = "Off I-Sat (A):"
                    n1361 = local read "Save1 Array"() -> (w2564:string[][])
                    n1362 = Array Size(array=w2564) -> (size(s)=w2570:i32[])
                    n1363 = Array Subset(array=w2564, index (row)=0, index (col)=0, length (col)=3) -> (w2566:string[][])  [unwired: 1 in]
                    n1364 = Index Array(array=w2570, index=0) -> (element=w2572:i32)
                    n1365 = Reshape Array(w2566, w2572) -> (w2565:string[])
                    n1366 = Search 1D Array(1D array=w2565, element=w2573) -> (index of element=w2576:i32)  [unwired: 1 in]
                    n1367 = Equal?(x=w2576, y=-1) -> (x = y?=w2575:bool)
                    n1368 = case shown="True" w2575 {
                      tunnel: w2564 -> [w2585 w2591]
                      tunnel: w2576 -> [w2582 _]
                      tunnel: [w2581 w2590] -> w2574
                      tunnel: w2565 -> [_ w2589]
                      tunnel: w2573 -> [_ w2588]
                      frame False {
                        n1369 = local read "Calc: Off I-Sat"() -> (w2580:dbl)
                        n1370 = Divide(x=w2582, y=3) -> (x/y=w2584:dbl)
                        n1371 = Format Value(format string="%#g", value (0)=w2580) -> (output string=w2578:string)  [unwired: 1 in]
                        n1372 = To Word Integer(number=w2584) -> (16bit integer=w2583:i16)
                        n1373 = Replace Array Subset(array=w2585, new element=w2578, index (row)=w2583, index (col)=1) -> (w2581:string[][])
                      }
                      frame True {
                        n1374 = local read "Calc: Off I-Sat"() -> (w2592:dbl)
                        n1375 = Search 1D Array(1D array=w2589, element="On/Off I-Sat:") -> (index of element=w2597:i32)  [unwired: 1 in]
                        n1376 = Divide(x=w2597, y=3) -> (x/y=w2598:dbl)
                        n1377 = To Word Integer(number=w2598) -> (16bit integer=w2596:i16)
                        n1378 = Format Value(format string="%#g", value (0)=w2592) -> (output string=w2601:string)  [unwired: 1 in]
                        n1379 = Build Array(w2588, w2601) -> (w2594:string[])
                        n1380 = Increment(x=w2596) -> (x+1=w2595:i16)
                        n1381 = Insert Into Array(array=w2591, index (row)=w2595, new element=w2594) -> (w2590:string[][])  [unwired: 1 in]
                      }
                    }
                    n1382 = local write "Save1 Array"(w2574) -> ()
                  }
                  frame #8 {
                    w2603 = "Vt-Sat (V):"
                    n1383 = local read "Save1 Array"() -> (w2604:string[][])
                    n1384 = Array Size(array=w2604) -> (size(s)=w2609:i32[])
                    n1385 = Array Subset(array=w2604, index (row)=0, index (col)=0, length (col)=3) -> (w2605:string[][])  [unwired: 1 in]
                    n1386 = Index Array(array=w2609, index=0) -> (element=w2611:i32)
                    n1387 = Reshape Array(w2605, w2611) -> (w2602:string[])
                    n1388 = Search 1D Array(1D array=w2602, element=w2603) -> (index of element=w2614:i32)  [unwired: 1 in]
                    n1389 = Equal?(x=w2614, y=-1) -> (x = y?=w2613:bool)
                    n1390 = case shown="True" w2613 {
                      tunnel: w2604 -> [w2621 w2630]
                      tunnel: w2614 -> [w2617 _]
                      tunnel: [w2616 w2629] -> w2612
                      tunnel: w2603 -> [_ w2628]
                      tunnel: w2602 -> [_ w2627]
                      frame False {
                        n1391 = local read "New: VT-Sat"() -> (w2623:dbl)
                        n1392 = Number To Fractional String(number=w2623) -> (F-format string=w2618:string)  [unwired: 3 in]
                        n1393 = Divide(x=w2617, y=3) -> (x/y=w2620:dbl)
                        n1394 = To Word Integer(number=w2620) -> (16bit integer=w2619:i16)
                        n1395 = Replace Array Subset(array=w2621, new element=w2618, index (row)=w2619, index (col)=1) -> (w2616:string[][])
                      }
                      frame True {
                        n1396 = local read "New: VT-Sat"() -> (w2631:dbl)
                        n1397 = Search 1D Array(1D array=w2627, element="Threshold V (V):") -> (index of element=w2626:i32)  [unwired: 1 in]
                        n1398 = Divide(x=w2626, y=3) -> (x/y=w2634:dbl)
                        n1399 = To Word Integer(number=w2634) -> (16bit integer=w2625:i16)
                        n1400 = Format Value(format string="%#g", value (0)=w2631) -> (output string=w2637:string)  [unwired: 1 in]
                        n1401 = Build Array(w2628, w2637) -> (w2633:string[])
                        n1402 = Replace Array Subset(array=w2630, new element=w2633, index (row)=w2625) -> (w2629:string[][])  [unwired: 1 in]
                      }
                    }
                    n1403 = local write "Save1 Array"(w2612) -> ()
                  }
                  frame #9 {
                    n1404 = local read "Save1 Array"() -> (w2638:string[][])
                    n1405 = Array Size(array=w2638) -> (size(s)=w2644:i32[])
                    n1406 = Array Subset(array=w2638, index (row)=0, index (col)=0, length (col)=3) -> (w2640:string[][])  [unwired: 1 in]
                    n1407 = Index Array(array=w2644, index=0) -> (element=w2646:i32)
                    n1408 = Reshape Array(w2640, w2646) -> (w2639:string[])
                    n1409 = Search 1D Array(1D array=w2639, element="VT-Lin (V):") -> (index of element=w2649:i32)  [unwired: 1 in]
                    n1410 = Equal?(x=w2649, y=-1) -> (x = y?=w2648:bool)
                    n1411 = case shown="False" w2648 {
                      tunnel: w2638 -> [w2659 w2662]
                      tunnel: w2649 -> [w2656 _]
                      tunnel: [w2655 w2662] -> w2647
                      frame False {
                        n1412 = local read "New: VT-Lin"() -> (w2653:dbl)
                        n1413 = Divide(x=w2656, y=3) -> (x/y=w2658:dbl)
                        n1414 = Format Value(format string="%#g", value (0)=w2653) -> (output string=w2652:string)  [unwired: 1 in]
                        n1415 = To Word Integer(number=w2658) -> (16bit integer=w2657:i16)
                        n1416 = Replace Array Subset(array=w2659, new element=w2652, index (row)=w2657, index (col)=1) -> (w2655:string[][])
                      }
                      frame True {
                      }
                    }
                    n1417 = local write "Save1 Array"(w2647) -> ()
                  }
                  frame #10 {
                    w2663 = "STS-Sat (V/decade):"
                    n1418 = local read "Save1 Array"() -> (w2665:string[][])
                    n1419 = Array Size(array=w2665) -> (size(s)=w2670:i32[])
                    n1420 = Array Subset(array=w2665, index (row)=0, index (col)=0, length (col)=3) -> (w2666:string[][])  [unwired: 1 in]
                    n1421 = Index Array(array=w2670, index=0) -> (element=w2672:i32)
                    n1422 = Reshape Array(w2666, w2672) -> (w2664:string[])
                    n1423 = Search 1D Array(1D array=w2664, element=w2663) -> (index of element=w2675:i32)  [unwired: 1 in]
                    n1424 = Equal?(x=w2675, y=-1) -> (x = y?=w2674:bool)
                    n1425 = case shown="True" w2674 {
                      tunnel: w2665 -> [w2684 w2690]
                      tunnel: w2675 -> [w2681 _]
                      tunnel: [w2680 w2691] -> w2673
                      tunnel: w2664 -> [_ w2689]
                      tunnel: w2663 -> [_ w2688]
                      frame False {
                        n1426 = local read "New: STS"() -> (w2678:dbl)
                        n1427 = Divide(x=w2681, y=3) -> (x/y=w2683:dbl)
                        n1428 = Format Value(format string="%#g", value (0)=w2678) -> (output string=w2677:string)  [unwired: 1 in]
                        n1429 = To Word Integer(number=w2683) -> (16bit integer=w2682:i16)
                        n1430 = Replace Array Subset(array=w2684, new element=w2677, index (row)=w2682, index (col)=1) -> (w2680:string[][])
                      }
                      frame True {
                        n1431 = local read "New: STS"() -> (w2692:dbl)
                        n1432 = Search 1D Array(1D array=w2689, element="S.T.S. (V/decade):") -> (index of element=w2695:i32)  [unwired: 1 in]
                        n1433 = Divide(x=w2695, y=3) -> (x/y=w2696:dbl)
                        n1434 = To Word Integer(number=w2696) -> (16bit integer=w2687:i16)
                        n1435 = Format Value(format string="%#g", value (0)=w2692) -> (output string=w2699:string)  [unwired: 1 in]
                        n1436 = Build Array(w2688, w2699) -> (w2694:string[])
                        n1437 = Replace Array Subset(array=w2690, new element=w2694, index (row)=w2687) -> (w2691:string[][])  [unwired: 1 in]
                      }
                    }
                    n1438 = local write "Save1 Array"(w2673) -> ()
                  }
                  frame #11 {
                    w2700 = "Trap Density-VT (Traps/Vcm^2):"
                    n1439 = local read "Save1 Array"() -> (w2702:string[][])
                    n1440 = Array Size(array=w2702) -> (size(s)=w2707:i32[])
                    n1441 = Array Subset(array=w2702, index (row)=0, index (col)=0, length (col)=3) -> (w2703:string[][])  [unwired: 1 in]
                    n1442 = Index Array(array=w2707, index=0) -> (element=w2709:i32)
                    n1443 = Reshape Array(w2703, w2709) -> (w2701:string[])
                    n1444 = Search 1D Array(1D array=w2701, element=w2700) -> (index of element=w2712:i32)  [unwired: 1 in]
                    n1445 = Equal?(x=w2712, y=-1) -> (x = y?=w2711:bool)
                    n1446 = case shown="True" w2711 {
                      tunnel: w2702 -> [w2721 w2726]
                      tunnel: w2712 -> [w2717 _]
                      tunnel: [w2716 w2727] -> w2710
                      tunnel: w2701 -> [_ w2725]
                      tunnel: w2700 -> [_ w2724]
                      frame False {
                        n1447 = local read "New: Trap Density-VT"() -> (w2715:dbl)
                        n1448 = Format Value(format string="%#g", value (0)=w2715) -> (output string=w2718:string)  [unwired: 1 in]
                        n1449 = Divide(x=w2717, y=3) -> (x/y=w2720:dbl)
                        n1450 = To Word Integer(number=w2720) -> (16bit integer=w2719:i16)
                        n1451 = Replace Array Subset(array=w2721, new element=w2718, index (row)=w2719, index (col)=1) -> (w2716:string[][])
                      }
                      frame True {
                        n1452 = local read "New: Trap Density-VT"() -> (w2737:dbl)
                        n1453 = Search 1D Array(1D array=w2725, element="STS-Sat (V/decade):") -> (index of element=w2732:i32)  [unwired: 1 in]
                        n1454 = Divide(x=w2732, y=3) -> (x/y=w2731:dbl)
                        n1455 = To Word Integer(number=w2731) -> (16bit integer=w2733:i16)
                        n1456 = Format Value(format string="%#g", value (0)=w2737) -> (output string=w2728:string)  [unwired: 1 in]
                        n1457 = Build Array(w2724, w2728) -> (w2735:string[])
                        n1458 = Increment(x=w2733) -> (x+1=w2734:i16)
                        n1459 = Insert Into Array(array=w2726, index (row)=w2734, new element=w2735) -> (w2727:string[][])  [unwired: 1 in]
                      }
                    }
                    n1460 = local write "Save1 Array"(w2710) -> ()
                  }
                  frame #12 {
                    w2739 = "Trap Density-STS (Traps/Vcm^2):"
                    n1461 = local read "Save1 Array"() -> (w2741:string[][])
                    n1462 = Array Size(array=w2741) -> (size(s)=w2746:i32[])
                    n1463 = Array Subset(array=w2741, index (row)=0, index (col)=0, length (col)=3) -> (w2742:string[][])  [unwired: 1 in]
                    n1464 = Index Array(array=w2746, index=0) -> (element=w2748:i32)
                    n1465 = Reshape Array(w2742, w2748) -> (w2740:string[])
                    n1466 = Search 1D Array(1D array=w2740, element=w2739) -> (index of element=w2750:i32)  [unwired: 1 in]
                    n1467 = Equal?(x=w2750, y=-1) -> (x = y?=w2749:bool)
                    n1468 = case shown="True" w2749 {
                      tunnel: w2741 -> [w2759 w2764]
                      tunnel: w2750 -> [w2756 _]
                      tunnel: [w2755 w2765] -> w2738
                      tunnel: w2740 -> [_ w2763]
                      tunnel: w2739 -> [_ w2762]
                      frame False {
                        n1469 = local read "New: Trap Density-STS"() -> (w2753:dbl)
                        n1470 = Divide(x=w2756, y=3) -> (x/y=w2758:dbl)
                        n1471 = To Word Integer(number=w2758) -> (16bit integer=w2757:i16)
                        n1472 = Format Value(format string="%#g", value (0)=w2753) -> (output string=w2752:string)  [unwired: 1 in]
                        n1473 = Replace Array Subset(array=w2759, new element=w2752, index (row)=w2757, index (col)=1) -> (w2755:string[][])
                      }
                      frame True {
                        n1474 = local read "New: Trap Density-STS"() -> (w2766:dbl)
                        n1475 = Search 1D Array(1D array=w2763, element="Trap Density-VT (Traps/Vcm^2):") -> (index of element=w2771:i32)  [unwired: 1 in]
                        n1476 = Divide(x=w2771, y=3) -> (x/y=w2772:dbl)
                        n1477 = To Word Integer(number=w2772) -> (16bit integer=w2770:i16)
                        n1478 = Format Value(format string="%#g", value (0)=w2766) -> (output string=w2775:string)  [unwired: 1 in]
                        n1479 = Build Array(w2762, w2775) -> (w2768:string[])
                        n1480 = Increment(x=w2770) -> (x+1=w2769:i16)
                        n1481 = Insert Into Array(array=w2764, index (row)=w2769, new element=w2768) -> (w2765:string[][])  [unwired: 1 in]
                      }
                    }
                    n1482 = local write "Save1 Array"(w2738) -> ()
                  }
                }
                n1483 = String To Path(string=w2335) -> (path=w2318:path)
                "No Image 2" <- w2318
              }
              frame #1 {
                n1484 = Equal?(x=w2779, y=w2778) -> (x = y?=w2777:bool)
                n1485 = case shown="False" w2777 {
                  tunnel: w2779 -> [w2783 _]
                  tunnel: w2778 -> [w2782 _]
                  frame False {
                    n1486 = Move(source path=w2783, 9:TRUE, 10:w2782) -> ()  [unwired: 2 in, 3 out]
                  }
                  frame True {
                  }
                }
              }
              frame #2 {
                n1487 = local write "Transfer File"(w2785) -> ()
                n1488 = call-poly <vilib>:"Write To Spreadsheet File.vi"("2D data"=w2784, "file path (dialog if empty)"=w2785) -> ()  [unwired: 6 in, 1 out]
              }
              frame #3 {
                w2885 = 0
                # "Moves to next file and displays new image/data"
                n1489 = property on="Image Out" class="ImageControl"() -> (error out=w2847:errorcluster, "Image Center Position"=w2851:cluster{"X":u32, "Y":u32})  [unwired: 2 in, 1 out]
                n1490 = local read "Transfer File"() -> (w2890:path)
                n1491 = Strip Path(path=w2890) -> (stripped path=w2881:path, name=w2899:string)
                n1492 = Unbundle(w2851) -> ("X"=w2849:u32)  [unwired: 1 out]
                n1493 = local write "Transfer Folder"(w2881) -> ()
                n1494 = Bundle("X"=w2849, 0) -> (w2850:cluster{"X":u32, i32})  [unwired: 1 in]
                n1495 = property on="Image Out" class="ImageControl"(error in=w2847, "Image Center Position"=w2850) -> ()  [unwired: 1 in, 2 out]
                n1496 = List Folder(path=w2881) -> (filenames=w2895:string[])  [unwired: 3 in, 3 out]
                n1497 = Search 1D Array(1D array=w2895, element=w2899) -> (index of element=w2892:i32)  [unwired: 1 in]
                n1498 = Array Size(array=w2895) -> (size(s)=w2891:i32)
                n1499 = Decrement(x=w2891) -> (x-1=w2893:i32)
                n1500 = Equal?(x=w2892, y=w2893) -> (x = y?=w2894:bool)
                n1501 = local read "Folder Index"() -> (w2843:dbl)
                n1502 = case shown="False" w2894 {
                  tunnel: w2843 -> [w3024 _]
                  tunnel: [w3023 0] -> w2842
                  frame False {
                    n1503 = Increment(x=w3024) -> (x+1=w3023:dbl)
                  }
                  frame True {
                  }
                }
                n1504 = invoke on="Image Out" class="ImageControl" method="Clear ROI"() -> ()  [unwired: 3 in, 3 out]
                n1505 = local write "Folder Index"(w2842) -> ()
                n1506 = Path To String(path=w2881) -> (string=w2900:string)
                n1507 = Index Array(array=w2895, index=w2842) -> (element=w2896:string)
                n1508 = local write "Data Name:"(w2896) -> ()
                n1509 = Concatenate Strings(w2900, "\\", w2896) -> (w2898:string)
                n1510 = String To Path(string=w2898) -> (path=w2794:path)
                n1511 = call "Recorded Values.vi"("Path"=w2794) -> ("Recorded Char"=w2796:T5, "Recorded Prop"=w2797:T6, "Fabrication Prop"=w2795:T7)  [unwired: 8 in]
                n1512 = Unbundle By Name(w2796) -> ("Mobility-Sat"=w2809:dbl, "Moblitity-Lin"=w2810:dbl, "On/Off"=w2811:dbl, "Off Current"=w2812:dbl, "Vt-Sat"=w2788:dbl, "STS"=w2813:dbl, "Trap Density-VT"=w2814:dbl, "Trap Density-STS"=w2815:dbl)
                n1513 = Unbundle By Name(w2797) -> ("Date Recorded"=w2805:string, "Index"=w2806:string, "Length"=w2807:dbl, "Width"=w2808:dbl, "Sample Temp"=w2791:dbl)
                n1514 = Unbundle By Name(w2795) -> ("Date Created"=w2816:string, "Material"=w2798:string, "Solvent"=w2799:string, "Concentration"=w2800:dbl, "Method"=w2801:string, "Dielectric (nm)"=w2802:dbl, "Treatment"=w2803:string, "Comments"=w2804:string)
                n1515 = local write "Rec: Off I-Sat"(w2812) -> ()
                n1516 = local write "Rec: VT-Sat"(w2788) -> ()
                n1517 = local write "Date Created"(w2816) -> ()
                n1518 = local write "Rec: Material"(w2798) -> ()
                n1519 = local write "Rec: Solvent"(w2799) -> ()
                n1520 = local write "Rec: Concentration"(w2800) -> ()
                n1521 = local write "Rec: Method"(w2801) -> ()
                n1522 = local write "Rec: Dielectric (d)"(w2802) -> ()
                n1523 = local write "Surface Treatment:"(w2803) -> ()
                n1524 = local write "Comments"(w2804) -> ()
                n1525 = local write "Index"(w2806) -> ()
                n1526 = local write "Rec: Mobility-Sat"(w2809) -> ()
                n1527 = local write "Rec: Mobility-Lin"(w2810) -> ()
                n1528 = local write "Rec: On/Off"(w2811) -> ()
                n1529 = local write "Rec: STS"(w2813) -> ()
                n1530 = local write "Rec: Trap Density-VT"(w2814) -> ()
                n1531 = local write "Rec: Trap Density-STS"(w2815) -> ()
                n1532 = local write "Date Recorded"(w2805) -> ()
                n1533 = local write "Rec: Length"(w2807) -> ()
                n1534 = local write "Rec: Width"(w2808) -> ()
                n1535 = local write "Rec: Temp"(w2791) -> ()
                n1536 = Equal To 0?(x=w2791) -> (x = 0?=w2792:bool)
                n1537 = case shown="False" w2792 {
                  tunnel: [w2901 w2902] -> w2789
                  tunnel: w2791 -> [w2901 _]
                  frame False {
                  }
                  frame True {
                    n1538 = local read "Room Temp"() -> (w2902:dbl)
                  }
                }
                n1539 = local write "Transfer File"(w2794) -> ()
                n1540 = local read "NumPts 2"() -> (w2838:dbl)
                n1541 = local read "NumPts"() -> (w2827:dbl)
                n1542 = local read "NumPts"() -> (w2839:dbl)
                n1543 = call-poly <vilib>:"Read From Spreadsheet File.vi"("file path (dialog if empty)"=w2794) -> ("all rows"=w2887:string[][])  [unwired: 6 in, 4 out]
                n1544 = call "Mobility-Vt Calculator-File.vi"("NumPts"=w2839, "Path"=w2794) -> ("XY Graph-Sat"=w2840:cluster{dbl[], dbl[]}[], "XY Graph-Lin"=w2822:cluster{dbl[], dbl[]}[], "Output"=w2841:T8, "Index-Sat"=w2819:dbl, "Index-Lin"=w2826:dbl)  [unwired: 4 in, 1 out]
                n1545 = Decimate 1D Array(w2822) -> (w2834:cluster{dbl[], dbl[]}[])  [unwired: 1 out]
                n1546 = Array To Cluster(array=w2834) -> (cluster=w2832:T9)
                n1547 = Unbundle(w2832) -> ("[0]"=w2833:cluster{dbl[], dbl[]})  [unwired: 8 out]
                n1548 = local write "XY Graph-Lin"(w2822) -> ()
                n1549 = Unbundle(w2833) -> (w2831:dbl[], w2830:dbl[])
                n1550 = Array Subset(array=w2830, index=w2826, length=w2827) -> (w2828:dbl[])
                n1551 = Array Subset(array=w2831, index=w2826, length=w2827) -> (w2829:dbl[])
                n1552 = call "STS Calculator-File.vi"("NumPts"=w2838, "Path"=w2794) -> ("STS Index-Sat"=w2837:dbl, "XY Graph-Sat"=w2836:cluster{dbl[], dbl[]}[], "Ouput"=w2835:cluster{"STS-Sat":dbl, "STS-Lin":dbl})  [unwired: 5 in, 2 out]
                n1553 = local read "New: Dielectric"() -> (w2821:dbl)
                n1554 = local write "Lin Id-Used"(w2828) -> ()
                n1555 = local write "Lin-Vg Array-Used"(w2829) -> ()
                n1556 = local write "MobVi Index"(w2819) -> ()
                n1557 = local write "Slide"(w2819) -> ()
                n1558 = local write "XY Graph"(w2840) -> ()
                n1559 = local write "Index 2"(w2837) -> ()
                n1560 = local write "XY Graph 2"(w2836) -> ()
                n1561 = Unbundle By Name(w2841) -> ("Mobility-Sat"=w2825:dbl, "Vt-Sat"=w2786:dbl, "Mobility-Lin"=w2824:dbl, "Mobility-Lin"=w2823:dbl, "Off I-Sat"=w2817:dbl, "On/Off I-Sat"=w2787:dbl)
                n1562 = Array Size(array=w2887) -> (size(s)=w2886:i32[])
                n1563 = local write "New: Temp"(w2789) -> ()
                n1564 = Unbundle By Name(w2835) -> ("STS-Sat"=w2820:dbl)
                n1565 = call "Trap Density_STS.vi"("Temp (T) [K]"=w2789, "S.T.S. (S)"=w2820, "Dielectric"=w2821) -> ("Trap Density (N)"=w2793:dbl)  [unwired: 8 in]
                n1566 = local write "Calc: Mobility-Lin"(w2824) -> ()
                n1567 = local write "Calc: Mobility-Sat"(w2825) -> ()
                n1568 = local write "Calc: Off I-Sat"(w2817) -> ()
                n1569 = local write "Calc: VT-Sat"(w2786) -> ()
                n1570 = local write "New: VT-Lin"(w2823) -> ()
                n1571 = local write "New: Trap Density-STS"(w2793) -> ()
                n1572 = local write "Calc: Trap Density-STS"(w2793) -> ()
                n1573 = local read "Image Folder"() -> (w2875:path)
                n1574 = local read "New: Dielectric"() -> (w2818:dbl)
                n1575 = Decimate 1D Array(w2840) -> (w2870:cluster{dbl[], dbl[]}[])  [unwired: 1 out]
                n1576 = Decimate 1D Array(w2836) -> (w2860:cluster{dbl[], dbl[]}[])  [unwired: 1 out]
                n1577 = Index Array(array=w2886, index=w2885) -> (element=w2866:i32)
                n1578 = Array Subset(array=w2887, index (row)=w2885, index (col)=w2885, length (col)=3) -> (w2888:string[][])  [unwired: 1 in]
                n1579 = local write "Calc: STS"(w2820) -> ()
                n1580 = local write "New: VT-Sat"(w2786) -> ()
                n1581 = local write "New: Mobility-Sat"(w2825) -> ()
                n1582 = local write "Calc: On/Off"(w2787) -> ()
                n1583 = local write "New: Mobility-Lin"(w2824) -> ()
                n1584 = List Folder(path=w2875) -> (filenames=w2880:string[])  [unwired: 3 in, 3 out]
                n1585 = local write "New: VT-Lin"(w2823) -> ()
                n1586 = Array To Cluster(array=w2870) -> (cluster=w2872:T9)
                n1587 = Array To Cluster(array=w2860) -> (cluster=w2858:T9)
                n1588 = Reshape Array(w2888, w2866) -> (w2873:string[])
                n1589 = Subtract(x=w2866, y=20) -> (x-y=w2865:i32)
                n1590 = local write "New: STS"(w2820) -> ()
                n1591 = property on="Slide" class="Slide (strict)"("Scale.Maximum"=w2865) -> ()  [unwired: 2 in, 2 out]
                n1592 = call "Trap Density_VT.vi"("VT"=w2786, "Dielectric"=w2818) -> ("Trap Density-VT"=w2790:dbl)
                n1593 = Unbundle(w2872) -> ("[0]"=w2871:cluster{dbl[], dbl[]})  [unwired: 8 out]
                n1594 = Unbundle(w2858) -> ("[0]"=w2859:cluster{dbl[], dbl[]})  [unwired: 8 out]
                n1595 = Search 1D Array(1D array=w2873, element="Index:") -> (index of element=w2882:i32)  [unwired: 1 in]
                n1596 = local write "New: Trap Density-VT"(w2790) -> ()
                n1597 = local write "Calc: Trap Density-VT"(w2790) -> ()
                n1598 = Unbundle(w2871) -> (w2862:dbl[], w2861:dbl[])
                n1599 = Unbundle(w2859) -> (w2857:dbl[], w2856:dbl[])
                n1600 = Increment(x=w2882) -> (x+1=w2883:i32)
                n1601 = Array Subset(array=w2862, index=w2819, length=w2839) -> (w2869:dbl[])
                n1602 = Array Subset(array=w2861, index=w2819, length=w2839) -> (w2868:dbl[])
                n1603 = Array Subset(array=w2857, index=w2837, length=w2838) -> (w2864:dbl[])
                n1604 = Array Subset(array=w2856, index=w2837, length=w2838) -> (w2863:dbl[])
                n1605 = Index Array(array=w2873, index=w2883) -> (element=w2878:string)
                n1606 = local write "Vg Array-Log-Used"(w2863) -> ()
                n1607 = local write "Sat Id-Log-Used"(w2864) -> ()
                n1608 = local write "Sat Id-Used"(w2868) -> ()
                n1609 = local write "Index"(w2878) -> ()
                n1610 = local write "Sat Vg Array-Used"(w2869) -> ()
                n1611 = while {
                  tunnel: w2880 -> [w2910]
                  tunnel: w2878 -> [w2908]
                  tunnel: [w2907] -> _
                  tunnel: [w2907] -> w2879
                  tunnel: w2866 -> [w2906]
                  i -> [w2907]
                  stop <- w2903 stop-if-true
                  n1612 = Index Array(array=w2910, index=w2907) -> (element=w2911:string)
                  n1613 = xnode "Match Regular Expression"("input string"=w2911, "regular expression"=w2908) -> ("whole match"=w2909:string)  [unwired: 4 in, 4 out]
                  n1614 = Equal?(x=w2909, y=w2908) -> (x = y?=w2905:bool)
                  n1615 = Equal?(x=w2906, y=w2907) -> (x = y?=w2904:bool)
                  n1616 = Or(x=w2905, y=w2904) -> (x .or. y?=w2903:bool)
                }
                n1617 = Path To String(path=w2875) -> (string=w2877:string)
                n1618 = Index Array(array=w2880, index=w2879) -> (element=w2854:string)
                n1619 = local write "Image Name"(w2854) -> ()
                n1620 = Empty String/Path?(string/path=w2854) -> (empty?=w2855:bool)
                n1621 = Concatenate Strings(w2877, "\\", w2854) -> (w2876:string)
                n1622 = String To Path(string=w2876) -> (path=w2853:path)
                n1623 = local read "No Image File"() -> (w2852:path)
                n1624 = Select(t=w2852, s=w2855, f=w2853) -> (s? t:f=w2846:path)
                n1625 = local write "Image File"(w2846) -> ()
                n1626 = local read "Image Out"() -> (w2844:T2)
                n1627 = call "IMAQ ReadFile"("File Path"=w2846, "Image"=w2844) -> ("Image Out"=w2845:T2)  [unwired: 5 in, 4 out]
                n1628 = local write "Image Out"(w2845) -> ()
                n1629 = local write "Image Out 2"(w2845) -> ()
              }
              frame #4 {
                # "Output ROI data"
                n1630 = local read "Image Folder"() -> (w3026:path)
                n1631 = Build Path(base path=w3026, name or relative path="ROI") -> (appended path=w3028:path)
                n1632 = local read "Index"() -> (w3027:string)
                n1633 = Build Path(base path=w3028, name or relative path=w3027) -> (appended path=w3033:path)
                n1634 = invoke on="Image Out" class="ImageControl" method="Clear ROI"() -> (error out=w3032:errorcluster)  [unwired: 3 in, 2 out]
                n1635 = call <vilib>:"Check if File or Folder Exists.vi"("error in (no error)"=w3032, "path"=w3033) -> ("file or folder exists?"=w3030:bool, "dup path"=w3031:path)  [unwired: 7 in, 1 out]
                n1636 = case shown="True" w3030 {
                  tunnel: w3031 -> [_ w3034]
                  frame False {
                  }
                  frame True {
                    n1637 = Read from Text File(file (use dialog)=w3034) -> (text=w3038:string)  [unwired: 3 in, 3 out]
                    n1638 = property on="Image Out" class="ImageControl"() -> ("ROI"=w3035:T10)  [unwired: 2 in, 2 out]
                    n1639 = Unflatten From String(type=w3035, binary string=w3038) -> (value=w3036:T10, error out=w3037:errorcluster)  [unwired: 3 in, 1 out]
                    n1640 = property on="Image Out" class="ImageControl"(error in=w3037, "ROI"=w3036) -> ()  [unwired: 1 in, 2 out]
                  }
                }
              }
            }
            n1641 = flat-sequence {
              tunnel: [w2275] -> w2262
              tunnel: w2262 -> [w2289]
              frame #0 {
                # "Makes Empty File for Transformer Data"
                n1642 = local read "Transfer Folder"() -> (w2264:path)
                n1643 = Build Path(base path=w2264, name or relative path="Stats") -> (appended path=w2266:path)
                n1644 = call <vilib>:"Check if File or Folder Exists.vi"("path"=w2266) -> ("file or folder exists?"=w2267:bool, "dup path"=w2268:path)  [unwired: 8 in, 1 out]
                n1645 = case shown="False" w2267 {
                  tunnel: [w2272 w2274] -> w2269
                  tunnel: w2268 -> [w2273 w2274]
                  frame False {
                    n1646 = Create Folder(path (use dialog)=w2273) -> (created path=w2272:path)  [unwired: 2 in, 2 out]
                  }
                  frame True {
                  }
                }
                n1647 = Build Path(base path=w2269, name or relative path="Tranformer Data.txt") -> (appended path=w2271:path)
                n1648 = call-poly <vilib>:"Write To Spreadsheet File.vi"("append to file? (new file:F)"=TRUE, "file path (dialog if empty)"=w2271) -> ()  [unwired: 6 in, 1 out]
              }
              frame #1 {
                # "Adds Headers if they don't exist"
                n1649 = local read "Transfer Folder"() -> (w2281:path)
                n1650 = Concatenate Strings("Stats\\", "Tranformer Data.txt") -> (w2282:string)
                n1651 = Build Path(base path=w2281, name or relative path=w2282) -> (appended path=w2275:path)
                n1652 = call-poly <vilib>:"Read From Spreadsheet File.vi"("file path (dialog if empty)"=w2275) -> ("first row"=w2280:string[])  [unwired: 6 in, 4 out]
                n1653 = Search 1D Array(1D array=w2280, element="DeviceID") -> (index of element=w2278:i32)  [unwired: 1 in]
                n1654 = Equal?(x=w2278, y=0) -> (x = y?=w2276:bool)
                n1655 = case shown="False" w2276 {
                  tunnel: w2275 -> [w2286 _]
                  frame False {
                    n1656 = local read "Transformer \nHeaders"() -> (w2285:string[])
                    n1657 = call-poly <vilib>:"Write To Spreadsheet File.vi"("1D data"=w2285, "file path (dialog if empty)"=w2286) -> ()  [unwired: 6 in, 1 out]
                  }
                  frame True {
                  }
                }
              }
              frame #2 {
                # "Adds current device if it doesn't exist"
                n1658 = local read "Current \nRecord"() -> (w2292:string[])
                n1659 = Index Array(array=w2292, index=0) -> (element=w2291:string)
                n1660 = local read "Transfer Folder"() -> (w2294:path)
                n1661 = Concatenate Strings("Stats\\", "Tranformer Data.txt") -> (w2295:string)
                n1662 = local write "Current Device ID"(w2291) -> ()
                n1663 = local read "Current Device ID"() -> (w2301:string)
                n1664 = Build Path(base path=w2294, name or relative path=w2295) -> (appended path=w2293:path)
                n1665 = call-poly <vilib>:"Read From Spreadsheet File.vi"("file path (dialog if empty)"=w2293) -> ("all rows"=w2288:string[][])  [unwired: 6 in, 4 out]
                n1666 = Index Array(array=w2288, index (col)=0) -> (element=w2299:string[])  [unwired: 1 in]
                n1667 = Search 1D Array(1D array=w2299, element=w2301) -> (index of element=w2287:i32)  [unwired: 1 in]
                n1668 = Equal?(x=w2287, y=-1) -> (x = y?=w2290:bool)
                n1669 = case shown="False" w2290 {
                  tunnel: w2289 -> [w2303 w2316]
                  tunnel: w2287 -> [w2308 _]
                  tunnel: w2288 -> [w2309 _]
                  frame False {
                    n1670 = local read "Current \nRecord"() -> (w2307:string[])
                    n1671 = Replace Array Subset(array=w2309, new element=w2307, index (row)=w2308) -> (w2304:string[][])  [unwired: 1 in]
                    n1672 = flat-sequence {
                      tunnel: [w2310] -> _
                      tunnel: [w2311] -> _
                      tunnel: [w2311] -> w2306
                      tunnel: [w2310] -> w2305
                      tunnel: w2304 -> [w2311]
                      tunnel: w2303 -> [w2310]
                      tunnel: w2306 -> [w2313]
                      tunnel: w2305 -> [w2312]
                      frame #0 {
                        n1673 = Delete(path (use dialog)=w2310) -> ()  [unwired: 4 in, 3 out]
                      }
                      frame #1 {
                        n1674 = call-poly <vilib>:"Write To Spreadsheet File.vi"("append to file? (new file:F)"=TRUE, "2D data"=w2313, "file path (dialog if empty)"=w2312) -> ()  [unwired: 5 in, 1 out]
                      }
                    }
                  }
                  frame True {
                    n1675 = local read "Current \nRecord"() -> (w2315:string[])
                    n1676 = call-poly <vilib>:"Write To Spreadsheet File.vi"("append to file? (new file:F)"=TRUE, "1D data"=w2315, "file path (dialog if empty)"=w2316) -> ()  [unwired: 5 in, 1 out]
                  }
                }
              }
            }
          }
          event "Export": Mouse Down {
            n1677 = event-data() -> ()  [unwired: 1 in, 7 out]
            n1678 = flat-sequence {
              frame #0 {
                n1679 = stacked-sequence {
                  frame #0 {
                    n1680 = local read "Independant Variable"() -> (w3040:string)
                    n1681 = Equal?(x=w3040, y="Length (um):") -> (x = y?=w3041:bool)
                    n1682 = case shown="True" w3041 {
                      frame False {
                      }
                      frame True {
                        n1683 = local write "X Axis Display Type"("1") -> ()
                        n1684 = local write "Opj X Axis"("2") -> ()
                      }
                    }
                  }
                  frame #1 {
                    n1685 = local read "Independant Variable"() -> (w3045:string)
                    n1686 = Equal?(x=w3045, y="Sample Temp (K):") -> (x = y?=w3046:bool)
                    n1687 = case shown="True" w3046 {
                      frame False {
                      }
                      frame True {
                        n1688 = local write "X Axis Display Type"("1") -> ()
                        n1689 = local write "Opj X Axis"("1") -> ()
                      }
                    }
                  }
                  frame #2 {
                    n1690 = local read "Independant Variable"() -> (w3050:string)
                    n1691 = Equal?(x=w3050, y="Mobility-Sat (cm^2/Vs):") -> (x = y?=w3051:bool)
                    n1692 = case shown="True" w3051 {
                      frame False {
                      }
                      frame True {
                        n1693 = local write "X Axis Display Type"("2") -> ()
                        n1694 = local write "Opj X Axis"("2") -> ()
                      }
                    }
                  }
                  frame #3 {
                    n1695 = local read "Independant Variable"() -> (w3055:string)
                    n1696 = Equal?(x=w3055, y="Mobility-Lin (cm^2/Vs):") -> (x = y?=w3056:bool)
                    n1697 = case shown="True" w3056 {
                      frame False {
                      }
                      frame True {
                        n1698 = local write "X Axis Display Type"("2") -> ()
                        n1699 = local write "Opj X Axis"("2") -> ()
                      }
                    }
                  }
                  frame #4 {
                    n1700 = local read "Independant Variable"() -> (w3060:string)
                    n1701 = Equal?(x=w3060, y="On/Off I-Sat:") -> (x = y?=w3061:bool)
                    n1702 = case shown="True" w3061 {
                      frame False {
                      }
                      frame True {
                        n1703 = local write "X Axis Display Type"("2") -> ()
                        n1704 = local write "Opj X Axis"("2") -> ()
                      }
                    }
                  }
                  frame #5 {
                    n1705 = local read "Independant Variable"() -> (w3065:string)
                    n1706 = Equal?(x=w3065, y="Off I-Sat (A):") -> (x = y?=w3066:bool)
                    n1707 = case shown="True" w3066 {
                      frame False {
                      }
                      frame True {
                        n1708 = local write "X Axis Display Type"("2") -> ()
                        n1709 = local write "Opj X Axis"("2") -> ()
                      }
                    }
                  }
                  frame #6 {
                    n1710 = local read "Independant Variable"() -> (w3070:string)
                    n1711 = Equal?(x=w3070, y="Vt-Sat (V):") -> (x = y?=w3071:bool)
                    n1712 = case shown="True" w3071 {
                      frame False {
                      }
                      frame True {
                        n1713 = local write "X Axis Display Type"("1") -> ()
                        n1714 = local write "Opj X Axis"("1") -> ()
                      }
                    }
                  }
                  frame #7 {
                    n1715 = local read "Independant Variable"() -> (w3075:string)
                    n1716 = Equal?(x=w3075, y="STS-Sat (V/decade):") -> (x = y?=w3076:bool)
                    n1717 = case shown="True" w3076 {
                      frame False {
                      }
                      frame True {
                        n1718 = local write "X Axis Display Type"("1") -> ()
                        n1719 = local write "Opj X Axis"("1") -> ()
                      }
                    }
                  }
                  frame #8 {
                    n1720 = local read "Independant Variable"() -> (w3080:string)
                    n1721 = Equal?(x=w3080, y="Trap Density-VT (Traps/Vcm^2):") -> (x = y?=w3081:bool)
                    n1722 = case shown="True" w3081 {
                      frame False {
                      }
                      frame True {
                        n1723 = local write "X Axis Display Type"("2") -> ()
                        n1724 = local write "Opj X Axis"("2") -> ()
                      }
                    }
                  }
                  frame #9 {
                    n1725 = local read "Independant Variable"() -> (w3085:string)
                    n1726 = Equal?(x=w3085, y="Trap Density-STS (Traps/Vcm^2):") -> (x = y?=w3086:bool)
                    n1727 = case shown="True" w3086 {
                      frame False {
                      }
                      frame True {
                        n1728 = local write "X Axis Display Type"("2") -> ()
                        n1729 = local write "Opj X Axis"("2") -> ()
                      }
                    }
                  }
                }
              }
              frame #1 {
                n1730 = local read "Transfer Folder"() -> (w3094:path)
                n1731 = Build Path(base path=w3094, name or relative path="Stats") -> (appended path=w3095:path)
                n1732 = local read "Origin Project File"() -> (w3106:path)
                n1733 = call <vilib>:"Check if File or Folder Exists.vi"("path"=w3095) -> ("file or folder exists?"=w3110:bool, "dup path"=w3109:path)  [unwired: 8 in, 1 out]
                n1734 = call <userlib>:"OA_ConnectToOrigin.vi"() -> ("error out"=w3107:errorcluster, "Origin.IOApplication"=w3108:refnum<k7>)  [unwired: 8 in]
                n1735 = case shown="False" w3110 {
                  tunnel: w3109 -> [w3283 w3284]
                  tunnel: [w3282 w3284] -> w3093
                  frame False {
                    n1736 = Create Folder(path (use dialog)=w3283) -> (created path=w3282:path)  [unwired: 2 in, 2 out]
                  }
                  frame True {
                  }
                }
                n1737 = call <userlib>:"OA_Load.vi"("error in (no error)"=w3107, "Path"=w3106, "Origin.IOApplication"=w3108) -> ("error out"=w3104:errorcluster, "Origin.IOApplication"=w3105:refnum<k7>)  [unwired: 1 out]
                n1738 = call <userlib>:"OAExecute.vi"("script"="document -m 3;", "Error IO"=w3104, "Origin.IOApplication"=w3105) -> ("Error IO Out"=w3102:errorcluster, "Origin.IOApplication"=w3103:refnum<k7>)  [unwired: 1 in, 1 out]
                n1739 = call "File Dialog"("start path"=w3095) -> ("selected path"=w3097:path)  [unwired: 11 in, 3 out]
                n1740 = local read "Independant Variable"() -> (w3090:string)
                n1741 = stacked-sequence {
                  tunnel: w3094 -> [w3121 w3151 w3163 w3185 w3205 w3226 w3247 w3270]
                  tunnel: w3093 -> [w3122 w3150 w3164 w3184 w3206 w3227 w3248 w3271]
                  tunnel: w3103 -> [w3124 w3148 w3166 w3187 w3208 w3229 w3250 w3273]
                  tunnel: w3102 -> [w3123 w3149 w3165 w3186 w3207 w3228 w3249 w3272]
                  tunnel: [_ _ _ _ _ _ _ w3268] -> w3092
                  tunnel: [_ _ _ _ _ _ _ w3269] -> w3091
                  tunnel: w3090 -> [w3120 w3141 w3162 w3183 w3204 w3225 w3246 w3267]
                  frame #0 {
                    n1742 = local read "X Axis Display Type"() -> (w3112:string)
                    n1743 = local read "Opj X Axis"() -> (w3117:string)
                    n1744 = Concatenate Strings("window -a MOBLGraph;\nlayer.x.type=", w3117, "; layer.x.label.numFormat = ", w3112, "; Y3 = 1; X3 = 1;", "window -a MOBLTable;\nwindow -s TV;") -> (w3115:string)
                    n1745 = call "Param_Analysis_7_24b_JW.vi"("Independant Variable"=w3120, "error in (no error)"=w3123, "Data Folder"=w3121, "Parameter String"="Mobility-Lin (cm^2/Vs):", "Parameter Name"="Mobility-Lin", "Stats Folder"=w3122) -> ("error out"=w3126:errorcluster, "Output Array"=w3128:string[][], "Variables"=w3119:T16)  [unwired: 2 in, 1 out]
                    n1746 = call "Origin_Export_7_27a_JW.vi"("Input Conditions"=w3119, "Analysis Array"=w3128, "error in (no error)"=w3126, "Parameter Worksheet Name"="[MOBLTable]Mobilities", "Parameter Folder Script"="pe_cd \"Mobility-Lin\";", "Origin.IOApplication"=w3124) -> ("error out"=w3125:errorcluster, "reference out"=w3127:refnum<k7>)  [unwired: 3 in, 1 out]
                    n1747 = call <userlib>:"OAExecute.vi"("script"=w3115, "Error IO"=w3125, "Origin.IOApplication"=w3127) -> ()  [unwired: 1 in, 3 out]
                  }
                  frame #1 {
                    n1748 = local read "X Axis Display Type"() -> (w3133:string)
                    n1749 = local read "Opj X Axis"() -> (w3138:string)
                    n1750 = Concatenate Strings("window -a MOBSGraph;\nlayer.x.type=", w3138, "; layer.x.label.numFormat = ", w3133, "; Y3 = 1; X3 = 1;", "window -a MOBSTable;\nwindow -s TV;") -> (w3136:string)
                    n1751 = call "Param_Analysis_7_24b_JW.vi"("Independant Variable"=w3141, "error in (no error)"=w3149, "Data Folder"=w3151, "Parameter String"="Mobility-Sat (cm^2/Vs):", "Parameter Name"="Mobility-Sat", "Stats Folder"=w3150) -> ("error out"=w3144:errorcluster, "Output Array"=w3142:string[][], "Variables"=w3140:T16)  [unwired: 2 in, 1 out]
                    n1752 = call "Origin_Export_7_27a_JW.vi"("Input Conditions"=w3140, "Analysis Array"=w3142, "error in (no error)"=w3144, "Parameter Worksheet Name"="[MOBSTable]Mobilities", "Parameter Folder Script"="pe_cd \"Mobility-Sat\";", "Origin.IOApplication"=w3148) -> ("error out"=w3143:errorcluster, "reference out"=w3145:refnum<k7>)  [unwired: 3 in, 1 out]
                    n1753 = call <userlib>:"OAExecute.vi"("script"=w3136, "Error IO"=w3143, "Origin.IOApplication"=w3145) -> ()  [unwired: 1 in, 3 out]
                  }
                  frame #2 {
                    n1754 = local read "X Axis Display Type"() -> (w3154:string)
                    n1755 = local read "Opj X Axis"() -> (w3159:string)
                    n1756 = Concatenate Strings("window -a NSTSGraph;\nlayer.x.type=", w3159, "; layer.x.label.numFormat = ", w3154, "; Y3 = 1; X3 = 1;", "window -a NSTSTable;\nwindow -s TV;") -> (w3157:string)
                    n1757 = call "Param_Analysis_7_24b_JW.vi"("Independant Variable"=w3162, "error in (no error)"=w3165, "Data Folder"=w3163, "Parameter String"="Trap Density-STS (Traps/Vcm^2):", "Parameter Name"="Trap Density-STS", "Stats Folder"=w3164) -> ("error out"=w3169:errorcluster, "Output Array"=w3167:string[][], "Variables"=w3161:T16)  [unwired: 2 in, 1 out]
                    n1758 = call "Origin_Export_7_27a_JW.vi"("Input Conditions"=w3161, "Analysis Array"=w3167, "error in (no error)"=w3169, "Parameter Worksheet Name"="[NSTSTable]Trap Densities", "Parameter Folder Script"="pe_cd \"N-STS\";", "Origin.IOApplication"=w3166) -> ("error out"=w3168:errorcluster, "reference out"=w3170:refnum<k7>)  [unwired: 3 in, 1 out]
                    n1759 = call <userlib>:"OAExecute.vi"("script"=w3157, "Error IO"=w3168, "Origin.IOApplication"=w3170) -> ()  [unwired: 1 in, 3 out]
                  }
                  frame #3 {
                    n1760 = local read "X Axis Display Type"() -> (w3175:string)
                    n1761 = local read "Opj X Axis"() -> (w3180:string)
                    n1762 = call "Param_Analysis_7_24b_JW.vi"("Independant Variable"=w3183, "error in (no error)"=w3186, "Data Folder"=w3185, "Parameter String"="Trap Density-VT (Traps/Vcm^2):", "Parameter Name"="Trap Density-Vt", "Stats Folder"=w3184) -> ("error out"=w3190:errorcluster, "Output Array"=w3188:string[][], "Variables"=w3182:T16)  [unwired: 2 in, 1 out]
                    n1763 = Concatenate Strings("window -a NVtGraph;\nlayer.x.type=", w3180, "; layer.x.label.numFormat = ", w3175, "; Y3 = 1; X3 = 1;", "window -a NVtTable;\nwindow -s TV;") -> (w3178:string)
                    n1764 = call "Origin_Export_7_27a_JW.vi"("Input Conditions"=w3182, "Analysis Array"=w3188, "error in (no error)"=w3190, "Parameter Worksheet Name"="[NVTTable]Trap Densities", "Parameter Folder Script"="pe_cd \"N-Vt\";", "Origin.IOApplication"=w3187) -> ("error out"=w3189:errorcluster, "reference out"=w3191:refnum<k7>)  [unwired: 3 in, 1 out]
                    n1765 = call <userlib>:"OAExecute.vi"("script"=w3178, "Error IO"=w3189, "Origin.IOApplication"=w3191) -> ()  [unwired: 1 in, 3 out]
                  }
                  frame #4 {
                    n1766 = local read "X Axis Display Type"() -> (w3196:string)
                    n1767 = local read "Opj X Axis"() -> (w3201:string)
                    n1768 = Concatenate Strings("window -a OffIGraph;\nlayer.x.type=", w3201, "; layer.x.label.numFormat = ", w3196, "; Y3 = 1; X3 = 1;", "window -a OffITable;\nwindow -s TV;") -> (w3199:string)
                    n1769 = call "Param_Analysis_7_24b_JW.vi"("Independant Variable"=w3204, "error in (no error)"=w3207, "Data Folder"=w3205, "Parameter String"="Off I-Sat (A):", "Parameter Name"="Off I-Sat", "Stats Folder"=w3206) -> ("error out"=w3211:errorcluster, "Output Array"=w3209:string[][], "Variables"=w3203:T16)  [unwired: 2 in, 1 out]
                    n1770 = call "Origin_Export_7_27a_JW.vi"("Input Conditions"=w3203, "Analysis Array"=w3209, "error in (no error)"=w3211, "Parameter Worksheet Name"="[OffItable]OffCurrents", "Parameter Folder Script"="pe_cd \"OffI-Sat\";", "Origin.IOApplication"=w3208) -> ("error out"=w3210:errorcluster, "reference out"=w3212:refnum<k7>)  [unwired: 3 in, 1 out]
                    n1771 = call <userlib>:"OAExecute.vi"("script"=w3199, "Error IO"=w3210, "Origin.IOApplication"=w3212) -> ()  [unwired: 1 in, 3 out]
                  }
                  frame #5 {
                    n1772 = local read "X Axis Display Type"() -> (w3217:string)
                    n1773 = local read "Opj X Axis"() -> (w3222:string)
                    n1774 = Concatenate Strings("window -a OnOffGraph;\nlayer.x.type=", w3222, "; layer.x.label.numFormat = ", w3217, "; Y3 = 1; X3 = 1;", "window -a OnOffTable;\nwindow -s TV;") -> (w3220:string)
                    n1775 = call "Param_Analysis_7_24b_JW.vi"("Independant Variable"=w3225, "error in (no error)"=w3228, "Data Folder"=w3226, "Parameter String"="On/Off I-Sat:", "Parameter Name"="OnOff Ratio", "Stats Folder"=w3227) -> ("error out"=w3232:errorcluster, "Output Array"=w3230:string[][], "Variables"=w3224:T16)  [unwired: 2 in, 1 out]
                    n1776 = call "Origin_Export_7_27a_JW.vi"("Input Conditions"=w3224, "Analysis Array"=w3230, "error in (no error)"=w3232, "Parameter Worksheet Name"="[OnOffTable]On/Off Ratios", "Parameter Folder Script"="pe_cd \"OnOff-Ratio\";", "Origin.IOApplication"=w3229) -> ("error out"=w3231:errorcluster, "reference out"=w3233:refnum<k7>)  [unwired: 3 in, 1 out]
                    n1777 = call <userlib>:"OAExecute.vi"("script"=w3220, "Error IO"=w3231, "Origin.IOApplication"=w3233) -> ()  [unwired: 1 in, 3 out]
                  }
                  frame #6 {
                    n1778 = local read "X Axis Display Type"() -> (w3238:string)
                    n1779 = local read "Opj X Axis"() -> (w3243:string)
                    n1780 = call "Param_Analysis_7_24b_JW.vi"("Independant Variable"=w3246, "error in (no error)"=w3249, "Data Folder"=w3247, "Parameter String"="STS-Sat (V/decade):", "Parameter Name"="STS-Sat", "Stats Folder"=w3248) -> ("error out"=w3253:errorcluster, "Output Array"=w3251:string[][], "Variables"=w3245:T16)  [unwired: 2 in, 1 out]
                    n1781 = Concatenate Strings("window -a SGraph;\nlayer.x.type=", w3243, "; layer.x.label.numFormat = ", w3238, "; Y3 = 1; X3 = 1;", "window -a STable;\nwindow -s TV;") -> (w3241:string)
                    n1782 = call "Origin_Export_7_27a_JW.vi"("Input Conditions"=w3245, "Analysis Array"=w3251, "error in (no error)"=w3253, "Parameter Worksheet Name"="[STable]Threshold Swing", "Parameter Folder Script"="pe_cd \"STS-Sat\";", "Origin.IOApplication"=w3250) -> ("error out"=w3252:errorcluster, "reference out"=w3254:refnum<k7>)  [unwired: 3 in, 1 out]
                    n1783 = call <userlib>:"OAExecute.vi"("script"=w3241, "Error IO"=w3252, "Origin.IOApplication"=w3254) -> ()  [unwired: 1 in, 3 out]
                  }
                  frame #7 {
                    n1784 = local read "X Axis Display Type"() -> (w3259:string)
                    n1785 = local read "Opj X Axis"() -> (w3264:string)
                    n1786 = Concatenate Strings("window -a VtGraph;\nlayer.x.type=", w3264, "; layer.x.label.numFormat = ", w3259, "; Y3 = 1; X3 = 1;", "window -a VtTable;\nwindow -s TV;") -> (w3262:string)
                    n1787 = call "Param_Analysis_7_24b_JW.vi"("Independant Variable"=w3267, "error in (no error)"=w3272, "Data Folder"=w3270, "Parameter String"="Vt-Sat (V):", "Parameter Name"="Vt-Sat", "Stats Folder"=w3271) -> ("error out"=w3276:errorcluster, "Output Array"=w3274:string[][], "Variables"=w3266:T16)  [unwired: 2 in, 1 out]
                    n1788 = call "Origin_Export_7_27a_JW.vi"("Input Conditions"=w3266, "Analysis Array"=w3274, "error in (no error)"=w3276, "Parameter Worksheet Name"="[VtTable]Threshold Voltages", "Parameter Folder Script"="pe_cd \"Vt-Sat\";", "Origin.IOApplication"=w3273) -> ("error out"=w3275:errorcluster, "reference out"=w3277:refnum<k7>)  [unwired: 3 in, 1 out]
                    n1789 = call <userlib>:"OAExecute.vi"("script"=w3262, "Error IO"=w3275, "Origin.IOApplication"=w3277) -> ("Error IO Out"=w3268:errorcluster, "Origin.IOApplication"=w3269:refnum<k7>)  [unwired: 1 in, 1 out]
                  }
                }
                n1790 = Path To String(path=w3097) -> (string=w3096:string)
                n1791 = call <userlib>:"OAExecute.vi"("script"="pe_cd /; ", "Error IO"=w3092, "Origin.IOApplication"=w3091) -> ("Error IO Out"=w3098:errorcluster, "Origin.IOApplication"=w3099:refnum<k7>)  [unwired: 1 in, 1 out]
                n1792 = call <userlib>:"OASaveProject.vi"("path"=w3096, "Error IO"=w3098, "Origin.IOApplication"=w3099) -> ()  [unwired: 3 out]
              }
            }
          }
          event "Blank Button": Mouse Down {
            n1793 = event-data() -> ()  [unwired: 1 in, 7 out]
            n1794 = local read "Transfer File"() -> (w3292:path)
            n1795 = disable-structure shown="Disabled" {
              frame Disabled {
                n1796 = local read "Folder Index"() -> (w3293:dbl)
                n1797 = Decrement(x=w3293) -> (x-1=w3294:dbl)
                n1798 = local write "Folder Index"(w3294) -> ()
              }
              frame Enabled {
              }
            }
            n1799 = Strip Path(path=w3292) -> (stripped path=w3288:path, name=w3290:string)
            n1800 = Path To String(path=w3288) -> (string=w3287:string)
            n1801 = Concatenate Strings(w3287, "\\", "X_", w3290) -> (w3286:string)
            n1802 = String To Path(string=w3286) -> (path=w3285:path)
            n1803 = Move(source path=w3292, 10:w3285) -> ()  [unwired: 3 in, 3 out]
            n1804 = local write "Transfer File"(w3285) -> ()
          }
          event "Cancel Button": Mouse Down {
            (unwired) 6
            n1805 = event-data() -> ()  [unwired: 1 in, 7 out]
            n1806 = call "Simulate_Keyboard.vi"("Action"=2, "Virtual Key"=162) -> ()  [unwired: 7 in, 1 out]
          }
        }
        n1807 = Multiply(x=w523, y=10) -> (x*y=w525:sgl)
        n1808 = case shown="\"0\"" w564 {
          tunnel: w538 -> [w622 w628 w632 w634 w638 w640 w642 w644 w646 w648 w650 w652 w654 w656 w658 w660 w662 w664 w666 w668 w670 w672 w674 w676 w678 w680 w682 w684 w686 w688 w690 w692 w694 w696 w698 w700 w702 w704 w706 w708 w710 w712 w714 w716 w718 w720 w722 w724 w726 w728 w730 w732 w734 w736 w738 w740 w742 w744 w746 w748 w750 w752 w754 w756 w758 w760 w762 w764 w766 w768 w770 w772 w774 w776 w778 w780 w782 w784 w786 w788 w790 w792 w794 w796 w798 w800 w802 w804 w806 w808 w810 w812 w814 w816 w818 w820 w822 w824 w826 w828 w830 w832 w834 w836 w838]
          tunnel: [w622 w627 w631 w634 w638 w640 w642 w644 w646 w648 w650 w652 w654 w656 w658 w660 w662 w664 w666 w668 w670 w672 w674 w676 w678 w680 w682 w684 w686 w688 w690 w692 w694 w696 w698 w700 w702 w704 w706 w708 w710 w712 w714 w716 w718 w720 w722 w724 w726 w728 w730 w732 w734 w736 w738 w740 w742 w744 w746 w748 w750 w752 w754 w756 w758 w760 w762 w764 w766 w768 w770 w772 w774 w776 w778 w780 w782 w784 w786 w788 w790 w792 w794 w796 w798 w800 w802 w804 w806 w808 w810 w812 w814 w816 w818 w820 w822 w824 w826 w828 w830 w832 w834 w836 w838] -> w563
          tunnel: w539 -> [w624 w626 w630 w636 w637 w639 w641 w643 w645 w647 w649 w651 w653 w655 w657 w659 w661 w663 w665 w667 w669 w671 w673 w675 w677 w679 w681 w683 w685 w687 w689 w691 w693 w695 w697 w699 w701 w703 w705 w707 w709 w711 w713 w715 w717 w719 w721 w723 w725 w727 w729 w731 w733 w735 w737 w739 w741 w743 w745 w747 w749 w751 w753 w755 w757 w759 w761 w763 w765 w767 w769 w771 w773 w775 w777 w779 w781 w783 w785 w787 w789 w791 w793 w795 w797 w799 w801 w803 w805 w807 w809 w811 w813 w815 w817 w819 w821 w823 w825 w827 w829 w831 w833 w835 w837]
          tunnel: [w623 w626 w630 w635 w637 w639 w641 w643 w645 w647 w649 w651 w653 w655 w657 w659 w661 w663 w665 w667 w669 w671 w673 w675 w677 w679 w681 w683 w685 w687 w689 w691 w693 w695 w697 w699 w701 w703 w705 w707 w709 w711 w713 w715 w717 w719 w721 w723 w725 w727 w729 w731 w733 w735 w737 w739 w741 w743 w745 w747 w749 w751 w753 w755 w757 w759 w761 w763 w765 w767 w769 w771 w773 w775 w777 w779 w781 w783 w785 w787 w789 w791 w793 w795 w797 w799 w801 w803 w805 w807 w809 w811 w813 w815 w817 w819 w821 w823 w825 w827 w829 w831 w833 w835 w837] -> w562
          tunnel: w525 -> [w621 w625 w629 w633 _ _ _ _ _ _ _ _ _ _ _ _ _ _ _ _ _ _ _ _ _ _ _ _ _ _ _ _ _ _ _ _ _ _ _ _ _ _ _ _ _ _ _ _ _ _ _ _ _ _ _ _ _ _ _ _ _ _ _ _ _ _ _ _ _ _ _ _ _ _ _ _ _ _ _ _ _ _ _ _ _ _ _ _ _ _ _ _ _ _ _ _ _ _ _ _ _ _ _ _ _]
          frame "DOWN" {
            n1809 = Add(x=w624, y=w621) -> (x+y=w623:sgl)
          }
          frame "LEFT" {
            n1810 = Subtract(x=w628, y=w625) -> (x-y=w627:sgl)
          }
          frame "RIGHT" {
            n1811 = Add(x=w632, y=w629) -> (x+y=w631:sgl)
          }
          frame "UP" {
            n1812 = Subtract(x=w636, y=w633) -> (x-y=w635:sgl)
          }
          frame "ENTER (num pad)" {
          }
          frame "' (quote)" {
          }
          frame "END" {
          }
          frame "EQUALS" {
          }
          frame "ESCAPE" {
          }
          frame "GRAVE (`)" {
          }
          frame "HOME" {
          }
          frame "INSERT" {
          }
          frame "LBRACKET" {
          }
          frame "LCONTROL" {
          }
          frame "L ALT" {
          }
          frame "LSHIFT" {
          }
          frame "LWIN" {
          }
          frame "MINUS" {
          }
          frame "MULTIPLY" {
          }
          frame "NEXT" {
          }
          frame "NUMLOCK" {
          }
          frame "NUMPAD_0" {
          }
          frame "NUMPAD_1" {
          }
          frame "NUMPAD_2" {
          }
          frame "NUMPAD_3" {
          }
          frame "NUMPAD_4" {
          }
          frame "NUMPAD_5" {
          }
          frame "NUMPAD_6" {
          }
          frame "NUMPAD_7" {
          }
          frame "NUMPAD_8" {
          }
          frame "NUMPAD_9" {
          }
          frame "PAUSE" {
          }
          frame "PERIOD" {
          }
          frame "PRIOR (PG UP)" {
          }
          frame "RBRACKET" {
          }
          frame "RCONTROL" {
          }
          frame "RETURN" {
          }
          frame "R ALT" {
          }
          frame "RSHIFT" {
          }
          frame "RWIN" {
          }
          frame "SCROLL" {
          }
          frame "SEMICOLON" {
          }
          frame "SLASH" {
          }
          frame "SPACE" {
          }
          frame "SUBTRACT" {
          }
          frame "TAB" {
          }
          frame "DIVIDE" {
          }
          frame "DELETE" {
          }
          frame "DECIMAL" {
          }
          frame "COMMA" {
          }
          frame "CAPITAL" {
          }
          frame "BACKSLASH" {
          }
          frame "BACK" {
          }
          frame "ADD" {
          }
          frame "F15" {
          }
          frame "F14" {
          }
          frame "F13" {
          }
          frame "F12" {
          }
          frame "F11" {
          }
          frame "F10" {
          }
          frame "F9" {
          }
          frame "F8" {
          }
          frame "F7" {
          }
          frame "F6" {
          }
          frame "F5" {
          }
          frame "F4" {
          }
          frame "F3" {
          }
          frame "F2" {
          }
          frame "F1" {
          }
          frame "Z" {
          }
          frame "Y" {
          }
          frame "X" {
          }
          frame "W" {
          }
          frame "V" {
          }
          frame "U" {
          }
          frame "T" {
          }
          frame "S" {
          }
          frame "R" {
          }
          frame "Q" {
          }
          frame "P" {
          }
          frame "O" {
          }
          frame "N" {
          }
          frame "M" {
          }
          frame "L" {
          }
          frame "K" {
          }
          frame "J" {
          }
          frame "I" {
          }
          frame "H" {
          }
          frame "G" {
          }
          frame "F" {
          }
          frame "E" {
          }
          frame "D" {
          }
          frame "C" {
          }
          frame "B" {
          }
          frame "A" {
          }
          frame "9" {
          }
          frame "8" {
          }
          frame "7" {
          }
          frame "6" {
          }
          frame "5" {
          }
          frame "4" {
          }
          frame "3" {
          }
          frame "2" {
          }
          frame "1" {
          }
          frame "0" {
          }
        }
        n1813 = Bundle(w541, w540, w555, w554, 0.0) -> (w553:cluster{dbl, dbl, dbl, dbl, dbl})  [unwired: 1 in]
        n1814 = Bundle("X"=w563, "Y"=w562) -> (w557:cluster{"X":sgl, "Y":sgl})  [unwired: 1 in]
        n1815 = Divide(x=20, y=w524) -> (x/y=w527:sgl)
        n1816 = property on="Image Out" class="ImageControl"("Image Center Position"=w557) -> ()  [unwired: 2 in, 2 out]
        n1817 = call "IMAQ Convert Rectangle to ROI (Polygon)"("Rectangle"=w553) -> ("ROI Descriptor"=w551:T3)  [unwired: 7 in, 2 out]
        n1818 = Bundle("Application Font", w527, w531, w531, w531, w531, w531, TRUE, w529) -> (w533:T17)  [unwired: 1 in]
        n1819 = property on="Image Out 2" class="ImageControl"("ROI"=w551) -> ()  [unwired: 2 in, 2 out]
        n1820 = Bundle(w529, w533, w529, w529) -> (w532:T18)  [unwired: 1 in]
        n1821 = property on="Image Out" class="ImageControl"() -> ("ROI"=w516:T10)  [unwired: 2 in, 2 out]
        n1822 = Unbundle By Name(w516) -> ("Contours"=w580:T14)
        n1823 = local read "Image Out"() -> (w535:T2)
        n1824 = call "IMAQ Clear Overlay"("Image"=w535) -> ("Image Out"=w534:T2)  [unwired: 9 in, 1 out]
        n1825 = Initialize Array(0) -> (w578:i32[])  [unwired: 1 in]
        n1826 = local read "Magnification"() -> (w569:u16)
        n1827 = Array Size(array=w580) -> (size(s)=w579:i32)
        n1828 = Build Array(0.505025, 0.252522, 0.127742, 0.050345, 0.031129) -> (w570:dbl[])
        n1829 = Array Subset(array=w570, index=w569, length=1) -> (w567:dbl[])
        n1830 = property on="Image Out" class="ImageControl"() -> ("ZoomInteger"=w559:cluster{"X":i32, "Y":i32})  [unwired: 2 in, 2 out]
        n1831 = To Double Precision Float(number=w567) -> (double precision float=w566:dbl[])
        n1832 = for {
          N: w579 -> [_]
          shift-right: [w861] -> _
          shift-left: w580 -> [w861]
          shift-right: [w859] -> w565
          shift-left: w578 -> [w858]
          tunnel: w566 -> [w857]
          shift-right: [w854] -> _
          shift-left: w534 -> [w856]
          tunnel: w532 -> [w849]
          i -> [w853]
          n1833 = Index Array(array=w861, index=w853) -> (element=w870:T19)
          n1834 = Unbundle(w870) -> ("Points"=w869:i32[])  [unwired: 2 out]
          n1835 = Array To Cluster(array=w869) -> (cluster=w868:T20)
          n1836 = Unbundle(w868) -> ("Points[0]"=w848:i32, "Points[1]"=w845:i32, "Points[2]"=w860:i32, "Points[3]"=w866:i32)  [unwired: 5 out]
          n1837 = Add(x=w848, y=10) -> (x+y=w846:i32)
          n1838 = Subtract(x=w845, y=w866) -> (x-y=w865:i32)
          n1839 = Subtract(x=w848, y=w860) -> (x-y=w867:i32)
          n1840 = Square(x=w865) -> (x^2=w863:i32)
          n1841 = Square(x=w867) -> (x^2=w864:i32)
          n1842 = Add(x=w864, y=w863) -> (x+y=w862:i32)
          n1843 = Square Root(x=w862) -> (sqrt(x)=w839:dbl)
          n1844 = Multiply(x=w839, y=0.5) -> (x*y=w842:dbl)
          n1845 = Add(x=w842, y=w845) -> (x+y=w844:dbl)
          n1846 = Bundle(w846, w844) -> (w855:cluster{i32, dbl})  [unwired: 1 in]
          n1847 = Multiply(x=w839, y=w857) -> (x*y=w852:dbl[])
          n1848 = Index Array(array=w852) -> (element=w851:dbl)  [unwired: 1 in]
          n1849 = Number To Fractional String(number=w851) -> (F-format string=w850:string)  [unwired: 3 in]
          n1850 = call "IMAQ Overlay Text"("BG Color (Transparent)"=u32 0, "Text Color (black)"=u32 16448250, "Font, Size & Style"=w849, "String"=w850, "Origin"=w855, "Image"=w856) -> ("Image Out"=w854:T2)  [unwired: 4 in, 1 out]
          n1851 = Build Array (concatenate)(w858, w852) -> (w859:dbl[])
          n1852 = local write "Numeric 3"(w839) -> ()
        }
        n1853 = local write "ROI Descriptor"(w516) -> ()
        n1854 = Unbundle(w559) -> ("X"=w558:i32)  [unwired: 1 out]
        n1855 = Add Array Elements(numeric array=w565) -> (sum=w576:dbl)
        n1856 = local write "Distances"(w565) -> ()
        n1857 = local write "Total Width"(w576) -> ()
        n1858 = local write "Zoom"(w558) -> ()
        n1859 = local read "Manual-Width"() -> (w515:bool)
        n1860 = local read "Total Width"() -> (w519:dbl)
        n1861 = local read "Rec: Width"() -> (w517:dbl)
        n1862 = Not(x=w515) -> (.not. x?=w513:bool)
        n1863 = Equal To 0?(x=w519) -> (x = 0?=w514:bool)
        n1864 = Or(x=w514, y=w515) -> (x .or. y?=w518:bool)
        n1865 = And(x=w514, y=w513) -> (x .and. y?=w512:bool)
        n1866 = case shown="True" w512 {
          tunnel: w517 -> [_ w599]
          frame False {
          }
          frame True {
            n1867 = local write "New: Width"(w599) -> ()
          }
        }
        n1868 = case shown="False" w518 {
          tunnel: w519 -> [w600 _]
          frame False {
            n1869 = local write "New: Width"(w600) -> ()
          }
          frame True {
          }
        }
        n1870 = local read "Manuel-Dielectric"() -> (w441:bool)
        n1871 = local read "Rec: Dielectric (d)"() -> (w440:dbl)
        n1872 = local read "Manuel-Length"() -> (w442:bool)
        n1873 = local read "Rec: Length"() -> (w443:dbl)
        n1874 = case shown="False" w442 {
          tunnel: w443 -> [w590 _]
          frame False {
            n1875 = local write "New: Length"(w590) -> ()
          }
          frame True {
          }
        }
        n1876 = case shown="False" w441 {
          tunnel: w440 -> [w589 _]
          frame False {
            n1877 = local write "New: Dielectric"(w589) -> ()
          }
          frame True {
          }
        }
      }
    }
  }
  n1878 = Build Array("DeviceID", "Fabricator", "Deposition", "Date", "Sample", "Row", "Column", "L (um)", "W (um)", "Material", "Treatment", "TC (mM)", "Solvent", "C (%)", "ST (C)", "Drops", "Wait (s)", "RT (F)", "RH (%)", "Ramp (s)", "RPM", "Accel (RPM/s)", "Time (s)", "Mobility", "On/Off", "Vt", "S.T.S") -> (→"Transformer \nHeaders":string[])
